vi "CW-main.vi"() -> ()   [LabVIEW 2024]
doc: "Main VI for HFEPR measurements in Field domain.\nProgram uses a tab control that divides user interface in 5 pages. First (status) page is to monitor status of instruments. Second (adjustment) page is to setup individual parameters of each instrument. Third (EPR measurement) page serves for execution of measurement. Fourth (script) page serves for generation of script that can be later loaded in measurement tab. Fifth (measurement review) page is to display previous measurements. The last (about) page contains quick start info for user."
uses:
  Datatypes/Connected modules.ctl
  Datatypes/Magnet controls.ctl
  Datatypes/Servo controls.ctl
  Datatypes/THz parameters.ctl
  Datatypes/Measurement info.ctl
  Datatypes/experiment state.ctl
  Datatypes/SampleHolders.ctl
  Datatypes/Module selection.ctl
  Subsystem modules/Lock-in module/ctl/MFLI parameters.ctl
  Subsystem modules/Temperature control module/ctl/Set temperature.ctl
  Datatypes/script polymorh line.ctl
  Datatypes/Instr Info.ctl
  Subsystem modules/Magnet module/ctl/RampingOutput.ctl
  Datatypes/Single servo status.ctl
  Subsystem modules/Servo drive module/ctl/Axis names.ctl
  Datatypes/Measurement type.ctl
  Datatypes/Rotator controls.ctl
  Subsystem modules/Sample rotator/ctl/Motion Properties.ctl
  Subsystem modules/Sample rotator/ctl/Positoin to set.ctl
  Subsystem modules/Source meter/ctls/SMU settings.ctl
  Datatypes/TopStates.ctl
  Datatypes/XY measurement graph data.ctl
  Datatypes/Measurement mode.ctl
  <vilib>/Utility/sysdir.llb/System Directory Type.ctl
  Subsystem modules/Magnet module/ctl/MSG to magnet.ctl
  Subsystem modules/Magnet module/ctl/Magnet Orders.ctl
  Subsystem modules/Magnet module/ctl/SetField data.ctl
  Subsystem modules/Magnet module/ctl/Magnet mode public.ctl
  Subsystem modules/Servo drive module/ctl/Servo MSG.ctl
  Subsystem modules/Servo drive module/ctl/Servo commands.ctl
  Subsystem modules/Sample rotator/ctl/MSG to Rotator.ctl
  Subsystem modules/Sample rotator/ctl/Rotator commands.ctl
  Subsystem modules/THz module/ctl/THz Message for module.ctl
  Subsystem modules/THz module/ctl/THz commands enum.ctl
  Subsystem modules/THz module/ctl/THz sweep parameters.ctl
  Subsystem modules/Lock-in module/ctl/MFLI_message for module.ctl
  Subsystem modules/Lock-in module/ctl/MFLI_command enum.ctl
  Subsystem modules/Lock-in module/ctl/MFLI_parameter and value.ctl
  Subsystem modules/Lock-in module/ctl/MFLI_node.ctl
  Subsystem modules/Temperature control module/ctl/MSG for VTI.ctl
  Subsystem modules/Temperature control module/ctl/TC commands.ctl
  Subsystem modules/Temperature control module/ctl/Set point.ctl
  Subsystem modules/Source meter/ctls/MSG to SMU.ctl
  Subsystem modules/Source meter/ctls/SMU Commands.ctl
  Subsystem modules/THz module/ctl/THz MW generator constants.ctl
  Subsystem modules/Magnet module/ctl/TM Revision.ctl
  Subsystem modules/Magnet module/ctl/Overall status.ctl
  Subsystem modules/Magnet module/ctl/Actual magnet state.ctl
  Subsystem modules/Magnet module/ctl/Magnet mode.ctl
  Subsystem modules/Magnet module/ctl/Cryostat temperature sensors.ctl
  Subsystem modules/Power monitor/PwrM status.ctl
  Subsystem modules/Source meter/ctls/SMU status.ctl
  Subsystem modules/Lock-in module/ctl/ACQ info.ctl
  <instrlib>/Zurich Instruments LabOne/Public/Data/ziTypeDemodSampleSingle.ctl
  <instrlib>/Zurich Instruments LabOne/Public/ziTypeHandle.ctl
  Subsystem modules/Temperature control module/ctl/TC sensors.ctl
  Subsystem modules/Servo drive module/ctl/Servo state.ctl
  Subsystem modules/Servo drive module/ctl/Servo variables.ctl
  Subsystem modules/Servo drive module/ctl/Servo constants.ctl
  Subsystem modules/Servo drive module/ctl/Status variable change.ctl
  Subsystem modules/Sample rotator/ctl/Rotator all.ctl
  Subsystem modules/Sample rotator/ctl/Axis status.ctl
  <vilib>/Utility/error.llb/Trim Whitespace One-Sided.vi
  Subsystem modules/Messenger service/MessengerLib.lvlib
  Subsystem modules/Magnet module/Magnet module.lvlib
  Subsystem modules/Servo drive module/Servo drive module.lvlib
  Subsystem modules/THz module/THz source modeule.lvlib
  Subsystem modules/Lock-in module/Lock-in module.lvlib
  Subsystem modules/Sample rotator/SampleRotator.lvlib
  <instrlib>/Zurich Instruments LabOne/Zurich Instruments LabOne.lvlib
  Subsystem modules/Temperature control module/Temperature controller.lvlib
  <userlib>/_OpenG.lib/variantconfig/variantconfig.llb/openg_variant_configuration_file.lvlib
  <vilib>/Utility/config.llb/NI_LVConfig.lvlib
  Subsystem modules/Source meter/Source meter.lvlib
  Subsystem modules/Power monitor/Power monitor.lvlib
panel:
  out "Instr status":T1 caption="Connected\ninstuments"
  out "Controls referencies":T2
  out "Tmp [K]":T3
  out "Busy":bool
  in  "Stop":bool
  out "Results":T5(array[cluster])
  out "Magnetic\nfield state":bool
  out "data time":timestamp
  out "New data":bool
  out "Data":dbl[](array[numeric])
  out "Instr control refs":refnum<vi>[](array[refnum])
  out "meas results":refnum<file>
  out "Tmp reched time":dbl format="%<%H:%M:%S>T"
  out "VTI tmp reached":bool
  out "Running experiment":bool
  out "Temperature log ref":refnum<file>
  out "round execution\ntime [ms]":u32
  out "loggersRef":refnum<file>
  in  "Tab Control":T6(tab)
  out "Drift[K/s]":dbl[](array[numeric])
  in  "Log folder":path=path "C:/HFEPR logs"
  in  "Disconnect":bool
  in  "Select module":T7
  out "Logger":string[](array[string])
  in  "Re-connect instruments":bool
  in  "System config file path":path=path "C:/Programs/Debug/HFEPR spectrometer SW 2024/Multi-HFEPR app/SystemData/config.ini"
  out "Instr info":T8 {"PwrMonitor"."Last update" format="%<%H:%M:%S>T"; "VTI"."Last update" format="%<%H:%M:%S>T"; "PMD"."Last update" format="%<%H:%M:%S>T"; "SMU"."Last update" format="%<%H:%M:%S>T"; "Servo"."Last update" format="%<%H:%M:%S>T"; "Rotator"."Actuator" items=["Linear", "Roatator", "Goniometer"]; "Rotator"."Name" items=["ANC350res", "ANC350num", "ANC350fps", "Unknown"]; "Rotator"."Last update" format="%<%H:%M:%S>T"; "THz"."Last update" format="%<%H:%M:%S>T"; "MFLI"."Last update" format="%<%H:%M:%S>T"; "Magnet"."Last update" format="%<%H:%M:%S>T"}
  in  "Use previous settings":bool=TRUE
  out "Temperature monitor":T12(graph)
  in  "Debug mode?":bool=TRUE
  in  "SMU controls":T14={"Apply"=FALSE, "Measurement settings"={"Source Mode "=1, "Source Level"=0.1, "Source Limit"=0.21, "Measure Function"=0, "Remote sense"=TRUE, "Clear buffer?"=FALSE, "Beep"=TRUE, "High Capacity"=TRUE, "Terminals"=1, "PLCs"=4.0, "Fast measurement"=TRUE}, "Value"=0.1006, "Stop"=FALSE, "Record"=FALSE, "B[T]"=0.0, "Refresh"=FALSE} {"Value" format="%#_3e"; "Measurement settings"."Measure Function" items=["Volts", "Current", "Auto Resistance", "Manual Resistance", "Digitize Voltage", "Digitize Current"]; "Measurement settings"."Source Level" max=0.3; "Measurement settings"."Source Mode" items=["Voltage", "Current"]; "Measurement settings"."Terminals" items=["Front", "Rear"]}
  in  "Rotator controls":T15={"Motion properties"={"Frequency [Hz]"=1000.0, "Precision [m°]"=100.0, "DC voltage [V]"=0.0, "Amplitude [V]"=25.0}, "Set position"={"Relative?"=FALSE, "Position [°]"=0.0, "Safe to move?"=FALSE}, "Actual angle[°]"=0.0, "Rot set properties btn"=FALSE, "Rot set position btn"=FALSE, "Stop btn"=FALSE, "EoF"=FALSE, "EoB"=FALSE, "Error"=FALSE} {"Motion properties"."Amplitude [V]" min=0.0 max=60.0; "Motion properties"."DC voltage [V]" min=0.0 max=60.0; "Motion properties"."Precision [m°]" min=1.0 max=1000.0; "Motion properties"."Frequency [Hz]" min=10.0 max=5000.0 step=1.0}
  in  "Password":string
  in  "VTI control":T18={"VTI space [K]"=1.0, "Sample [K]"=0.0, "Heater3 [K]"=1.8, "Heater4 [K]"=1.8, "Out 1 [%]"=0.0, "Out 2 [%]"=0.0, "Range out 1"=0} {"Range out 1" items=["Off", "Range 1 (On)", "Range 2", "Range 3", "Range 4", "Range 5"]; "Heater4 [K]" min=1.8 max=300.0; "Heater3 [K]" min=1.8 max=300.0}
  in  "Acquisition controls":T21={"ACQ parameters"={"Filter order"=7.0, "Filter tau [ms]"=10.0, "F_Mod [kHz]"=1.0, "Amp_Mod [mV]"=10.0, "Enable output"=0, "Phase [°]"=0.0}, "ACQ shot btn"=FALSE, "Modulation [A]"=0.0, "In50"=FALSE, "Out50"=FALSE, "DemEn"=FALSE, "Actual [G]"=0.0, "Sample holder"=enum."Simple", "Desired [G]"=0.0, "Adj mod"=FALSE, "Auto-modulation"=TRUE, "Autorange"=FALSE, "AuxIn0 [V]"=0.0, "AuxIn1 [V]"=0.0} {"AuxIn1 [V]" format="%#_3g"; "AuxIn0 [V]" format="%#_3g"; "Desired [G]" format="%.1g"; "ACQ parameters"."Enable output" items=["Disable", "Enable"]; "ACQ parameters"."Amp_Mod [mV]" min=0.0 max=10000.0; "ACQ parameters"."F_Mod [kHz]" min=0.1 max=500.0; "ACQ parameters"."Filter order" min=1.0 max=9.0 step=1.0; "ACQ parameters"."Filter tau [ms]" min=0.0 max=1000.0}
  in  "THz control":T22={"AMC"=9, "Multip"=1, "Base frequency [GHz]"=82.0, "End frequency [GHz]"=0.0, "Im frequency [MHz]"=1500.0, "Sweep up [ms]"=0.0, "Reset trigger?"=FALSE} {"Multip" items=["1"=1, "2"=2, "3"=3, "4"=4, "6"=6, "8"=8, "9"=9]; "AMC" items=["9"=9, "12"=12]; "End frequency [GHz]" min=0.09 max=126.0; "Base frequency [GHz]" min=0.09 max=126.0 step=0.001 format="%.2g"}
  in  "Servo controls":T23={"Y left"=FALSE, "Y right"=FALSE, "X backward"=FALSE, "X forward"=FALSE, "Zdown"=FALSE, "Zup"=FALSE, "Step\n[mm]"=5.0, "QO table"={"ZLdown"=FALSE, "ZLup"=FALSE, "ZRup"=FALSE, "ZRdown"=FALSE, "ZMdown"=FALSE, "ZMup"=FALSE}, "X"=0.0, "Y"=0.0, "ZL"=0.0, "ZR"=0.0, "ZM"=0.0, "Measure Position btn"=FALSE, "Eject position btn"=FALSE, "Stop servo btn"=FALSE, "Save position btn"=FALSE} {"Step\n[mm]" min=0.0 max=10.0 step=0.25}
  in  "Magnet controls":T24 {"Actual\noutput [T]" scale=0.0..16.0; "Actual\nfield [T]" scale=0.0..16.0; "Desired\nramp [mT/s]" max=7.544966; "Set Field [T]" max=16.0}
  out "lookup":cluster{"X (Vrms)":dbl, "Y (Vrms)":dbl}(graph) caption="Waveform Chart - Dark"
  in  "Create folder with date":bool
  in  "Operator":string
  in  "Hide script":bool
  in  "Save also backup":bool
  in  "Main data folder":path
  in  "Global comment":string
  in  "Sample name":string="Unknown"
  in  "Run script btn":bool
  in  "Direct stop meas. btn":bool
  out "Infobar":T25 {"Started" format="%<%H:%M:%S>T"; "Remains" format="%<%H:%M:%S>t"}
  out "Spectrum":cluster{dbl[], dbl[]}[](graph) caption="Live spectrum"
  in  "Paste from Editor":bool
  out "Actual measurement":T27={"Start"=nan, "Start Caption"="Start [T]", "End"=0.0, "End Caption"="End [T]", "Sweep"=0.0, "Sweep caption"="Rate [mT/s]", "Constant"=0.0, "Constant caption"="Freq [GHz]", "Mod_F [kHz]"=0.0, "Mod_A [G]"=0.0, "Tau [ms]"=0.0, "Angle [°]"=0.0, "Tmp [K]"=50.0, "Wait [min]"=0.0, "Carousel"=-1, "Comment"="", "Auto-mod"=TRUE, "Execute"=FALSE} {"Carousel" items=["0", "1", "2", "3", "4", "5", "6"]; "Angle [°]" min=0.0 max=350.0; "Tau [ms]" min=0.0 max=100.0; "Wait [min]" min=0.0 max=350.0; "Tmp [K]" min=0.0 max=3000.0; "Mod_A [G]" min=0.1 max=150.0; "Mod_F [kHz]" min=0.1 max=150.0}
  in  "Script Array":T27[](array[typedef]) {"Carousel" items=["0", "1", "2", "3", "4", "5", "6"]; "Angle [°]" min=-1.0 max=330.0; "Tau [ms]" min=0.002 max=10000.0; "Wait [min]" min=0.0 max=3000.0; "Tmp [K]" min=0.0 max=350.0; "Mod_A [G]" min=0.0 max=100.0; "Mod_F [kHz]" min=0.1 max=150.0}
  in  "Generator options":T28={"Tmp step [K]"=0.0, "Angle step [°]"=0.0, "Freq step [GHz]"=0.0, "Append"=TRUE, "Iterate"=0}
  in  "Clear script btn":bool caption="Clear all script"
  in  "Set as adj tab btn":bool caption="Apply settings from\nadjustment tab"
  in  "Prototype line":T27={"Start"=0.0, "Start Caption"="Start [T]", "End"=0.0, "End Caption"="End [T]", "Sweep"=3.0, "Sweep caption"="Rate [mT/s]", "Constant"=210.0, "Constant caption"="Freq [GHz]", "Mod_F [kHz]"=69.1, "Mod_A [G]"=2.0, "Tau [ms]"=100.0, "Angle [°]"=-1.0, "Tmp [K]"=2.0, "Wait [min]"=0.1, "Carousel"=0, "Comment"="No comment", "Auto-mod"=TRUE, "Execute"=FALSE} {"Carousel" items=["0", "1", "2", "3", "4", "5", "6"]; "Angle [°]" min=-1.0 max=330.0; "Tau [ms]" min=0.002 max=10000.0; "Wait [min]" min=0.0 max=3000.0; "Tmp [K]" min=0.0 max=350.0; "Mod_A [G]" min=0.0 max=100.0; "Mod_F [kHz]" min=0.1 max=150.0}
  in  "Paste from meeasurrement":bool
  in  "Save script file btn":bool
  in  "Generate Script btn":bool caption="Generate Script"
  in  "Edited script":T27[](array[typedef]) caption="Script file name:" {"Carousel" items=["0", "1", "2", "3", "4", "5", "6"]; "Angle [°]" min=-1.0 max=330.0; "Tau [ms]" min=0.002 max=10000.0; "Wait [min]" min=0.0 max=3000.0; "Tmp [K]" min=0.0 max=350.0; "Mod_A [G]" min=0.0 max=100.0; "Mod_F [kHz]" min=0.1 max=150.0}
  in  "Remove from script btn":bool
  in  "Load script btn":bool
  in  "Select\nline":i32 min=-8 max=7
  in  "Save data btn":bool
  in  "Shift data btn":bool
  in  "Edit Channel":bool
  in  "Amlitude shift [-]":dbl
  in  "From point [T]":dbl
  out "Header":string[](array[string])
  out "Review Graph":cluster{"Array":dbl[], "Array":dbl[]}[](graph) caption="Header"
  in  "Open measurement":bool
  in  "Data file to show":u16(ring) items=["Empty", "Empty", "Empty", "Empty", "Empty", "Empty", "Empty", "Empty", "Empty", "Empty"]
  in  "Quick guide":T29(tab)
  # "Status part"
  # "Action part"
  # "stop after this line button"
  # "Option 1:\nchoice primary and secondary sweep\n\nOption 2:\nChoice measurement mode, and appropriate cluster will apear. Other clusters wil be hidden.\n\n\nOption 3:\nChoice measurement mode.\nInternal parts of single cluster will (dis)apear if needed.\n\nNote:\nPosibility to do an orientation/temperature deppendency."
  # "Tmp [K]"
  # "Position [mm]"
  # "Z"
  # "X/Y"
  # "This software was developed for HFEPR spectrometer in 2019 (2020) at CEITEC BUT by members of MOTES research group.\n\nQuick guide:\n1) Re-connect to all instruments.\n2) Check if necessary instruments are ready. (At least VTI, VDI, Lock-In, and Magnet has to work)\n3) Go to Adjustment tab and set up Lock-in parameters as well as VDI multipiers.\n4) Go to EPR measurement tab, select folder path, fill the sample description.\n5) Fill at least 1 line of the script and press Run script button.\n\n6) In case of a bug please report this to software developer or make a note into developement diary loaceted at:\n    RG-1-12/Instriments/HFEPR spectrometer/Software developement.\n\nLast update: 07.02. 2020 - Script editor is working, measurement review not yet.\n\nSpecial thanks to: Luke Skywalker, my mom, Tonda's mom, Pilsner, God, Oleksi, Vinicius, Petr from parallel universe.\n\n \nTODO: Invisible controls: referencies for: adjustment controls, meas results, loggerRef,"
  # "1.\tSelect module for subsystem, which is ready to operate. For CW measurements it is necessary to use subsystems: Magnet, VTI,\n THz sources and data acquisition (MFLI).\n2.\tClick on (Re)Connect button. Repeat for all subsystems that are ready and needed.\n3.\tWhen VTI and Magnet subsystems are connected, readings from temperature monitor and controller are displayed in graph.\n4.\tSuccessful connection to subsystem is indicated here.\n5.\tEvents on instruments are reported in this indicator.\n6.\tIf everything is OK, user may continue to another tab."
  # "1.\tFor CW experiments, magnet has to be in  ramping mode. (Magnet can be then pre-set to a start field.)\n2.\tCorrect multiplication factor need to be set manually by user.\n3.\tIntermediate frequency need to be set in in a middle of the range of band pass filters. \n4.\tTemperature of VTI can be also pre-set, while other settings are done (2 - 325 K).\n5.\tPosition of table in X axis should be about 900 mm. If table is not in measurement position, and there is no object in way, user can click on button Measure.\n6.\tIn control cluster for MFLI it is needed to enable output and set reasonable frequency and amplitude of modulation. After that click on Auto range button.\n7.\tIn case when sample rotator is used, user can check if rotator works correctly by setting desired position and press Go button.\n8.\tIn case when field sensor is used, it is required to setup current source, 100 mA, measure voltage, remote sense, rear terminals and press Apply button.\n9.\tIf series of measurement is going to be done, it is recommended to first setup measurement script in a script editor."
  # "1.\tLoad script from the Script editor tab. (overwrites current script in this tab)\n2.\tModify script if needed.\n3.\tSelect main folder, where data will be stored.\n4.\tFill name of a sample and operator that will be included in a file name.\n5.\tIf checked, save data in subfolder.\n6.\tTextbox for user to add any comment in header of data file.\n7.\tStart sequence of measurements in the script.\n8.\tContain brief information about measurement process.\n9.\tDisplays a raw spectrum.\n10.\tStop whole sequence.\n11.\tA standard graph tools."
  # "1.\tLoad actual settings of instruments and apply them to a prototype line.\n2.\tModify prototype line if needed.\n3.\tSet step for one (or more) parameter, and number of iterations.\n4.\tIf checked, append to a current scrip; else, overwrites.\n5.\tSave current script into text file (structured as configuration file) to load it later.\n6.\tModify generated script or manually fill a next line."
  # "1.\tLoad data from a file.\n2.\tRing for switching to previously loaded data.\n3.\tStandard graph tools (zoom, cursor).\n4.\tFeature to apply a simple data correction."
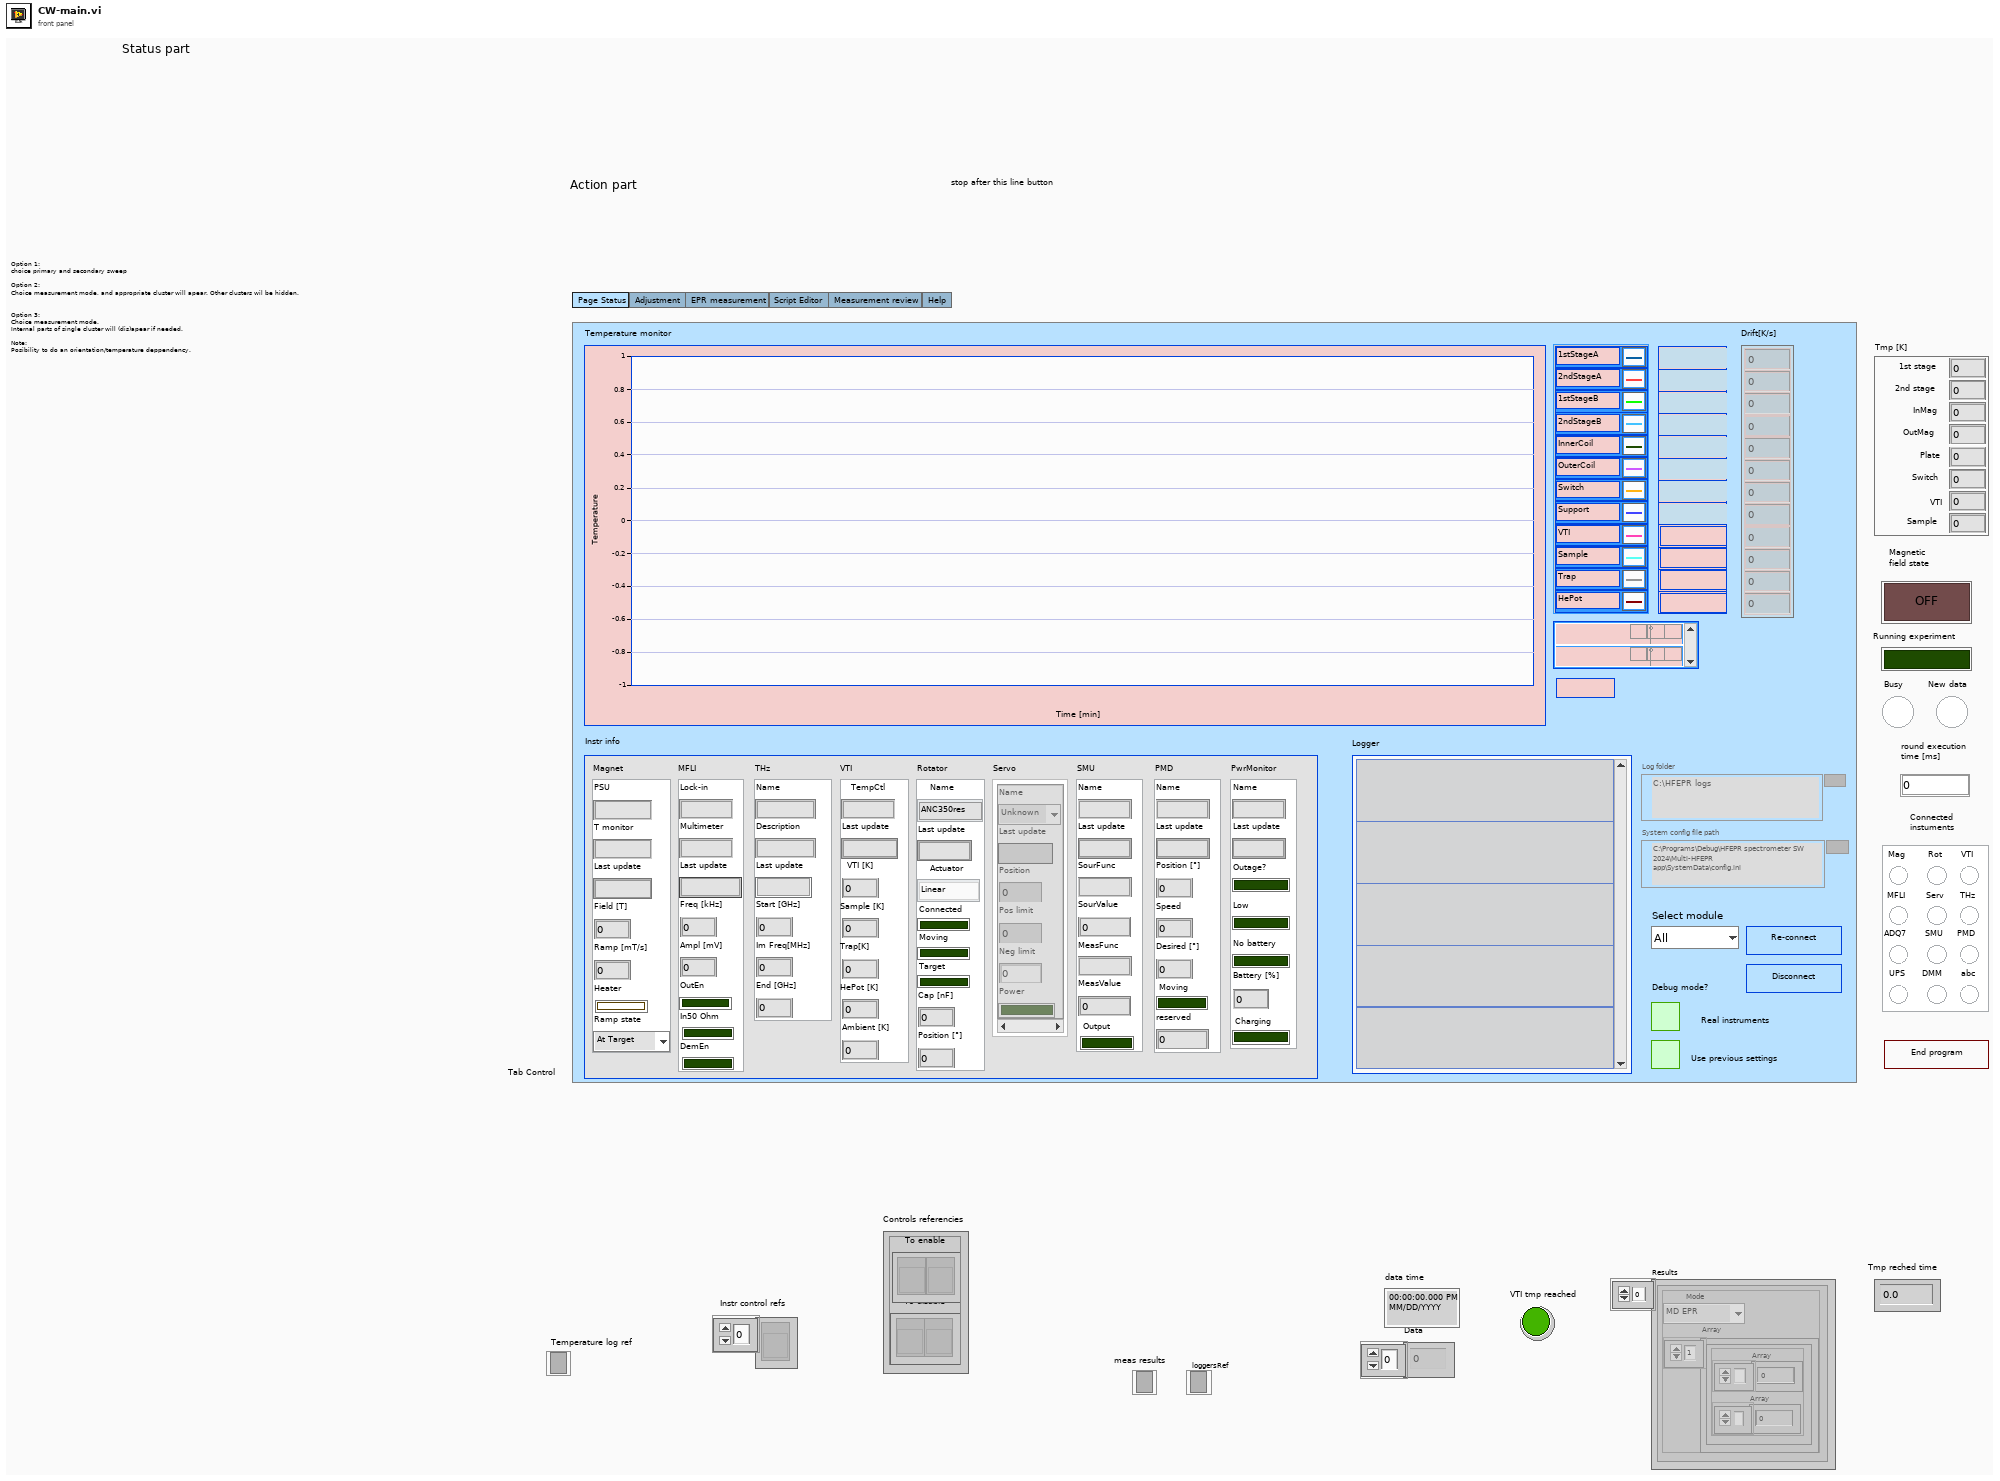
[diagram p1: front panel]
types:
  T1 = typedef "Connected modules.ctl" = cluster{"Mag":bool, "Rot":bool, "VTI":bool, "MFLI":bool, "Serv":bool, "THz":bool, "ADQ7":bool, "SMU":bool, "PMD":bool, "UPS":bool, "DMM":bool, "abc":bool}
  T2 = cluster{"To disable":refnum<vi>[], "To enable":refnum<vi>[]}
  T3 = cluster{"1st stage":dbl, "2nd stage":dbl, "InMag":dbl, "OutMag":dbl, "Plate":dbl, "Switch":dbl, "VTI":dbl, "Sample":dbl}
  T4 = typedef "Measurement type.ctl" = enum16{"MD EPR", "FD EPR"}
  T5 = cluster{"Mode":T4, "Array":cluster{"Array":dbl[], "Array":dbl[]}[]}[]
  T6 = enum32{"Page Status", "Adjustment", "EPR measurement", "Script Editor", "Measurement review", "Help"}
  T7 = typedef "Module selection.ctl" = enum16{"All", "None", "ACQ", "THz", "MAG", "SERV", "ROT", "VTI", "SMU", "ADQ7", "PMD"}
  T8 = typedef "Instr Info.ctl" = cluster{"Magnet":cluster{"PSU":string, "T monitor":string, "Last update":timestamp, "Field [T]":dbl, "Ramp [mT/s]":dbl, "Heater":bool, "Ramp state":T9}, "MFLI":cluster{"Lock-in":string, "Multimeter":string, "Last update":timestamp, "Freq [kHz]":dbl, "Ampl [mV]":dbl, "OutEn":bool, "In50 Ohm":bool, "DemEn":bool}, "THz":cluster{"Name":string, "Description":string, "Last update":timestamp, "Start [GHz]":dbl, "Im Freq[MHz]":dbl, "End [GHz]":dbl}, "VTI":cluster{"TempCtl":string, "Last update":timestamp, "VTI [K]":dbl, "Sample [K]":dbl, "Trap[K]":dbl, "HePot [K]":dbl, "Ambient [K]":dbl}, "Rotator":cluster{"Name":u16, "Last update":timestamp, "Actuator":u16, "Connected":bool, "Moving":bool, "Target":bool, "Cap [nF]":dbl, "Position [°]":dbl}, "Servo":T10[], "SMU":cluster{"Name":string, "Last update":timestamp, "SourFunc":string, "SourValue":dbl, "MeasFunc":string, "MeasValue":dbl, "Output":bool}, "PMD":cluster{"Name":string, "Last update":timestamp, "Position [°]":dbl, "Speed":dbl, "Desired [°]":dbl, "Moving":bool, "reserved":dbl}, "PwrMonitor":cluster{"Name":string, "Last update":timestamp, "Outage?":bool, "Low":bool, "No battery":bool, "Battery [%]":u8, "Charging":bool}}
  T9 = typedef "Magnet module.lvlib/RampingOutput.ctl" = enum16{"At Target", "Go up", "Go down"}
  T10 = typedef "Single servo status.ctl" = cluster{"Name":T11, "Last update":timestamp, "Position":dbl, "Pos limit":dbl, "Neg limit":dbl, "Power":bool}
  T11 = typedef "Servo drive module.lvlib/Axis names.ctl" = enum16{"Unknown", "AxisX", "AxisY", "AxisZ_left", "AxisZ_middle", "AxisZ_right"}
  T12 = cluster{"[0]":dbl, "[1]":dbl, "[2]":dbl, "[3]":dbl, "[4]":dbl, "[5]":dbl, "[6]":dbl, "[7]":dbl, "[8]":dbl, "[9]":dbl, "[10]":dbl, "[11]":dbl}
  T13 = typedef "SMU settings.ctl" = cluster{"Source Mode ":u16, "Source Level":dbl, "Source Limit":dbl, "Measure Function":u16, "Remote sense":bool, "Clear buffer?":bool, "Beep":bool, "High Capacity":bool, "Terminals":u16, "PLCs":dbl, "Fast measurement":bool}
  T14 = cluster{"Apply":bool, "Measurement settings":T13, "Value":dbl, "Stop":bool, "Record":bool, "B[T]":dbl, "Refresh":bool}
  T15 = typedef "Rotator controls.ctl" = cluster{"Motion properties":T16, "Set position":T17, "Actual angle[°]":dbl, "Rot set properties btn":bool, "Rot set position btn":bool, "Stop btn":bool, "EoF":bool, "EoB":bool, "Error":bool}
  T16 = typedef "Motion Properties.ctl" = cluster{"Frequency [Hz]":dbl, "Precision [m°]":dbl, "DC voltage [V]":dbl, "Amplitude [V]":dbl}
  T17 = typedef "Positoin to set.ctl" = cluster{"Relative?":bool, "Position [°]":dbl, "Safe to move?":bool}
  T18 = typedef "Temperature controller.lvlib/Set temperature.ctl" = cluster{"VTI space [K]":dbl, "Sample [K]":dbl, "Heater3 [K]":dbl, "Heater4 [K]":dbl, "Out 1 [%]":dbl, "Out 2 [%]":dbl, "Range out 1":u16}
  T19 = typedef "Lock-in module.lvlib/MFLI parameters.ctl" = cluster{"Filter order":dbl, "Filter tau [ms]":dbl, "F_Mod [kHz]":dbl, "Amp_Mod [mV]":dbl, "Enable output":u16, "Phase [°]":dbl}
  T20 = typedef "SampleHolders.ctl" = enum16{"Simple", "Carousel", "Chip", "Rotator", "Liquid"}
  T21 = cluster{"ACQ parameters":T19, "ACQ shot btn":bool, "Modulation [A]":dbl, "In50":bool, "Out50":bool, "DemEn":bool, "Actual [G]":dbl, "Sample holder":T20, "Desired [G]":dbl, "Adj mod":bool, "Auto-modulation":bool, "Autorange":bool, "AuxIn0 [V]":dbl, "AuxIn1 [V]":dbl}
  T22 = typedef "THz parameters.ctl" = cluster{"AMC":u16, "Multip":u16, "Base frequency [GHz]":dbl, "End frequency [GHz]":dbl, "Im frequency [MHz]":dbl, "Sweep up [ms]":dbl, "Reset trigger?":bool}
  T23 = typedef "Servo controls.ctl" = cluster{"Y left":bool, "Y right":bool, "X backward":bool, "X forward":bool, "Zdown":bool, "Zup":bool, "Step\n[mm]":dbl, "QO table":cluster{"ZLdown":bool, "ZLup":bool, "ZRup":bool, "ZRdown":bool, "ZMdown":bool, "ZMup":bool}, "X":dbl, "Y":dbl, "ZL":dbl, "ZR":dbl, "ZM":dbl, "Measure Position btn":bool, "Eject position btn":bool, "Stop servo btn":bool, "Save position btn":bool}
  T24 = typedef "Magnet controls.ctl" = cluster{"Set Field [T]":dbl, "Desired\nramp [mT/s]":dbl, "Custom\nramp":bool, "Mode switch":bool, "Pause ramp":bool, "Actual\nfield [T]":dbl, "Actual\noutput [T]":dbl, "Equalize":bool, "Discharge":bool, "Switch tmp [K]":dbl, "Direction":bool}
  T25 = typedef "Measurement info.ctl" = cluster{"Remains":dbl, "T_sample [K]":dbl, "Last log":string, "Experiment state":T26, "Field [T]":dbl, "Sample holder":T20, "Started":timestamp}
  T26 = typedef "experiment state.ctl" = enum16{"Setup", "Preparation", "Stabilization", "Begin", "Acquisition", "Save"}
  T27 = typedef "script polymorh line.ctl" = cluster{"Start":dbl, "Start Caption":string, "End":dbl, "End Caption":string, "Sweep":dbl, "Sweep caption":string, "Constant":dbl, "Constant caption":string, "Mod_F [kHz]":dbl, "Mod_A [G]":dbl, "Tau [ms]":dbl, "Angle [°]":dbl, "Tmp [K]":dbl, "Wait [min]":dbl, "Carousel":i8, "Comment":string, "Auto-mod":bool, "Execute":bool}
  T28 = cluster{"Tmp step [K]":dbl, "Angle step [°]":dbl, "Freq step [GHz]":dbl, "Append":bool, "Iterate":u16}
  T29 = enum32{"Status", "Adjustment", "Measurement", "Script", "Viewer"}
  T30 = typedef "TopStates.ctl" = enum16{"Initialize GUI", "Wait for Event", "Check message", "Check measurement", "Stop", "Restart"}
  T31 = typedef "MessengerLib.lvlib/Messenger referencies.ctl" = cluster{"TOP":refnum<queue>, "Instr_M":refnum<queue>, "Field_C":refnum<queue>, "Tmp_M":refnum<queue>, "Tmp_C":refnum<queue>, "Table_C":refnum<queue>, "MW_C":refnum<queue>, "Data_Aq":refnum<queue>, "Mod_M":refnum<queue>, "Field_M":refnum<queue>, "Pwr_M":refnum<queue>, "Angle_C":refnum<queue>, "Sample_C":refnum<queue>, "Reserved":refnum<queue>}
  T32 = typedef "XY measurement graph data.ctl" = cluster{"Mode":T33, "Array":cluster{"Array":dbl[], "Array":dbl[]}[]}
  T33 = typedef "Measurement mode.ctl" = enum16{"MD EPR", "FD EPR", "EDMR", "EPR MAP"}
  T34 = enum8{"Enabled", "Disabled", "Disabled and Grayed Out"}
  T35 = typedef "Magnet module.lvlib/Magnet mode public.ctl" = enum16{"Persistant", "Ramping"}
  T36 = typedef "Magnet module.lvlib/SetField data.ctl" = cluster{"Field [T]":dbl, "Ramp [T/s]":dbl, "Custom Ramp?":bool, "Mode":T35}
  T37 = typedef "Magnet module.lvlib/Magnet Orders.ctl" = enum16{"Ignore", "Connect", "Update", "Switch mode", "Set field", "Stop ramping", "Equalize output", "Zero output", "Flip polarity", "Blackout", "Set timer", "Eval temperatures", "Disconnect"}
  T38 = typedef "Magnet module.lvlib/MSG to magnet.ctl" = cluster{"Order":T37, "Data":variant}
  T39 = typedef "Servo drive module.lvlib/Servo commands.ctl" = enum16{"Initialize", "Update", "Move by", "Move to", "Stop", "Ignore", "Disconnect", "End"}
  T40 = typedef "Servo drive module.lvlib/Servo MSG.ctl" = cluster{"Command":T39, "Data":variant}
  T41 = typedef "SampleRotator.lvlib/MSG to Rotator.ctl" = cluster{"Command":T42, "Data":variant}
  T42 = typedef "SampleRotator.lvlib/Rotator commands.ctl" = enum16{"Ignore", "Initialize", "Update", "Set parameters", "Stop movement", "Set position", "Disconnect", "End"}
  T43 = typedef "THz source modeule.lvlib/THz commands enum.ctl" = enum16{"Ignore", "Connect", "Update", "Set parameters", "Disconnect", "End"}
  T44 = typedef "THz source modeule.lvlib/THz sweep parameters.ctl" = cluster{"Start [GHz]":dbl, "End [GHz] ":dbl, "Sweep up\ntime [ms]":dbl, "Sweep down\ntime [ms]":dbl, "Intermidiate [MHz]":dbl, "Reset trigger":bool}
  T45 = typedef "THz source modeule.lvlib/THz Message for module.ctl" = cluster{"Command":T43, "Data":variant}
  T46 = typedef "Lock-in module.lvlib/MFLI_parameter and value.ctl" = cluster{"parameter":T47, "value":dbl}
  T47 = typedef "Lock-in module.lvlib/MFLI_node.ctl" = enum16{"None", "filter_order [-]", "filter_constant [ms]", "in_diff", "in_autorange", "in_imp50", "in_AC", "osc_freq [kHz]", "out_ampl [V]", "out_autorange", "out_imp50", "enable output", "enamble ampl", "scope_enable", "scope_rate", "scope_len", "scope_trigEn", "AuxOut_amplify", "Phase_deg", "AuxOut_select"}
  T48 = typedef "Lock-in module.lvlib/MFLI_command enum.ctl" = enum16{"Initialize", "Update", "Set parameters", "Set module", "Set individual parameters", "Get point", "Get array", "Disconnect", "End", "Ignore"}
  T49 = typedef "Lock-in module.lvlib/MFLI_message for module.ctl" = cluster{"Command":T48, "Data":variant}
  T50 = typedef "Temperature controller.lvlib/Set point.ctl" = cluster{"Heater":string, "Tmp [K]":dbl}
  T51 = typedef "Temperature controller.lvlib/TC commands.ctl" = enum16{"Initialize", "Update", "Stop tmp change", "Set temperature", "Set point", "Disconnect", "End", "Ignore"}
  T52 = typedef "Temperature controller.lvlib/MSG for VTI.ctl" = cluster{"Command":T51, "Data":variant}
  T53 = typedef "Source meter.lvlib/MSG to SMU.ctl" = cluster{"Command":T54, "Data":variant}
  T54 = typedef "Source meter.lvlib/SMU Commands.ctl" = enum16{"Ignore", "Connect", "Update", "Set measurement", "Start measurement", "Get actual results", "Stop measurement", "Disconnect", "End"}
  T55 = cluster{"min synth f":dbl, "max synth f":dbl, "Ramp limits [mT/s]":dbl[], "Field ranges [T]":dbl[]}
  T56 = cluster{"Mode":T4, "Array":cluster{"Array":dbl[], "Array":dbl[]}[]}
  T57 = typedef "THz source modeule.lvlib/THz MW generator constants.ctl" = cluster{"Lower limit [GHz]":dbl, "Upper limit [GHz]":dbl, "Device name":string, "Connection":string, "Description":string, "Connected":bool, "Last settings":string, "Operation mode":enum16{"Disabled", "CW", "Arbitrary", "Sweep"}, "Enable ch 1":bool, "Enable ch 2":bool}
  T58 = typedef "Magnet module.lvlib/TM Revision.ctl" = cluster{"Instr Serial Number":string, "Instr Driver Revision":string, "Instr Firmware Revision":string, "Instr Model Number":string}
  T59 = typedef "Magnet module.lvlib/Overall status.ctl" = cluster{"Desired":T36, "Actual":T60}
  T60 = typedef "Magnet module.lvlib/Actual magnet state.ctl" = cluster{"Mode":T61, "Ramping output":T9, "Ready for change":bool, "Switch heater":bool, "Cooler Overheat":bool, "Coil overheat":bool, "Energized":bool, "Output [T]":dbl, "Field [T]":dbl, "Ramp[T/s]":dbl, "Switch\ntemperature [K]":dbl, "Voltage [V]":dbl, "Current direction":bool}
  T61 = typedef "Magnet module.lvlib/Magnet mode.ctl" = enum16{"Persistant", "Switching", "Ramping", "Quenched"}
  T62 = typedef "Magnet module.lvlib/Cryostat temperature sensors.ctl" = cluster{"First stage A [K]":dbl, "Second stage A [K]":dbl, "Firs stage B [K]":dbl, "Second stage B [K]":dbl, "Inner magnet [K]":dbl, "Outer Magnet [K]":dbl, "Switch [K]":dbl, "Support plate [K]":dbl, "Time stamp":dbl}
  T63 = typedef "Power monitor.lvlib/PwrM status.ctl" = cluster{"Name":string, "Last update":timestamp, "Outage?":bool, "Low":bool, "No battery":bool, "Battery [%]":u8, "Charging":bool}
  T64 = typedef "Source meter.lvlib/SMU status.ctl" = cluster{"VISA name":refnum<visa-resource-name>, "Connected":bool, "Name":string, "Message":string, "Error message":string, "Min voltage":dbl, "Max voltage":dbl, "Min Current":dbl, "Max Current":dbl, "Measurement value":dbl, "Source Voltage":dbl, "Measurement":bool, "Source Current":dbl, "Source Mode":u16, "Measure Function":u16}
  T65 = typedef "Lock-in module.lvlib/ACQ info.ctl" = cluster{"In50":bool, "InAC":bool, "InDiff":bool, "Out50":bool, "OutEN":bool, "OutF[Hz]":dbl, "OutA[V]":dbl, "DemEN":bool, "Const[ms]":dbl, "Order[-]":i32, "Phase [°]":dbl}
  T66 = enum32{"Page Status", "Adjustment", "EPR measurement", "About"}
  T67 = typedef "Zurich Instruments LabOne.lvlib/ziTypeDemodSampleSingle.ctl" = cluster{"Timestamps (ticks)":u64, "X (Vrms)":dbl, "Y (Vrms)":dbl, "Osc Phase (deg)":dbl, "Freq (Hz)":dbl, "DIO":u32, "AuxIn0 (V)":dbl, "AuxIn1 (V)":dbl, "Trigger":u32}
  T68 = typedef "Zurich Instruments LabOne.lvlib/ziTypeHandle.ctl" = cluster{"handleValid":bool, "Conn":u64, "Path Prefix":string, "Handle":u64, "Connected":bool, "Clockbase(s)":dbl}
  T69 = typedef "Temperature controller.lvlib/TC sensors.ctl" = cluster{"VTI space":dbl, "Sample":dbl, "He pot":dbl, "Trap":dbl, "Ambient":dbl, "SetP_VTI":dbl, "SetP_Smp":dbl, "SetP_Pot":dbl, "SetP_Trap":dbl, "Range out 1":u16, "Out 1 [%]":dbl, "Out 2 [%]":dbl}
  T70 = typedef "Servo drive module.lvlib/Servo state.ctl" = cluster{"Servo variables":T71, "Servo constants":T72, "Connection":variant}
  T71 = typedef "Servo drive module.lvlib/Servo variables.ctl" = cluster{"Terget reached":bool, "Connected":bool, "Power ON":bool, "Operation mode":bool, "Actual position":dbl, "Target position":dbl}
  T72 = typedef "Servo drive module.lvlib/Servo constants.ctl" = cluster{"Name":T11, "Pos position limit [mm]":dbl, "Neg position limit [mm]":dbl, "Pos velocity limit":dbl, "Neg velocity limit":dbl, "Acceleration limit":dbl}
  T73 = typedef "Servo drive module.lvlib/Status variable change.ctl" = cluster{"Property":string, "Value":variant, "Name":T11}
  T74 = typedef "SampleRotator.lvlib/Rotator all.ctl" = cluster{"Controller info":cluster{"deviceNumber":i32, "DeviceType":i32, "ID":u32, "Serial":string, "Address":string, "connected":bool}, "Handle":u64, "FW-Version":i32, "Features":u32, "ActuatorType":u16, "ActuatorName":string, "Axis info":T75, "Capacitance[uF]":dbl, "Path to DLL":path}
  T75 = typedef "SampleRotator.lvlib/Axis status.ctl" = cluster{"Axis status":cluster{"connected":bool, "enabled":bool, "moving":bool, "target":bool, "EotFwd":bool, "EotBwd":bool, "error":bool}, "Position [°]":dbl, "Freque [Hz]":dbl, "Voltage [V]":dbl}
  T76 = typedef "NI_LVConfig.lvlib/Config Data RefNum.ctl" = refnum<k1>
  T77 = typedef "System Directory Type.ctl" = i32
  T78 = typedef "lveventtype.ctl" = enum32{"Null", "Timeout", "Annotation Menu Selection", "Annotation Menu Selection?", "App Instance Close", "App Instance Close?", "Autoscale Range Change", "Bookmark Info Change", "Cell Edit", "Cell Edit?", "Cursor Grab", "Cursor Grab?", "Cursor Menu Selection", "Cursor Menu Selection?", "Cursor Move", "Cursor Release", "Data Change", "Direction Change", "Display State Change", "Drag Ended", "Drag Enter", "Drag Leave", "Drag Over", "Drag Source Update", "Drag Starting", "Drag Starting?", "Drop", "Exec State Change", "Key Down", "Key Down?", "Key Repeat", "Key Repeat?", "Key Up", "Listbox Double Click", "Menu Activation?", "Menu Selection (App)", "Menu Selection? (App)", "Menu Selection (User)", "Mouse Down", "Mouse Down?", "Mouse Enter", "Mouse Leave", "Mouse Move", "Mouse Up", "Mouse Wheel", "NI Security User Change (App)", "Pane Size", "Panel Close", "Panel Close?", "Panel Resize", "Plot Attribute Change", "Scale Range Change", "Shortcut Menu Activation?", "Shortcut Menu Selection (App)", "Shortcut Menu Selection? (App)", "Shortcut Menu Selection (User)", "Tree Double Click", "Tree Drag", "Tree Drag?", "Tree Drop", "Tree Drop?", "Tree Item Close", "Tree Item Close?", "Tree Item Open", "Tree Item Open?", "User Event", "Value Change"}
  T79 = typedef "Mudules status.ctl" = cluster{"Mag":bool, "Rot":bool, "VTI":bool, "MFLI":bool, "Serv":bool, "THz":bool, "ADQ7":bool, "SMU":bool, "PMD":bool, "UPS":bool, "DMM":bool, "abc":bool}
  T80 = typedef "Magnet module.lvlib/Magnet config constants.ctl" = cluster{"Switch resistant [K]":dbl, "Switch superconducting [K]":dbl, "First stage critical temperature [K]":dbl, "Second stage critical temperature [K]":dbl, "Inner magnet critical temperature [K]":dbl, "Outer magnet critical temperature [K]":dbl, "Field Constant [T/A]":dbl, "Maximum Current [A]":dbl, "Maximum field [T]":dbl, "Maximum source ramp [A/s]":dbl, "Source precision [T]":dbl, "Ramp limits [A/s]":dbl[], "Field limits [T]":dbl[], "SMS":refnum<visa-resource-name>, "LSC218":refnum<visa-resource-name>}
  T81 = typedef "MessengerLib.lvlib/MSG to TOP.ctl" = cluster{"Module":T82, "Response":string, "Data":variant, "Time":timestamp}
  T82 = typedef "Module name.ctl" = enum16{"Emty", "Magnet", "VTI", "Excitation", "Servo", "Acquisition", "Rotator", "Digitizer", "SMU2450", "Carousel", "Multimeter", "Tmp monitor", "Power monitor"}
  T83 = cluster{"PSU":string, "T monitor":string, "Last update":timestamp, "Field [T]":dbl, "Ramp [mT/s]":dbl, "Heater":bool, "Ramp state":T9}
  T84 = cluster{"TempCtl":string, "Last update":timestamp, "VTI [K]":dbl, "Sample [K]":dbl, "Trap[K]":dbl, "HePot [K]":dbl, "Ambient [K]":dbl}
  T85 = cluster{"Name":string, "Description":string, "Last update":timestamp, "Start [GHz]":dbl, "Im Freq[MHz]":dbl, "End [GHz]":dbl}
  T86 = cluster{"Name":string, "Last update":timestamp, "Outage?":bool, "Low":bool, "No battery":bool, "Battery [%]":u8, "Charging":bool}
  T87 = cluster{"Name":string, "Last update":timestamp, "SourFunc":string, "SourValue":dbl, "MeasFunc":string, "MeasValue":dbl, "Output":bool}
  T88 = cluster{"Lock-in":string, "Multimeter":string, "Last update":timestamp, "Freq [kHz]":dbl, "Ampl [mV]":dbl, "OutEn":bool, "In50 Ohm":bool, "DemEn":bool}
  T89 = cluster{"Name":u16, "Last update":timestamp, "Actuator":u16, "Connected":bool, "Moving":bool, "Target":bool, "Cap [nF]":dbl, "Position [°]":dbl}
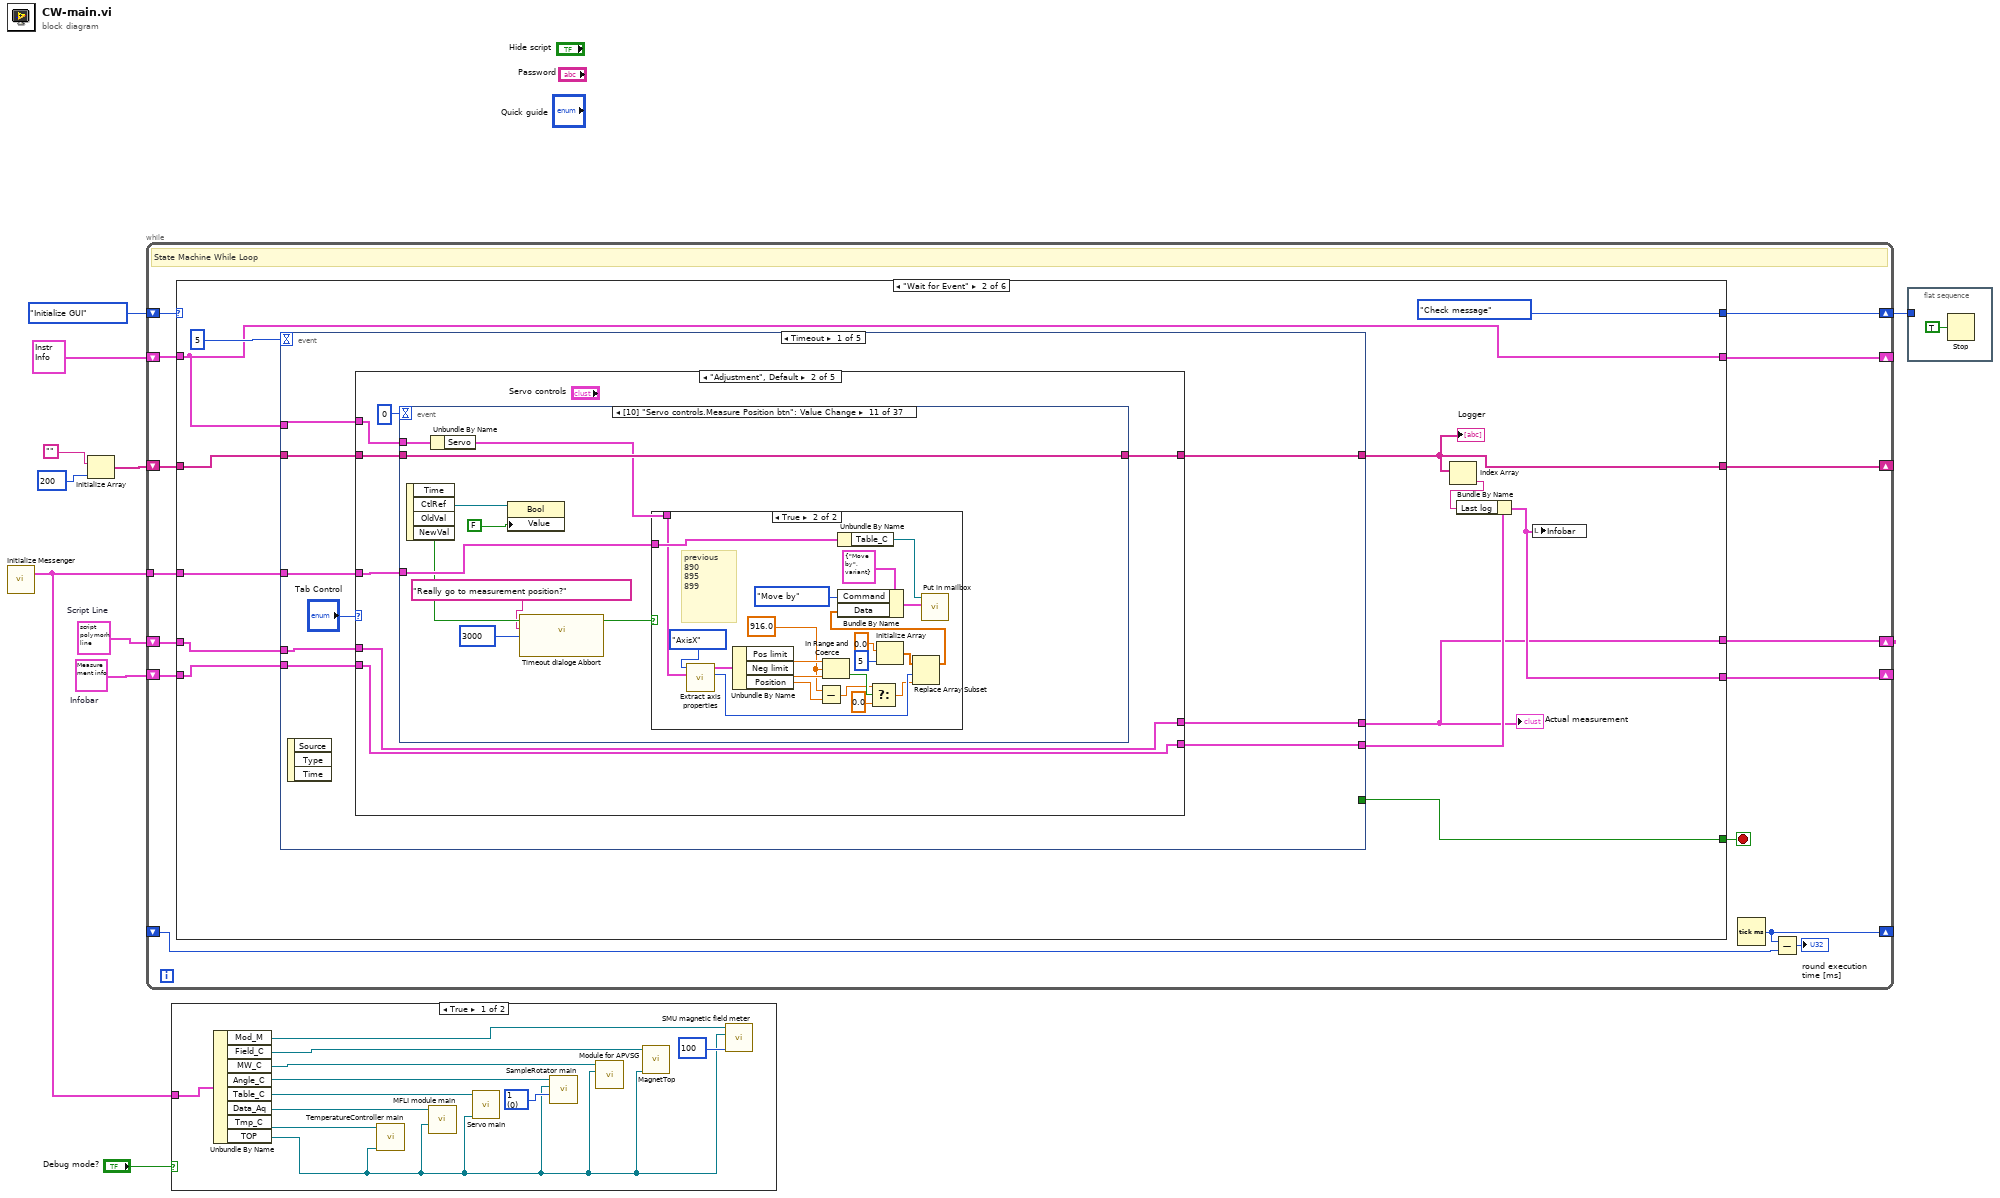
[diagram p0: block diagram]
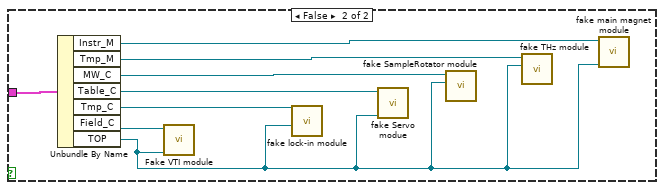
[diagram p2: hidden frame]
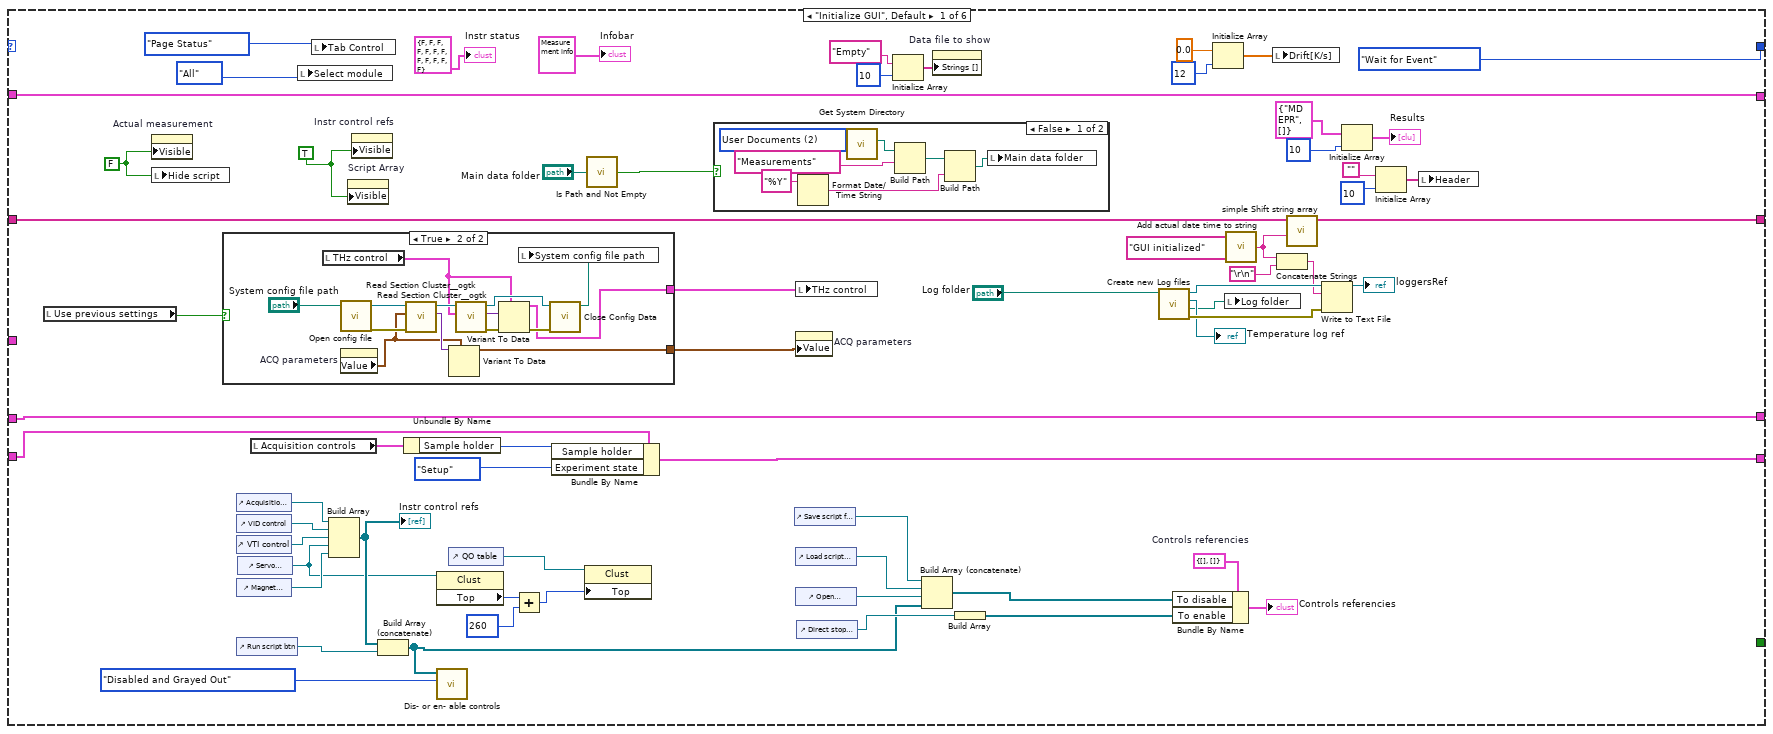
[diagram p3: hidden frame]
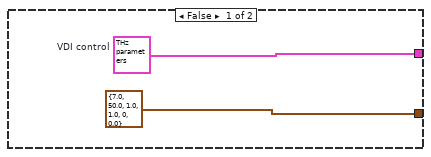
[diagram p5: hidden frame]
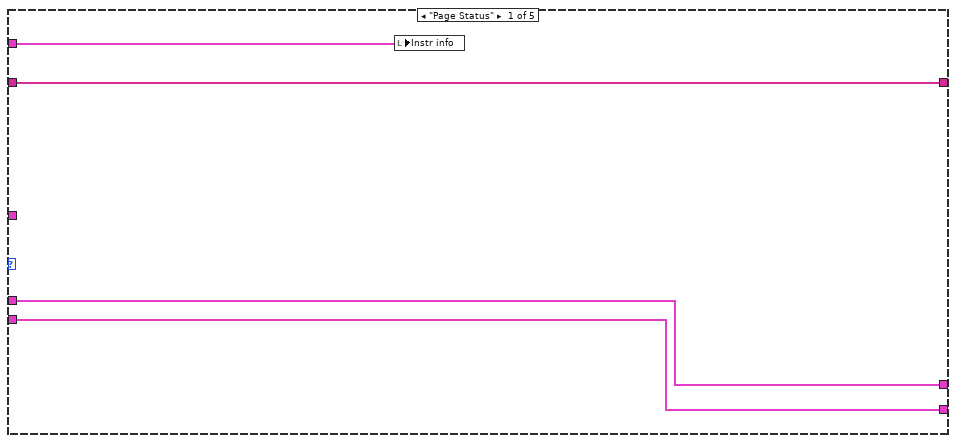
[diagram p6: hidden frame]
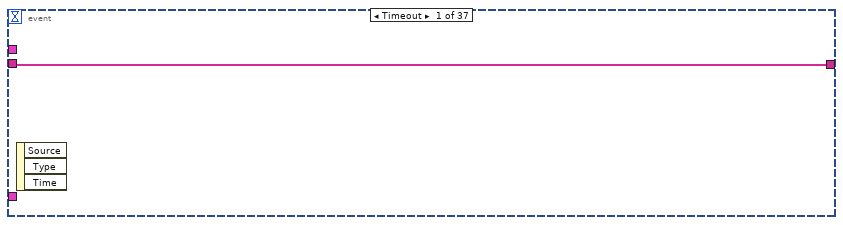
[diagram p7: hidden frame]
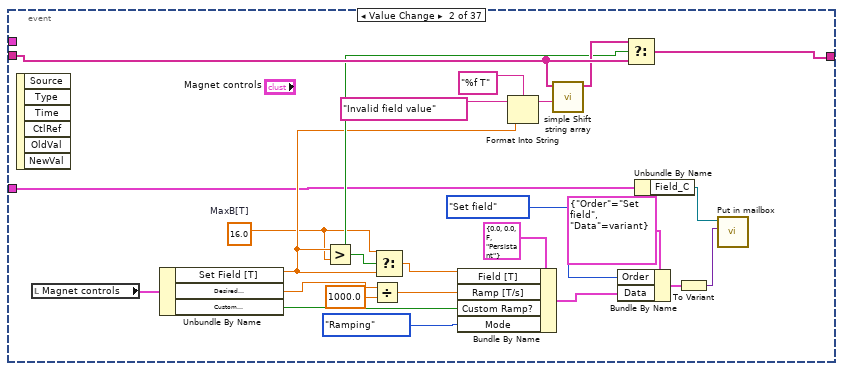
[diagram p8: hidden frame]
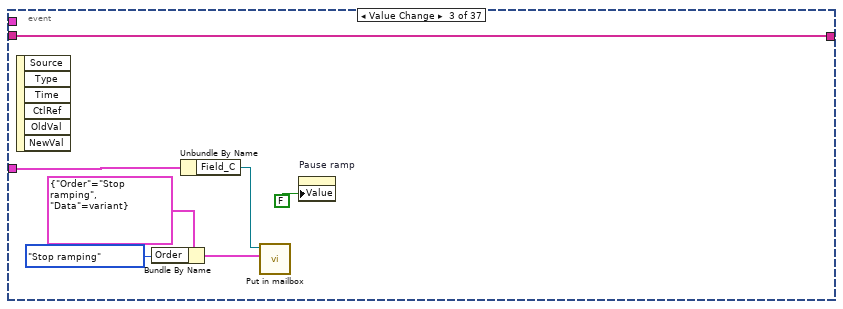
[diagram p9: hidden frame]
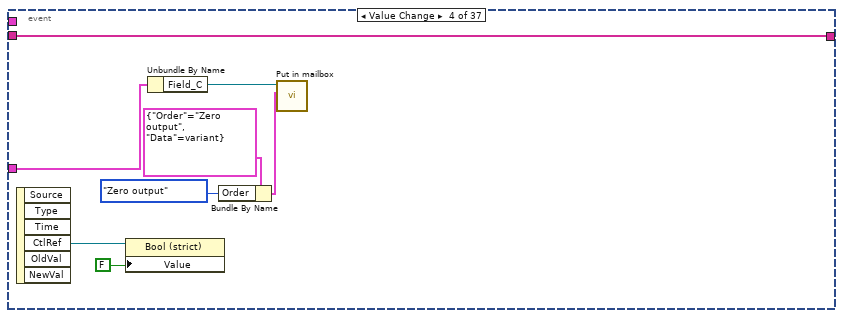
[diagram p10: hidden frame]
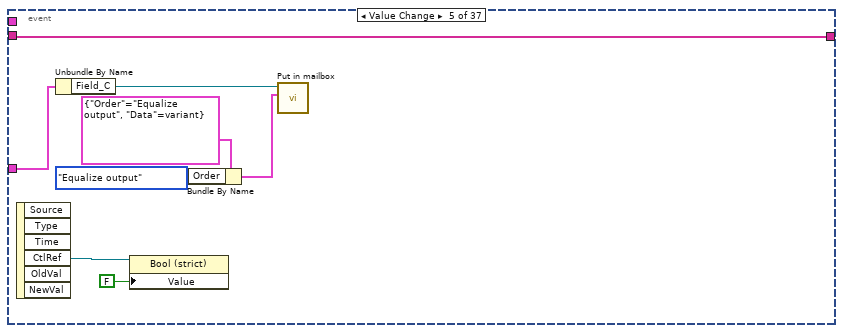
[diagram p11: hidden frame]
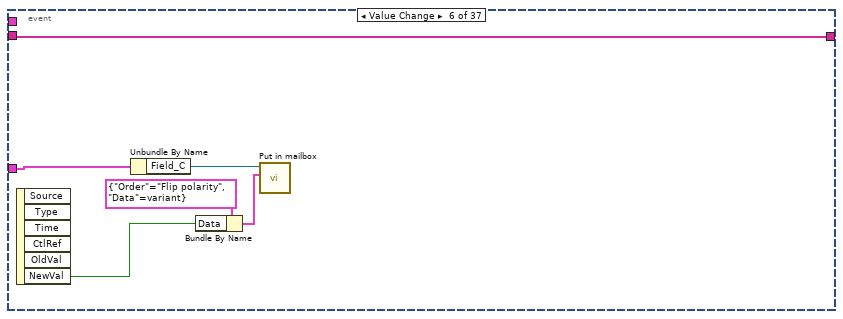
[diagram p12: hidden frame]
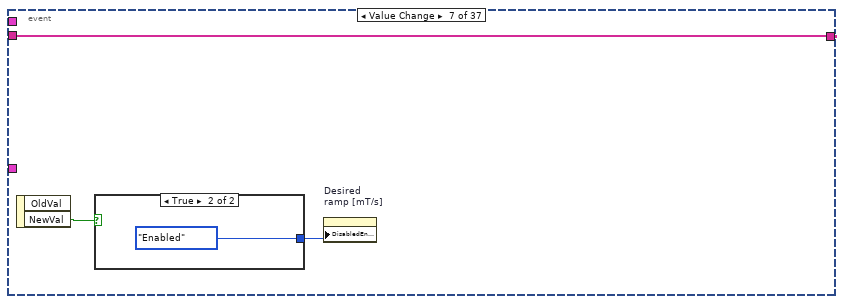
[diagram p13: hidden frame]
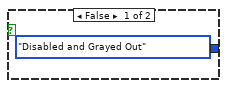
[diagram p14: hidden frame]
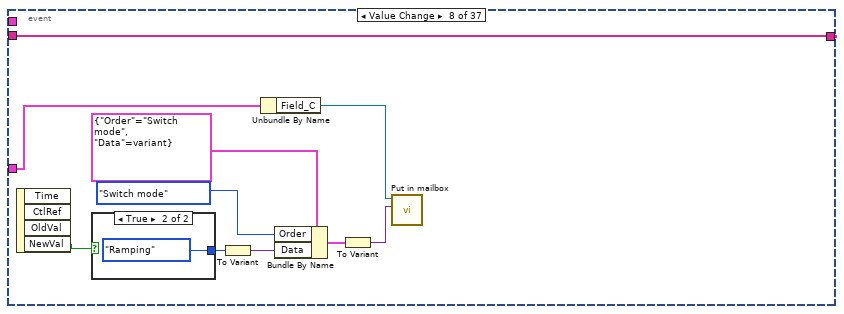
[diagram p15: hidden frame]
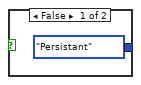
[diagram p16: hidden frame]
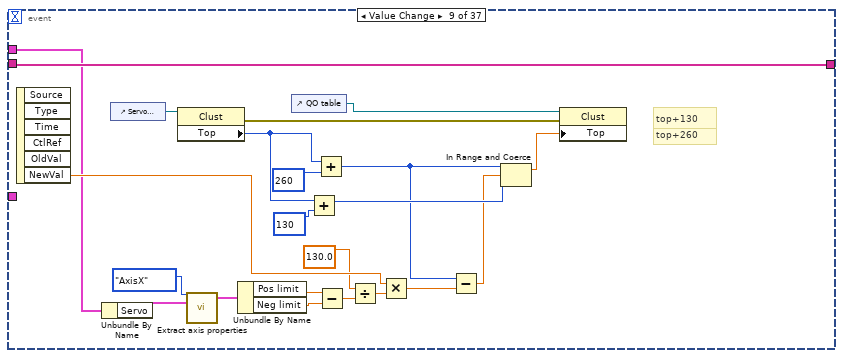
[diagram p17: hidden frame]
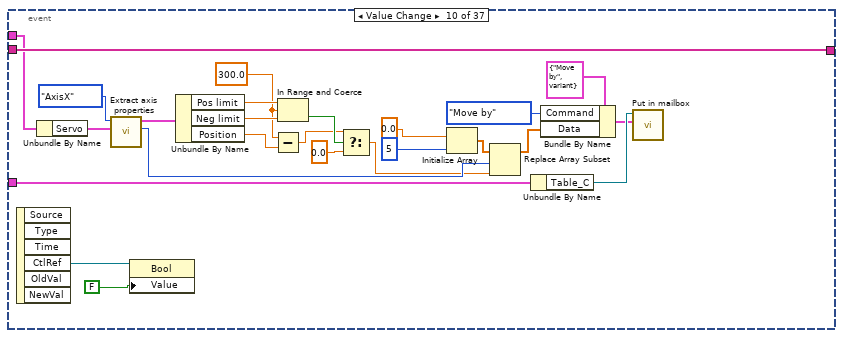
[diagram p18: hidden frame]
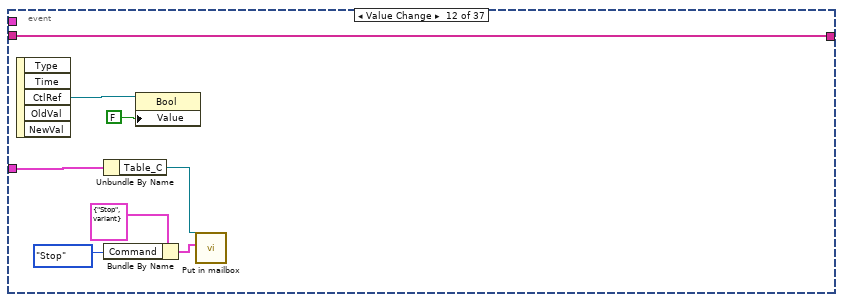
[diagram p20: hidden frame]
diagram:
  w1 = T27 {"Start"=nan, "Start Caption"="Start [T]", "End"=0.0, "End Caption"="End [T]", "Sweep"=0.0, "Sweep caption"="Rate [mT/s]", "Constant"=0.0, "Constant caption"="Freq [GHz]", "Mod_F [kHz]"=0.0, "Mod_A [G]"=0.0, "Tau [ms]"=0.0, "Angle [°]"=0.0, "Tmp [K]"=50.0, "Wait [min]"=0.0, "Carousel"=-1, "Comment"="", "Auto-mod"=TRUE, "Execute"=FALSE}  # Script Line
  w4 = T25 {"Remains"=0.0, "T_sample [K]"=1.6, "Last log"="", "Experiment state"=enum."Setup", "Field [T]"=0.0, "Sample holder"=enum."Simple", "Started"=timestamp(0 s since 1904-01-01)}  # Infobar
  n1 = call "Initialize Messenger.vi"() -> ("Referencies out"=w10:T31)  [unwired: 2 in, 1 out]
  n2 = Initialize Array("", 200 ("dimension size")) -> (w7:string[])
  n3 = while {
    tunnel: w10 -> [w25]
    shift-right: [w14] -> _
    shift-left: w7 -> [w24]
    shift-right: [w22] -> w5
    shift-left: TopStates."Initialize GUI" ("State") -> [w23]
    shift-right: [w20] -> _
    shift-left: _ -> [w19]
    shift-right: [w11] -> _
    shift-left: w1 -> [w17]
    shift-right: [w15] -> _
    shift-left: w4 -> [w16]
    shift-right: [w12] -> _
    shift-left: T8 {"Magnet"={"PSU"="None", "T monitor"="None", "Last update"=timestamp(0 s since 1904-01-01), "Field [T]"=0.0, "Ramp [mT/s]"=0.0, "Heater"=FALSE, "Ramp state"=enum."At Target"}, "MFLI"={"Lock-in"="None", "Multimeter"="None", "Last update"=timestamp(0 s since 1904-01-01), "Freq [kHz]"=0.0, "Ampl [mV]"=0.0, "OutEn"=FALSE, "In50 Ohm"=FALSE, "DemEn"=FALSE}, "THz"={"Name"="None", "Description"="None", "Last update"=timestamp(0 s since 1904-01-01), "Start [GHz]"=0.0, "Im Freq[MHz]"=0.0, "End [GHz]"=0.0}, "VTI"={"TempCtl"="", "Last update"=timestamp(0 s since 1904-01-01), "VTI [K]"=0.0, "Sample [K]"=0.0, "Trap[K]"=0.0, "HePot [K]"=0.0, "Ambient [K]"=0.0}, "Rotator"={"Name"=0, "Last update"=timestamp(0 s since 1904-01-01), "Actuator"=0, "Connected"=FALSE, "Moving"=FALSE, "Target"=FALSE, "Cap [nF]"=0.0, "Position [°]"=0.0}, "Servo"=[{"Name"=enum."Unknown", "Last update"=timestamp(0 s since 1904-01-01), "Position"=0.0, "Pos limit"=0.0, "Neg limit"=0.0, "Power"=FALSE}], "SMU"={"Name"="", "Last update"=timestamp(0 s since 1904-01-01), "SourFunc"="None", "SourValue"=0.0, "MeasFunc"="", "MeasValue"=0.0, "Output"=FALSE}, "PMD"={"Name"="", "Last update"=timestamp(0 s since 1904-01-01), "Position [°]"=0.0, "Speed"=0.0, "Desired [°]"=0.0, "Moving"=FALSE, "reserved"=0.0}, "PwrMonitor"={"Name"="", "Last update"=timestamp(0 s since 1904-01-01), "Outage?"=FALSE, "Low"=FALSE, "No battery"=FALSE, "Battery [%]"=0, "Charging"=FALSE}} ("Instr info") -> [w13]
    stop <- w21 stop-if-true
    # "State Machine While Loop"
    n4 = case shown="\"Wait for Event\"" w23 {
      tunnel: w25 -> [_ w125 w1412 w2843 _ _]
      tunnel: w24 -> [w88 w124 w1426 w2842 w3123 _]
      tunnel: [w87 w113 w1425 w2841 w3122 w3128] -> w14
      tunnel: [TopStates."Wait for Event" ("State") TopStates."Check message" ("State") w1415 TopStates."Wait for Event" ("State") TopStates."Stop" ("State") TopStates."Initialize GUI" ("State")] -> w22
      tunnel: [_ w122 _ _ _ _] -> w21
      tunnel: [w74 w114 w1413 w2838 w3120 w3127] -> w11
      tunnel: w17 -> [w74 w120 w1413 w2839 w3120 w3127]
      tunnel: [w72 w115 w1414 w2840 w3119 w3126] -> w15
      tunnel: w16 -> [w73 w119 w1409 w2835 w3119 w3126]
      tunnel: w13 -> [w64 w116 w1411 w2836 w3118 w3125]
      tunnel: [w64 w116 w1410 w2836 w3118 w3125] -> w12
      frame "Initialize GUI", Default {
        w34 = FALSE ("Hide script")
        w42 = T2 {"To disable"=[], "To enable"=[]}  # Controls referencies
        w63 = TRUE ("Visible")
        n5 = local read "Use previous settings"() -> (w57:bool)
        n6 = property on="Actual measurement" class="Clust (strict)"("Visible"=w34) -> ()  [unwired: 2 in, 2 out]
        n7 = local write "Hide script"(w34) -> ()
        n8 = case shown="True" w57 {
          tunnel: [w98 w100] -> w60
          tunnel: [T19 {"Filter order"=7.0, "Filter tau [ms]"=50.0, "F_Mod [kHz]"=1.0, "Amp_Mod [mV]"=1.0, "Enable output"=0, "Phase [°]"=0.0} ("ACQ parameters") w103] -> w54
          frame False {
            w98 = T22 {"AMC"=9, "Multip"=1, "Base frequency [GHz]"=90.0, "End frequency [GHz]"=90.0, "Im frequency [MHz]"=10.0, "Sweep up [ms]"=0.0, "Reset trigger?"=FALSE}  # VDI control
          }
          frame True {
            n9 = local read "THz control"() -> (w102:T22)
            n10 = call "Open config file.vi"("MAG config file path"="System config file path") -> ("error out"=w111:errorcluster, "Refnum out"=w112:T76)  [unwired: 7 in, 2 out]
            n11 = property on="ACQ parameters" class="Clust (strict)"() -> ("Value"=w101:T19)  [unwired: 2 in, 2 out]
            n12 = call <userlib>:"Read Section Cluster__ogtk.vi"("error in (no error)"=w111, "Section Formatted Cluster Type"=w101, "refnum"=w112) -> ("Section Formatted Cluster"=w110:variant, "dup refnum"=w107:T76)  [unwired: 4 in, 3 out]
            n13 = Variant To Data(type=w101, Variant=w110) -> (data=w103:T19)  [unwired: 1 in, 1 out]
            n14 = call <userlib>:"Read Section Cluster__ogtk.vi"("Section Formatted Cluster Type"=w102, "refnum"=w107) -> ("error out"=w109:errorcluster, "Section Formatted Cluster"=w108:variant, "dup refnum"=w106:T76)  [unwired: 5 in, 2 out]
            n15 = Variant To Data(error in=w109, type=w102, Variant=w108) -> (data=w100:T22, error out=w104:errorcluster)
            n16 = call <vilib>:"Close Config Data.vi"("error in (no error)"=w104, "refnum"=w106) -> ("file path"=w99:path)  [unwired: 8 in, 1 out]
            n17 = local write "System config file path"(w99) -> ()
          }
        }
        n18 = control-ref of="Acquisition controls"() -> (w76:refnum<vi>)
        n19 = control-ref of="VID control"() -> (w58:refnum<vi>)
        n20 = control-ref of="VTI control"() -> (w59:refnum<vi>)
        n21 = control-ref of="Magnet controls"() -> (w75:refnum<vi>)
        n22 = control-ref of="Run script btn"() -> (w52:refnum<vi>)
        n23 = control-ref of="Servo controls"() -> (w65:refnum<vi>)
        n24 = local read "Acquisition controls"() -> (w56:T21)
        n25 = local write "Select module"(Module_selection."All" ("Module")) -> ()
        n26 = local write "Tab Control"(T6."Page Status" ("Tab Control")) -> ()
        n27 = Build Array(w76, w58, w59, w65, w75) -> (w66:refnum<vi>[])
        "Instr control refs" <- w66
        n28 = property on="Script Array" class="Arr (strict)"("Visible"=w63) -> ()  [unwired: 2 in, 2 out]
        n29 = property on="Instr control refs" class="Arr (strict)"("Visible"=w63) -> ()  [unwired: 2 in, 2 out]
        n30 = Build Array (concatenate)(w66, w52) -> (w33:refnum<vi>[])
        n31 = Unbundle By Name(w56) -> ("Sample holder"=w30:T20)
        n32 = property class="Clust"(reference=w65) -> ("Top"=w69:i32)  [unwired: 1 in, 2 out]
        n33 = call "Dis- or en- able controls.vi"("Disabled"=T34."Disabled and Grayed Out", "Control referencies"=w33) -> ()  [unwired: 9 in, 1 out]
        n34 = control-ref of="QO table"() -> (w68:refnum<vi>)
        n35 = Add(x=w69, y=260 ("Position:Top")) -> (x+y=w70:i32)
        n36 = Bundle By Name(cluster=w73, "Sample holder"=w30, "Experiment state"=experiment_state."Setup" ("Value")) -> (w72:T25)
        n37 = property class="Clust"(reference=w68, "Top"=w70) -> ()  [unwired: 1 in, 2 out]
        n38 = call <vilib>:"Is Path and Not Empty.vi"("path"="Main data folder") -> ("Is Path and Not Empty?"=w32:bool)  [unwired: 4 in]
        n39 = case shown="False" w32 {
          frame False {
            w94 = T77 2 items=["User Home"=0, "User Desktop"=1, "User Documents"=2, "User Application Data"=3, "User Preferences"=4, "User Temporary"=5, "Public Documents"=6, "Public Application Data"=7, "Public Preferences"=8, "Public Cache"=13, "System Core Libraries"=9, "System Installed Libraries"=10, "Application Files"=11, "Boot Volume Root"=12] ("system directory type")
            n40 = Format Date/Time String(time format string (%c)="%Y") -> (date/time string=w90:string)  [unwired: 2 in]
            n41 = call <vilib>:"Get System Directory.vi"("system directory type"=w94) -> ("system directory"=w96:path)  [unwired: 10 in]
            n42 = Build Path(base path=w96, name or relative path="Measurements") -> (appended path=w95:path)
            n43 = Build Path(base path=w95, name or relative path=w90) -> (appended path=w92:path)
            n44 = local write "Main data folder"(w92) -> ()
          }
          frame True {
          }
        }
        n45 = control-ref of="Save script file btn"() -> (w35:refnum<vi>)
        n46 = local write "THz control"(w60) -> ()
        n47 = property on="ACQ parameters" class="Clust (strict)"("Value"=w54) -> ()  [unwired: 2 in, 2 out]
        n48 = control-ref of="Load script btn"() -> (w36:refnum<vi>)
        n49 = control-ref of="Open measurement"() -> (w37:refnum<vi>)
        n50 = control-ref of="Direct stop meas. btn"() -> (w40:refnum<vi>)
        n51 = Initialize Array("Empty", 10 ("dimension size")) -> (w44:string[])
        n52 = Build Array (concatenate)(w35, w36, w37, w33) -> (w38:refnum<vi>[])
        n53 = property on="Data file to show" class="Ring (strict)"("Strings []"=w44) -> ()  [unwired: 2 in, 2 out]
        n54 = Build Array(w40) -> (w39:refnum<vi>[])
        n55 = call "Create new Log files.vi"("Log folder"="Log folder") -> ("error out"=w82:errorcluster, "dup path"=w53:path, "tmp logfile out"=→"Temperature log ref":refnum<file>, "event logfile out"=w83:refnum<file>)  [unwired: 7 in]
        n56 = Bundle By Name(cluster=w42, "To disable"=w38, "To enable"=w39) -> (→"Controls referencies":T2)
        n57 = Initialize Array(0.0 ("element"), 12 ("dimension size")) -> (w29:dbl[])
        n58 = local write "Log folder"(w53) -> ()
        n59 = call "Add actual date time to string.vi"("String in"="GUI initialized") -> ("String out"=w81:string)  [unwired: 4 in]
        n60 = local write "Drift[K/s]"(w29) -> ()
        n61 = Concatenate Strings(w81, "\r\n") -> (w80:string)
        n62 = call "simple Shift string array.vi"("Element in"=w81, "Array in"=w88) -> ("Array out"=w87:string[])  [unwired: 8 in, 1 out]
        n63 = Write to Text File(file (use dialog)=w83, text=w80, error in=w82) -> (refnum out=→"loggersRef":refnum<file>)  [unwired: 1 in, 2 out]
        n64 = Initialize Array(T32 {"Mode"=enum."MD EPR", "Array"=[]} ("Results"), 10 ("dimension size")) -> (→"Results":T32[])
        n65 = Initialize Array("", 10 ("dimension size")) -> (w50:string[])
        n66 = local write "Header"(w50) -> ()
        "Instr status" <- T1 {"Mag"=FALSE, "Rot"=FALSE, "VTI"=FALSE, "MFLI"=FALSE, "Serv"=FALSE, "THz"=FALSE, "ADQ7"=FALSE, "SMU"=FALSE, "PMD"=FALSE, "UPS"=FALSE, "DMM"=FALSE, "abc"=FALSE} ("Instruments status 2")
        "Infobar" <- T25 {"Remains"=0.0, "T_sample [K]"=0.0, "Last log"="", "Experiment state"=enum."Setup", "Field [T]"=0.0, "Sample holder"=enum."Simple", "Started"=timestamp(0 s since 1904-01-01)} ("Infobar")
      }
      frame "Wait for Event" {
        n67 = event shown="[0] Timeout" {
          selector: _ -> [_ _ _ _ _]
          dyn-events: _ -> [_ _ _ _ _]
          timeout: 5 -> [_ _ _ _ _]
          tunnel: w124 -> [w132 w1137 w1147 w1219 w1303]
          tunnel: [w134 w1137 w1147 w1219 w1302] -> w113
          tunnel: w125 -> [w127 _ w1141 w1221 w1304]
          tunnel: [_ _ _ w1220 _] -> w122
          tunnel: [w131 w1140 w1146 w1218 w1301] -> w114
          tunnel: w120 -> [w130 w1140 w1146 w1218 w1301]
          tunnel: [w129 w1139 w1145 w1217 w1300] -> w117
          tunnel: w119 -> [w128 w1139 w1145 w1217 w1300]
          tunnel: w116 -> [w126 _ _ _ _]
          event Timeout {
            n68 = event-data() -> ()  [unwired: 1 in, 3 out]
            n69 = case shown="\"Adjustment\", Default" "Tab Control" {
              tunnel: [w138 w145 w842 w976 w1080] -> w134
              tunnel: w132 -> [w138 w143 w843 w976 w1080]
              tunnel: w127 -> [_ w142 w840 _ _]
              tunnel: [w137 w141 w839 w975 w1079] -> w131
              tunnel: w130 -> [w137 w141 w838 w975 w1079]
              tunnel: [w136 w140 w836 w974 w1078] -> w129
              tunnel: w128 -> [w136 w140 w837 w974 w1078]
              tunnel: w126 -> [w135 w139 _ _ _]
              frame "Page Status" {
                n70 = local write "Instr info"(w135) -> ()
              }
              frame "Adjustment", Default {
                n71 = event shown="[10] \"Servo controls.Measure Position btn\": Value Change" {
                  selector: _ -> [_ _ _ _ _ _ _ _ _ _ _ _ _ _ _ _ _ _ _ _ _ _ _ _ _ _ _ _ _ _ _ _ _ _ _ _ _]
                  dyn-events: _ -> [_ _ _ _ _ _ _ _ _ _ _ _ _ _ _ _ _ _ _ _ _ _ _ _ _ _ _ _ _ _ _ _ _ _ _ _ _]
                  timeout: 0 -> [_ _ _ _ _ _ _ _ _ _ _ _ _ _ _ _ _ _ _ _ _ _ _ _ _ _ _ _ _ _ _ _ _ _ _ _ _]
                  tunnel: w143 -> [w146 w162 w177 w185 w193 w199 w200 w209 w219 w263 w273 w302 w316 w341 w367 w397 w432 w477 w506 w531 w557 w582 w608 w633 w666 w679 w687 w709 w718 w733 w784 w793 w804 w813 w820 w827 w833]
                  tunnel: [w146 w166 w177 w185 w193 w199 w200 w209 w219 w263 w273 w302 w316 w341 w367 w397 w432 w477 w506 w531 w557 w582 w608 w633 w666 w679 w687 w709 w718 w733 w784 w793 w804 w813 w820 w827 w833] -> w145
                  tunnel: w142 -> [_ w152 w171 w180 w188 w195 _ w205 _ w253 w270 w299 w307 w332 w358 w383 w408 w452 w497 w522 w548 w573 w599 w624 w652 w675 w684 w700 _ w732 w783 w790 w803 w808 w814 w823 _]
                  tunnel: w139 -> [_ _ _ _ _ _ _ _ w218 w240 w265 _ w304 w328 w354 w379 w405 w448 w494 w518 w544 w569 w595 w620 w665 _ _ _ _ _ _ _ _ _ _ _ _]
                  event Timeout {
                    (unwired) TopStates."Check message" ("State")
                    n72 = event-data() -> ()  [unwired: 1 in, 3 out]
                  }
                  event Value Change {
                    w147 = 16.0  # MaxB[T]
                    n73 = event-data() -> ()  [unwired: 1 in, 6 out]
                    n74 = local read "Magnet controls"() -> (w168:T24)
                    n75 = Unbundle By Name(w168) -> ("Set Field [T]"=w159:dbl, "Desired\nramp [mT/s]"=w149:dbl, "Custom\nramp"=w155:bool)
                    n76 = Greater?(x=w159, y=w147) -> (0:w160:bool)
                    n77 = Divide(x=w149, y=1000.0) -> (x/y=w150:dbl)
                    n78 = Select(t=w147, s=w160, f=w159) -> (s? t:f=w157:dbl)
                    n79 = Bundle By Name(cluster=T36 {"Field [T]"=0.0, "Ramp [T/s]"=0.0, "Custom Ramp?"=FALSE, "Mode"=enum."Persistant"} ("Set Field"), "Field [T]"=w157, "Ramp [T/s]"=w150, "Custom Ramp?"=w155, "Mode"=Magnet_mode_public."Ramping") -> (w156:T36)
                    n80 = Format Into String(format string="%f T", initial string="Invalid field value" ("Element in"), w159) -> (resulting string=w163:string)  [unwired: 1 in, 1 out]
                    n81 = call "simple Shift string array.vi"("Element in"=w163, "Array in"=w162) -> ("Array out"=w161:string[])  [unwired: 8 in, 1 out]
                    n82 = Bundle By Name(cluster=T38 {"Order"=enum."Set field", "Data"=variant(enum16{"Ramping", "Perzistant"} enum."Ramping")} ("MSG to magnet"), "Order"=Magnet_Orders."Set field", "Data"=w156) -> (w170:T38)
                    n83 = Select(t=w161, s=w160, f=w162) -> (s? t:f=w166:string[])
                    n84 = Unbundle By Name(w152) -> ("Field_C"=w154:refnum<queue>)
                    n85 = To Variant(anything=w170) -> (Variant=w153:variant)
                    n86 = call "Put in mailbox.vi"("Message"=w153, "Queue in"=w154) -> ()  [unwired: 7 in, 3 out]
                  }
                  event Value Change {
                    n87 = event-data() -> ()  [unwired: 1 in, 6 out]
                    n88 = Bundle By Name(cluster=T38 {"Order"=enum."Stop ramping", "Data"=variant(enum16{"Ramping", "Perzistant"} enum."Ramping")} ("MSG to magnet"), "Order"=Magnet_Orders."Stop ramping") -> (w174:T38)
                    n89 = Unbundle By Name(w171) -> ("Field_C"=w175:refnum<queue>)
                    n90 = call "Put in mailbox.vi"("Message"=w174, "Queue in"=w175) -> ()  [unwired: 7 in, 3 out]
                    n91 = property on="Pause ramp" class="Bool (strict)"("Value"=FALSE) -> ()  [unwired: 2 in, 2 out]
                  }
                  event Value Change {
                    n92 = event-data() -> ("CtlRef"=w179:refnum<vi>)  [unwired: 1 in, 5 out]
                    n93 = property class="Bool (strict)"(reference=w179, "Value"=FALSE) -> ()  [unwired: 1 in, 2 out]
                    n94 = Unbundle By Name(w180) -> ("Field_C"=w182:refnum<queue>)
                    n95 = Bundle By Name(cluster=T38 {"Order"=enum."Zero output", "Data"=variant(enum16{"Ramping", "Perzistant"} enum."Ramping")} ("MSG to magnet"), "Order"=Magnet_Orders."Zero output") -> (w181:T38)
                    n96 = call "Put in mailbox.vi"("Message"=w181, "Queue in"=w182) -> ()  [unwired: 7 in, 3 out]
                  }
                  event Value Change {
                    n97 = event-data() -> ("CtlRef"=w186:refnum<vi>)  [unwired: 1 in, 5 out]
                    n98 = Unbundle By Name(w188) -> ("Field_C"=w190:refnum<queue>)
                    n99 = property class="Bool (strict)"(reference=w186, "Value"=FALSE) -> ()  [unwired: 1 in, 2 out]
                    n100 = Bundle By Name(cluster=T38 {"Order"=enum."Equalize output", "Data"=variant(enum16{"Ramping", "Perzistant"} enum."Ramping")} ("MSG to magnet"), "Order"=Magnet_Orders."Equalize output") -> (w189:T38)
                    n101 = call "Put in mailbox.vi"("Message"=w189, "Queue in"=w190) -> ()  [unwired: 7 in, 3 out]
                  }
                  event Value Change {
                    n102 = event-data() -> ("NewVal"=w194:bool)  [unwired: 1 in, 5 out]
                    n103 = Unbundle By Name(w195) -> ("Field_C"=w197:refnum<queue>)
                    n104 = Bundle By Name(cluster=T38 {"Order"=enum."Flip polarity", "Data"=variant(enum16{"Ramping", "Perzistant"} enum."Ramping")} ("MSG to magnet"), "Data"=w194) -> (w196:T38)
                    n105 = call "Put in mailbox.vi"("Message"=w196, "Queue in"=w197) -> ()  [unwired: 7 in, 3 out]
                  }
                  event Value Change {
                    n106 = event-data() -> ("NewVal"=w202:bool)  [unwired: 1 in, 1 out]
                    n107 = case shown="True" w202 {
                      tunnel: [T34."Disabled and Grayed Out" ("Disabled") T34."Enabled" ("Disabled")] -> w201
                      frame False {
                      }
                      frame True {
                      }
                    }
                    n108 = property on="Desired\nramp [mT/s]" class="DigNum (strict)"("DisabledEnum"=w201) -> ()  [unwired: 2 in, 2 out]
                  }
                  event Value Change {
                    n109 = event-data() -> ("NewVal"=w210:bool)  [unwired: 1 in, 3 out]
                    n110 = case shown="True" w210 {
                      tunnel: [Magnet_mode_public."Persistant" ("Operation mode") Magnet_mode_public."Ramping" ("Operation mode")] -> w211
                      frame False {
                      }
                      frame True {
                      }
                    }
                    n111 = To Variant(anything=w211) -> (Variant=w208:variant)
                    n112 = Unbundle By Name(w205) -> ("Field_C"=w207:refnum<queue>)
                    n113 = Bundle By Name(cluster=T38 {"Order"=enum."Switch mode", "Data"=variant(enum16{"Ramping", "Perzistant"} enum."Ramping")} ("MSG to magnet"), "Order"=Magnet_Orders."Switch mode", "Data"=w208) -> (w214:T38)
                    n114 = To Variant(anything=w214) -> (Variant=w206:variant)
                    n115 = call "Put in mailbox.vi"("Message"=w206, "Queue in"=w207) -> ()  [unwired: 7 in, 3 out]
                  }
                  event Value Change {
                    # "top+260"
                    # "top+130"
                    n116 = event-data() -> ("NewVal"=w230:dbl)  [unwired: 1 in, 5 out]
                    n117 = Unbundle By Name(w218) -> ("Servo"=w217:T10[])
                    n118 = control-ref of="Servo controls"() -> (w238:refnum<vi>)
                    n119 = property class="Clust"(reference=w238) -> (error out=w229:errorcluster, "Top"=w224:i32)  [unwired: 1 in, 1 out]
                    n120 = call "Extract axis properties.vi"("Name"=Axis_names."AxisX", "All servo status"=w217) -> ("Servo"=w235:T10)  [unwired: 6 in, 2 out]
                    n121 = Unbundle By Name(w235) -> ("Pos limit"=w233:dbl, "Neg limit"=w232:dbl)
                    n122 = control-ref of="QO table"() -> (w234:refnum<vi>)
                    n123 = Add(x=w224, y=130) -> (x+y=w226:i32)
                    n124 = Add(x=w224, y=260) -> (x+y=w223:i32)
                    n125 = Subtract(x=w233, y=w232) -> (x-y=w220:dbl)
                    n126 = Divide(x=130.0 ("y"), y=w220) -> (x/y=w231:dbl)
                    n127 = Multiply(x=w230, y=w231) -> (x*y=w227:dbl)
                    n128 = Subtract(x=w223, y=w227) -> (x-y=w222:dbl)
                    n129 = In Range and Coerce(upper limit=w223, x=w222, lower limit=w226) -> (coerced(x)=w237:dbl)  [unwired: 1 out]
                    n130 = property class="Clust"(reference=w234, error in=w229, "Top"=w237) -> ()  [unwired: 2 out]
                  }
                  event Value Change {
                    w245 = 300.0 ("x")
                    n131 = event-data() -> ("CtlRef"=w262:refnum<vi>)  [unwired: 1 in, 5 out]
                    n132 = Unbundle By Name(w240) -> ("Servo"=w239:T10[])
                    n133 = call "Extract axis properties.vi"("Name"=Axis_names."AxisX", "All servo status"=w239) -> ("Servo"=w260:T10, "Index"=w251:i32)  [unwired: 6 in, 1 out]
                    n134 = property class="Bool"(reference=w262, "Value"=FALSE) -> ()  [unwired: 1 in, 2 out]
                    n135 = Unbundle By Name(w260) -> ("Pos limit"=w247:dbl, "Neg limit"=w246:dbl, "Position"=w248:dbl)
                    n136 = Subtract(x=w245, y=w248) -> (x-y=w242:dbl)
                    n137 = In Range and Coerce(upper limit=w247, x=w245, lower limit=w246) -> (In Range?=w244:bool)  [unwired: 1 out]
                    n138 = Select(t=w242, s=w244, f=0.0) -> (s? t:f=w241:dbl)
                    n139 = Initialize Array(0.0 ("element"), 5 ("dimension size")) -> (w249:dbl[])
                    n140 = Replace Array Subset(array=w249, new element=w241, index=w251) -> (w250:dbl[])
                    n141 = Unbundle By Name(w253) -> ("Table_C"=w254:refnum<queue>)
                    n142 = Bundle By Name(cluster=T40 {"Command"=enum."Move by", "Data"=variant(dbl[] [])} ("MSG to Servo"), "Command"=Servo_commands."Move by", "Data"=w250) -> (w252:T40)
                    n143 = call "Put in mailbox.vi"("Message"=w252, "Queue in"=w254) -> ()  [unwired: 7 in, 3 out]
                  }
                  event Value Change {
                    n144 = event-data() -> ("CtlRef"=w272:refnum<vi>, "NewVal"=w269:bool)  [unwired: 1 in, 2 out]
                    n145 = Unbundle By Name(w265) -> ("Servo"=w264:T10[])
                    n146 = property class="Bool"(reference=w272, "Value"=FALSE) -> ()  [unwired: 1 in, 2 out]
                    n147 = call "Timeout dialoge Abbort.vi"("Enable"=w269, "Message to Display"="Really go to measurement position?", "timeout[ms]"=u32 3000) -> ("Yes"=w266:bool)  [unwired: 15 in, 1 out]
                    n148 = case shown="True" w266 {
                      tunnel: w270 -> [_ w287]
                      tunnel: w264 -> [_ w275]
                      frame False {
                      }
                      frame True {
                        w274 = 916.0 ("x")
                        # "previous\n890\n895\n899"
                        n149 = call "Extract axis properties.vi"("Name"=Axis_names."AxisX", "All servo status"=w275) -> ("Servo"=w294:T10, "Index"=w285:i32)  [unwired: 6 in, 1 out]
                        n150 = Unbundle By Name(w294) -> ("Pos limit"=w281:dbl, "Neg limit"=w280:dbl, "Position"=w282:dbl)
                        n151 = Subtract(x=w274, y=w282) -> (x-y=w277:dbl)
                        n152 = In Range and Coerce(upper limit=w281, x=w274, lower limit=w280) -> (In Range?=w279:bool)  [unwired: 1 out]
                        n153 = Unbundle By Name(w287) -> ("Table_C"=w288:refnum<queue>)
                        n154 = Select(t=w277, s=w279, f=0.0) -> (s? t:f=w276:dbl)
                        n155 = Initialize Array(0.0 ("element"), 5 ("dimension size")) -> (w283:dbl[])
                        n156 = Replace Array Subset(array=w283, new element=w276, index=w285) -> (w284:dbl[])
                        n157 = Bundle By Name(cluster=T40 {"Command"=enum."Move by", "Data"=variant(dbl[] [])} ("MSG to Servo"), "Command"=Servo_commands."Move by", "Data"=w284) -> (w286:T40)
                        n158 = call "Put in mailbox.vi"("Message"=w286, "Queue in"=w288) -> ()  [unwired: 7 in, 3 out]
                      }
                    }
                  }
                  event Value Change {
                    n159 = event-data() -> ("CtlRef"=w301:refnum<vi>)  [unwired: 1 in, 4 out]
                    n160 = Unbundle By Name(w299) -> ("Table_C"=w296:refnum<queue>)
                    n161 = Bundle By Name(cluster=T40 {"Command"=enum."Stop", "Data"=variant(dbl[] [])} ("MSG to Servo"), "Command"=Servo_commands."Stop") -> (w295:T40)
                    n162 = property class="Bool"(reference=w301, "Value"=FALSE) -> ()  [unwired: 1 in, 2 out]
                    n163 = call "Put in mailbox.vi"("Message"=w295, "Queue in"=w296) -> ()  [unwired: 7 in, 3 out]
                  }
                  event Value Change {
                    # "X position limit"
                    n164 = event-data() -> ("CtlRef"=w305:refnum<vi>)  [unwired: 1 in, 5 out]
                    n165 = Unbundle By Name(w304) -> ("Servo"=w303:T10[])
                    n166 = call "Extract axis properties.vi"("Name"=Axis_names."AxisX", "All servo status"=w303) -> ("Servo"=w313:T10, "Index"=w310:i32)  [unwired: 6 in, 1 out]
                    n167 = property class="Bool"(reference=w305, "Value"=FALSE) -> ()  [unwired: 1 in, 2 out]
                    n168 = Unbundle By Name(w313) -> ("Position"=w308:dbl, "Pos limit"=w311:dbl)
                    n169 = property on="Step\n[mm]" class="DigNum (strict)"() -> ("Value"=w309:dbl)  [unwired: 2 in, 2 out]
                    n170 = Subtract(x=w311, y=w309) -> (x-y=w315:dbl)
                    n171 = Less?(x=w308, y=w315) -> (x < y?=w314:bool)
                    n172 = case shown="True" w314 {
                      tunnel: w309 -> [_ w325]
                      tunnel: w310 -> [_ w321]
                      tunnel: w307 -> [_ w318]
                      frame False {
                      }
                      frame True {
                        n173 = Initialize Array(0.0 ("element"), 5 ("dimension size")) -> (w326:dbl[])
                        n174 = Replace Array Subset(array=w326, new element=w325, index=w321) -> (w322:dbl[])
                        n175 = Bundle By Name(cluster=T40 {"Command"=enum."Move by", "Data"=variant(dbl[] [])} ("MSG to Servo"), "Command"=Servo_commands."Move by", "Data"=w322) -> (w319:T40)
                        n176 = Unbundle By Name(w318) -> ("Table_C"=w320:refnum<queue>)
                        n177 = call "Put in mailbox.vi"("Message"=w319, "Queue in"=w320) -> ()  [unwired: 7 in, 3 out]
                      }
                    }
                  }
                  event Value Change {
                    n178 = event-data() -> ("CtlRef"=w330:refnum<vi>)  [unwired: 1 in, 5 out]
                    n179 = Unbundle By Name(w328) -> ("Servo"=w329:T10[])
                    n180 = property on="Step\n[mm]" class="DigNum (strict)"() -> ("Value"=w334:dbl)  [unwired: 2 in, 2 out]
                    n181 = call "Extract axis properties.vi"("Name"=Axis_names."AxisX", "All servo status"=w329) -> ("Servo"=w338:T10, "Index"=w335:i32)  [unwired: 6 in, 1 out]
                    n182 = property class="Bool"(reference=w330, "Value"=FALSE) -> ()  [unwired: 1 in, 2 out]
                    n183 = Unbundle By Name(w338) -> ("Position"=w333:dbl, "Neg limit"=w336:dbl)
                    n184 = Add(x=w336, y=w334) -> (x+y=w339:dbl)
                    n185 = Greater?(x=w333, y=w339) -> (0:w340:bool)
                    n186 = case shown="True" w340 {
                      tunnel: w334 -> [_ w350]
                      tunnel: w335 -> [_ w346]
                      tunnel: w332 -> [_ w343]
                      frame False {
                      }
                      frame True {
                        n187 = Negate(x=w350) -> (-x=w352:dbl)
                        n188 = Initialize Array(0.0 ("element"), 5 ("dimension size")) -> (w351:dbl[])
                        n189 = Replace Array Subset(array=w351, new element=w352, index=w346) -> (w347:dbl[])
                        n190 = Unbundle By Name(w343) -> ("Table_C"=w344:refnum<queue>)
                        n191 = Bundle By Name(cluster=T40 {"Command"=enum."Move by", "Data"=variant(dbl[] [])} ("MSG to Servo"), "Command"=Servo_commands."Move by", "Data"=w347) -> (w342:T40)
                        n192 = call "Put in mailbox.vi"("Message"=w342, "Queue in"=w344) -> ()  [unwired: 7 in, 3 out]
                      }
                    }
                  }
                  event Value Change {
                    w364 = 0.5 ("y")
                    n193 = event-data() -> ("CtlRef"=w356:refnum<vi>)  [unwired: 1 in, 3 out]
                    n194 = Unbundle By Name(w354) -> ("Servo"=w355:T10[])
                    n195 = call "Extract axis properties.vi"("Name"=Axis_names."AxisY", "All servo status"=w355) -> ("Servo"=w363:T10, "Index"=w360:i32)  [unwired: 6 in, 1 out]
                    n196 = Unbundle By Name(w363) -> ("Position"=w359:dbl, "Pos limit"=w361:dbl)
                    n197 = property class="Bool"(reference=w356, "Value"=FALSE) -> ()  [unwired: 1 in, 2 out]
                    n198 = Subtract(x=w361, y=w364) -> (x-y=w365:dbl)
                    n199 = Less?(x=w359, y=w365) -> (x < y?=w366:bool)
                    n200 = case shown="True" w366 {
                      tunnel: w364 -> [_ w376]
                      tunnel: w360 -> [_ w372]
                      tunnel: w358 -> [_ w368]
                      frame False {
                      }
                      frame True {
                        n201 = Initialize Array(0.0 ("element"), 5 ("dimension size")) -> (w377:dbl[])
                        n202 = Replace Array Subset(array=w377, new element=w376, index=w372) -> (w373:dbl[])
                        n203 = Bundle By Name(cluster=T40 {"Command"=enum."Move by", "Data"=variant(dbl[] [])} ("MSG to Servo"), "Command"=Servo_commands."Move by", "Data"=w373) -> (w369:T40)
                        n204 = Unbundle By Name(w368) -> ("Table_C"=w370:refnum<queue>)
                        n205 = call "Put in mailbox.vi"("Message"=w369, "Queue in"=w370) -> ()  [unwired: 7 in, 3 out]
                      }
                    }
                  }
                  event Value Change {
                    w390 = 0.5 ("y")
                    n206 = event-data() -> ("CtlRef"=w381:refnum<vi>)  [unwired: 1 in, 5 out]
                    n207 = Unbundle By Name(w379) -> ("Servo"=w380:T10[])
                    n208 = call "Extract axis properties.vi"("Name"=Axis_names."AxisY", "All servo status"=w380) -> ("Servo"=w388:T10, "Index"=w385:i32)  [unwired: 6 in, 1 out]
                    n209 = Unbundle By Name(w388) -> ("Position"=w384:dbl, "Neg limit"=w387:dbl)
                    n210 = property class="Bool"(reference=w381, "Value"=FALSE) -> ()  [unwired: 1 in, 2 out]
                    n211 = Add(x=w387, y=w390) -> (x+y=w389:dbl)
                    n212 = Negate(x=w390) -> (-x=w391:dbl)
                    n213 = Greater?(x=w384, y=w389) -> (0:w396:bool)
                    n214 = Initialize Array(0.0 ("element"), 5 ("dimension size")) -> (w395:dbl[])
                    n215 = Replace Array Subset(array=w395, new element=w391, index=w385) -> (w392:dbl[])
                    n216 = case shown="True" w396 {
                      tunnel: w392 -> [_ w402]
                      tunnel: w383 -> [_ w399]
                      frame False {
                      }
                      frame True {
                        n217 = Unbundle By Name(w399) -> ("Table_C"=w400:refnum<queue>)
                        n218 = Bundle By Name(cluster=T40 {"Command"=enum."Move by", "Data"=variant(dbl[] [])} ("MSG to Servo"), "Command"=Servo_commands."Move by", "Data"=w402) -> (w398:T40)
                        n219 = call "Put in mailbox.vi"("Message"=w398, "Queue in"=w400) -> ()  [unwired: 7 in, 3 out]
                      }
                    }
                  }
                  event Value Change {
                    w427 = 0.5 ("y")
                    n220 = event-data() -> ("CtlRef"=w406:refnum<vi>)  [unwired: 1 in, 5 out]
                    n221 = Unbundle By Name(w405) -> ("Servo"=w404:T10[])
                    n222 = call "Extract axis properties.vi"("Name"=Axis_names."AxisZ_right", "All servo status"=w404) -> ("Servo"=w425:T10, "Index"=w416:i32)  [unwired: 6 in, 1 out]
                    n223 = call "Extract axis properties.vi"("Name"=Axis_names."AxisZ_middle", "All servo status"=w404) -> ("Servo"=w424:T10, "Index"=w415:i32)  [unwired: 6 in, 1 out]
                    n224 = call "Extract axis properties.vi"("Name"=Axis_names."AxisZ_left", "All servo status"=w404) -> ("Servo"=w426:T10, "Index"=w417:i32)  [unwired: 6 in, 1 out]
                    n225 = property class="Bool"(reference=w406, "Value"=FALSE) -> ()  [unwired: 1 in, 2 out]
                    n226 = Unbundle By Name(w425) -> ("Position"=w411:dbl, "Pos limit"=w419:dbl)
                    n227 = Unbundle By Name(w424) -> ("Position"=w410:dbl, "Pos limit"=w418:dbl)
                    n228 = Unbundle By Name(w426) -> ("Position"=w409:dbl, "Pos limit"=w420:dbl)
                    n229 = Subtract(x=w419, y=w427) -> (x-y=w430:dbl)
                    n230 = Subtract(x=w420, y=w427) -> (x-y=w431:dbl)
                    n231 = Subtract(x=w418, y=w427) -> (x-y=w429:dbl)
                    n232 = Less?(x=w409, y=w431) -> (x < y?=w412:bool)
                    n233 = Less?(x=w411, y=w430) -> (x < y?=w413:bool)
                    n234 = Less?(x=w410, y=w429) -> (x < y?=w414:bool)
                    n235 = Compound Arithmetic op=AND(w413, w414, w412) -> (w428:bool)
                    n236 = case shown="True" w428 {
                      tunnel: w427 -> [_ w439]
                      tunnel: w417 -> [_ w440]
                      tunnel: w416 -> [_ w438]
                      tunnel: w415 -> [_ w437]
                      tunnel: w408 -> [_ w434]
                      frame False {
                      }
                      frame True {
                        n237 = Initialize Array(0.0 ("element"), 5 ("dimension size")) -> (w446:dbl[])
                        n238 = Replace Array Subset(array=w446, new element=w439, index=w438) -> (w443:dbl[])
                        n239 = Replace Array Subset(array=w443, new element=w439, index=w437) -> (w442:dbl[])
                        n240 = Replace Array Subset(array=w442, new element=w439, index=w440) -> (w441:dbl[])
                        n241 = Bundle By Name(cluster=T40 {"Command"=enum."Move by", "Data"=variant(dbl[] [])} ("MSG to Servo"), "Command"=Servo_commands."Move by", "Data"=w441) -> (w435:T40)
                        n242 = Unbundle By Name(w434) -> ("Table_C"=w436:refnum<queue>)
                        n243 = call "Put in mailbox.vi"("Message"=w435, "Queue in"=w436) -> ()  [unwired: 7 in, 3 out]
                      }
                    }
                  }
                  event Value Change {
                    w469 = 0.5 ("y")
                    n244 = event-data() -> ("CtlRef"=w450:refnum<vi>)  [unwired: 1 in, 2 out]
                    n245 = Unbundle By Name(w448) -> ("Servo"=w449:T10[])
                    n246 = property class="Bool"(reference=w450, "Value"=FALSE) -> ()  [unwired: 1 in, 2 out]
                    n247 = call "Extract axis properties.vi"("Name"=Axis_names."AxisZ_middle", "All servo status"=w449) -> ("Servo"=w465:T10, "Index"=w458:i32)  [unwired: 6 in, 1 out]
                    n248 = call "Extract axis properties.vi"("Name"=Axis_names."AxisZ_left", "All servo status"=w449) -> ("Servo"=w468:T10, "Index"=w457:i32)  [unwired: 6 in, 1 out]
                    n249 = call "Extract axis properties.vi"("Name"=Axis_names."AxisZ_right", "All servo status"=w449) -> ("Servo"=w466:T10, "Index"=w456:i32)  [unwired: 6 in, 1 out]
                    n250 = Unbundle By Name(w468) -> ("Position"=w455:dbl, "Neg limit"=w462:dbl)
                    n251 = Unbundle By Name(w465) -> ("Position"=w453:dbl, "Neg limit"=w460:dbl)
                    n252 = Unbundle By Name(w466) -> ("Position"=w454:dbl, "Neg limit"=w461:dbl)
                    n253 = Add(x=w462, y=w469) -> (x+y=w476:dbl)
                    n254 = Add(x=w461, y=w469) -> (x+y=w475:dbl)
                    n255 = Add(x=w460, y=w469) -> (x+y=w474:dbl)
                    n256 = Greater?(x=w455, y=w476) -> (0:w473:bool)
                    n257 = Greater?(x=w454, y=w475) -> (0:w472:bool)
                    n258 = Greater?(x=w453, y=w474) -> (0:w470:bool)
                    n259 = Negate(x=w469) -> (-x=w459:dbl)
                    n260 = Compound Arithmetic op=AND(w473, w472, w470) -> (w471:bool)
                    n261 = case shown="True" w471 {
                      tunnel: w459 -> [_ w485]
                      tunnel: w458 -> [_ w484]
                      tunnel: w457 -> [_ w483]
                      tunnel: w456 -> [_ w482]
                      tunnel: w452 -> [_ w478]
                      frame False {
                      }
                      frame True {
                        n262 = Initialize Array(0.0 ("element"), 5 ("dimension size")) -> (w491:dbl[])
                        n263 = Replace Array Subset(array=w491, new element=w485, index=w484) -> (w488:dbl[])
                        n264 = Replace Array Subset(array=w488, new element=w485, index=w483) -> (w487:dbl[])
                        n265 = Replace Array Subset(array=w487, new element=w485, index=w482) -> (w486:dbl[])
                        n266 = Bundle By Name(cluster=T40 {"Command"=enum."Move by", "Data"=variant(dbl[] [])} ("MSG to Servo"), "Command"=Servo_commands."Move by", "Data"=w486) -> (w479:T40)
                        n267 = Unbundle By Name(w478) -> ("Table_C"=w480:refnum<queue>)
                        n268 = call "Put in mailbox.vi"("Message"=w479, "Queue in"=w480) -> ()  [unwired: 7 in, 3 out]
                      }
                    }
                  }
                  event Value Change {
                    w503 = 0.5 ("y")
                    n269 = event-data() -> ("CtlRef"=w495:refnum<vi>)  [unwired: 1 in, 2 out]
                    n270 = Unbundle By Name(w494) -> ("Servo"=w493:T10[])
                    n271 = call "Extract axis properties.vi"("Name"=Axis_names."AxisZ_left", "All servo status"=w493) -> ("Servo"=w502:T10, "Index"=w499:i32)  [unwired: 6 in, 1 out]
                    n272 = Unbundle By Name(w502) -> ("Position"=w498:dbl, "Pos limit"=w500:dbl)
                    n273 = property class="Bool"(reference=w495, "Value"=FALSE) -> ()  [unwired: 1 in, 2 out]
                    n274 = Subtract(x=w500, y=w503) -> (x-y=w504:dbl)
                    n275 = Less?(x=w498, y=w504) -> (x < y?=w505:bool)
                    n276 = case shown="True" w505 {
                      tunnel: w503 -> [_ w516]
                      tunnel: w499 -> [_ w511]
                      tunnel: w497 -> [_ w507]
                      frame False {
                      }
                      frame True {
                        n277 = Initialize Array(0.0 ("element"), 5 ("dimension size")) -> (w515:dbl[])
                        n278 = Replace Array Subset(array=w515, new element=w516, index=w511) -> (w512:dbl[])
                        n279 = Bundle By Name(cluster=T40 {"Command"=enum."Move by", "Data"=variant(dbl[] [])} ("MSG to Servo"), "Command"=Servo_commands."Move by", "Data"=w512) -> (w508:T40)
                        n280 = Unbundle By Name(w507) -> ("Table_C"=w509:refnum<queue>)
                        n281 = call "Put in mailbox.vi"("Message"=w508, "Queue in"=w509) -> ()  [unwired: 7 in, 3 out]
                      }
                    }
                  }
                  event Value Change {
                    w528 = 0.5 ("y")
                    n282 = event-data() -> ("CtlRef"=w520:refnum<vi>)  [unwired: 1 in, 3 out]
                    n283 = Unbundle By Name(w518) -> ("Servo"=w519:T10[])
                    n284 = call "Extract axis properties.vi"("Name"=Axis_names."AxisZ_left", "All servo status"=w519) -> ("Servo"=w527:T10, "Index"=w524:i32)  [unwired: 6 in, 1 out]
                    n285 = Unbundle By Name(w527) -> ("Position"=w523:dbl, "Neg limit"=w525:dbl)
                    n286 = property class="Bool"(reference=w520, "Value"=FALSE) -> ()  [unwired: 1 in, 2 out]
                    n287 = Add(x=w525, y=w528) -> (x+y=w529:dbl)
                    n288 = Greater?(x=w523, y=w529) -> (0:w530:bool)
                    n289 = case shown="True" w530 {
                      tunnel: w528 -> [_ w540]
                      tunnel: w524 -> [_ w536]
                      tunnel: w522 -> [_ w533]
                      frame False {
                      }
                      frame True {
                        n290 = Negate(x=w540) -> (-x=w542:dbl)
                        n291 = Initialize Array(0.0 ("element"), 5 ("dimension size")) -> (w541:dbl[])
                        n292 = Replace Array Subset(array=w541, new element=w542, index=w536) -> (w537:dbl[])
                        n293 = Unbundle By Name(w533) -> ("Table_C"=w534:refnum<queue>)
                        n294 = Bundle By Name(cluster=T40 {"Command"=enum."Move by", "Data"=variant(dbl[] [])} ("MSG to Servo"), "Command"=Servo_commands."Move by", "Data"=w537) -> (w532:T40)
                        n295 = call "Put in mailbox.vi"("Message"=w532, "Queue in"=w534) -> ()  [unwired: 7 in, 3 out]
                      }
                    }
                  }
                  event Value Change {
                    w554 = 0.5 ("y")
                    n296 = event-data() -> ("CtlRef"=w546:refnum<vi>)  [unwired: 1 in, 3 out]
                    n297 = Unbundle By Name(w544) -> ("Servo"=w545:T10[])
                    n298 = call "Extract axis properties.vi"("Name"=Axis_names."AxisZ_right", "All servo status"=w545) -> ("Servo"=w553:T10, "Index"=w550:i32)  [unwired: 6 in, 1 out]
                    n299 = Unbundle By Name(w553) -> ("Position"=w549:dbl, "Pos limit"=w551:dbl)
                    n300 = property class="Bool"(reference=w546, "Value"=FALSE) -> ()  [unwired: 1 in, 2 out]
                    n301 = Subtract(x=w551, y=w554) -> (x-y=w556:dbl)
                    n302 = Less?(x=w549, y=w556) -> (x < y?=w555:bool)
                    n303 = case shown="True" w555 {
                      tunnel: w554 -> [_ w566]
                      tunnel: w550 -> [_ w562]
                      tunnel: w548 -> [_ w558]
                      frame False {
                      }
                      frame True {
                        n304 = Initialize Array(0.0 ("element"), 5 ("dimension size")) -> (w567:dbl[])
                        n305 = Replace Array Subset(array=w567, new element=w566, index=w562) -> (w563:dbl[])
                        n306 = Bundle By Name(cluster=T40 {"Command"=enum."Move by", "Data"=variant(dbl[] [])} ("MSG to Servo"), "Command"=Servo_commands."Move by", "Data"=w563) -> (w559:T40)
                        n307 = Unbundle By Name(w558) -> ("Table_C"=w560:refnum<queue>)
                        n308 = call "Put in mailbox.vi"("Message"=w559, "Queue in"=w560) -> ()  [unwired: 7 in, 3 out]
                      }
                    }
                  }
                  event Value Change {
                    w578 = 0.5 ("y")
                    n309 = event-data() -> ("CtlRef"=w571:refnum<vi>)  [unwired: 1 in, 4 out]
                    n310 = Unbundle By Name(w569) -> ("Servo"=w570:T10[])
                    n311 = call "Extract axis properties.vi"("Name"=Axis_names."AxisZ_right", "All servo status"=w570) -> ("Servo"=w577:T10, "Index"=w575:i32)  [unwired: 6 in, 1 out]
                    n312 = property class="Bool"(reference=w571, "Value"=FALSE) -> ()  [unwired: 1 in, 2 out]
                    n313 = Unbundle By Name(w577) -> ("Position"=w574:dbl, "Neg limit"=w580:dbl)
                    n314 = Add(x=w580, y=w578) -> (x+y=w579:dbl)
                    n315 = Greater?(x=w574, y=w579) -> (0:w581:bool)
                    n316 = case shown="True" w581 {
                      tunnel: w578 -> [_ w591]
                      tunnel: w575 -> [_ w587]
                      tunnel: w573 -> [_ w583]
                      frame False {
                      }
                      frame True {
                        n317 = Negate(x=w591) -> (-x=w593:dbl)
                        n318 = Initialize Array(0.0 ("element"), 5 ("dimension size")) -> (w592:dbl[])
                        n319 = Replace Array Subset(array=w592, new element=w593, index=w587) -> (w588:dbl[])
                        n320 = Unbundle By Name(w583) -> ("Table_C"=w585:refnum<queue>)
                        n321 = Bundle By Name(cluster=T40 {"Command"=enum."Move by", "Data"=variant(dbl[] [])} ("MSG to Servo"), "Command"=Servo_commands."Move by", "Data"=w588) -> (w584:T40)
                        n322 = call "Put in mailbox.vi"("Message"=w584, "Queue in"=w585) -> ()  [unwired: 7 in, 3 out]
                      }
                    }
                  }
                  event Value Change {
                    w605 = 0.5 ("y")
                    n323 = event-data() -> ("CtlRef"=w597:refnum<vi>)  [unwired: 1 in, 3 out]
                    n324 = Unbundle By Name(w595) -> ("Servo"=w596:T10[])
                    n325 = call "Extract axis properties.vi"("Name"=Axis_names."AxisZ_middle", "All servo status"=w596) -> ("Servo"=w604:T10, "Index"=w601:i32)  [unwired: 6 in, 1 out]
                    n326 = Unbundle By Name(w604) -> ("Position"=w600:dbl, "Pos limit"=w602:dbl)
                    n327 = property class="Bool"(reference=w597, "Value"=FALSE) -> ()  [unwired: 1 in, 2 out]
                    n328 = Subtract(x=w602, y=w605) -> (x-y=w606:dbl)
                    n329 = Less?(x=w600, y=w606) -> (x < y?=w607:bool)
                    n330 = case shown="True" w607 {
                      tunnel: w605 -> [_ w617]
                      tunnel: w601 -> [_ w613]
                      tunnel: w599 -> [_ w609]
                      frame False {
                      }
                      frame True {
                        n331 = Initialize Array(0.0 ("element"), 5 ("dimension size")) -> (w618:dbl[])
                        n332 = Replace Array Subset(array=w618, new element=w617, index=w613) -> (w614:dbl[])
                        n333 = Bundle By Name(cluster=T40 {"Command"=enum."Move by", "Data"=variant(dbl[] [])} ("MSG to Servo"), "Command"=Servo_commands."Move by", "Data"=w614) -> (w610:T40)
                        n334 = Unbundle By Name(w609) -> ("Table_C"=w611:refnum<queue>)
                        n335 = call "Put in mailbox.vi"("Message"=w610, "Queue in"=w611) -> ()  [unwired: 7 in, 3 out]
                      }
                    }
                  }
                  event Value Change {
                    w630 = 0.5 ("y")
                    n336 = event-data() -> ("CtlRef"=w622:refnum<vi>)  [unwired: 1 in, 3 out]
                    n337 = Unbundle By Name(w620) -> ("Servo"=w621:T10[])
                    n338 = call "Extract axis properties.vi"("Name"=Axis_names."AxisZ_middle", "All servo status"=w621) -> ("Servo"=w628:T10, "Index"=w626:i32)  [unwired: 6 in, 1 out]
                    n339 = Unbundle By Name(w628) -> ("Position"=w625:dbl, "Neg limit"=w627:dbl)
                    n340 = property class="Bool"(reference=w622, "Value"=FALSE) -> ()  [unwired: 1 in, 2 out]
                    n341 = Add(x=w627, y=w630) -> (x+y=w631:dbl)
                    n342 = Greater?(x=w625, y=w631) -> (0:w632:bool)
                    n343 = case shown="True" w632 {
                      tunnel: w630 -> [_ w642]
                      tunnel: w626 -> [_ w638]
                      tunnel: w624 -> [_ w635]
                      frame False {
                      }
                      frame True {
                        n344 = Negate(x=w642) -> (-x=w644:dbl)
                        n345 = Initialize Array(0.0 ("element"), 5 ("dimension size")) -> (w643:dbl[])
                        n346 = Replace Array Subset(array=w643, new element=w644, index=w638) -> (w639:dbl[])
                        n347 = Unbundle By Name(w635) -> ("Table_C"=w636:refnum<queue>)
                        n348 = Bundle By Name(cluster=T40 {"Command"=enum."Move by", "Data"=variant(dbl[] [])} ("MSG to Servo"), "Command"=Servo_commands."Move by", "Data"=w639) -> (w634:T40)
                        n349 = call "Put in mailbox.vi"("Message"=w634, "Queue in"=w636) -> ()  [unwired: 7 in, 3 out]
                      }
                    }
                  }
                  event Value Change {
                    n350 = event-data() -> ("CtlRef"=w647:refnum<vi>)  [unwired: 1 in, 3 out]
                    n351 = Unbundle By Name(w665) -> ("Magnet.PSU"=w664:string, "Magnet.Field [T]"=w663:dbl)
                    n352 = Unbundle By Name(w652) -> ("Angle_C"=w651:refnum<queue>)
                    n353 = property class="Bool (strict)"(reference=w647, "Value"=FALSE) -> ()  [unwired: 1 in, 2 out]
                    n354 = local read "Rotator controls"() -> (w655:T15)
                    n355 = Less?(x=w663, y=8.0) -> (x < y?=w660:bool)
                    n356 = Not Equal?(x="", y=w664) -> (x != y?=w659:bool)
                    n357 = And(x=w659, y=w660) -> (x .and. y?=w658:bool)
                    n358 = Select(t=TRUE, s=w658, f=FALSE ("x .and. y?")) -> (s? t:f=w653:bool)
                    n359 = Unbundle By Name(w655) -> ("Set position"=w654:T17)
                    n360 = Bundle By Name(cluster=w654, "Safe to move?"=w653) -> (w648:T17)
                    n361 = Bundle By Name(cluster=T41 {"Command"=enum."Set position", "Data"=variant} ("MSG to rotator"), "Data"=w648) -> (w649:T41)
                    n362 = call "Put in mailbox.vi"("Message"=w649, "Queue in"=w651) -> ()  [unwired: 7 in, 3 out]
                  }
                  event Value Change {
                    n363 = event-data() -> ()  [unwired: 1 in, 5 out]
                    n364 = Unbundle By Name(w675) -> ("Angle_C"=w674:refnum<queue>)
                    n365 = Unbundle By Name("Rotator controls") -> ("Motion properties"=w673:T16)
                    n366 = Unbundle By Name(w673) -> ("DC voltage [V]"=w668:dbl)
                    n367 = Greater Than 0?(x=w668) -> (x > 0?=w672:bool)
                    n368 = case shown="True" w672 {
                      tunnel: [_ w680] -> w670
                      frame False {
                      }
                      frame True {
                        n369 = Two Button Dialog(message="DC Voltage is not zero.\nDo you realy want to set it?") -> (T button?=w680:bool)  [unwired: 2 in]
                      }
                    }
                    n370 = Select(t=w668, s=w670, f=0.0) -> (s? t:f=w669:dbl)
                    n371 = Bundle By Name(cluster=w673, "DC voltage [V]"=w669) -> (w671:T16)
                    n372 = Bundle By Name(cluster=T41 {"Command"=enum."Set parameters", "Data"=variant} ("MSG to rotator"), "Data"=w671) -> (w676:T41)
                    n373 = call "Put in mailbox.vi"("Message"=w676, "Queue in"=w674) -> ()  [unwired: 7 in, 3 out]
                  }
                  event Value Change {
                    n374 = event-data() -> ("CtlRef"=w686:refnum<vi>)  [unwired: 1 in, 3 out]
                    n375 = Unbundle By Name(w684) -> ("Angle_C"=w683:refnum<queue>)
                    n376 = property class="Bool (strict)"(reference=w686, "Value"=FALSE) -> ()  [unwired: 1 in, 2 out]
                    n377 = call "Put in mailbox.vi"("Message"=T41 {"Command"=enum."Stop movement", "Data"=variant} ("MSG to rotator"), "Queue in"=w683) -> ()  [unwired: 7 in, 3 out]
                  }
                  event Value Change {
                    n378 = event-data() -> ()  [unwired: 1 in, 6 out]
                    n379 = Unbundle By Name("THz control") -> ("AMC"=w698:u16, "Multip"=w697:u16, "Base frequency [GHz]"=w705:dbl, "End frequency [GHz]"=w706:dbl, "Im frequency [MHz]"=w707:dbl, "Sweep up [ms]"=w691:dbl, "Reset trigger?"=w690:bool)
                    n380 = Unbundle By Name(w700) -> ("MW_C"=w699:refnum<queue>)
                    n381 = Multiply(x=w698, y=w697) -> (x*y=w693:u16)
                    n382 = Divide(x=w705, y=w693) -> (x/y=w696:dbl)
                    n383 = Divide(x=w706, y=w693) -> (x/y=w695:dbl)
                    n384 = Divide(x=w691, y=2.0) -> (x/y=w689:dbl)
                    n385 = Divide(x=w707, y=w693) -> (x/y=w694:dbl)
                    n386 = Bundle By Name(cluster=T44 {"Start [GHz]"=8.0, "End [GHz] "=8.0, "Sweep up\ntime [ms]"=0.0, "Sweep down\ntime [ms]"=0.0, "Intermidiate [MHz]"=0.0, "Reset trigger"=FALSE} ("Sweep parameters"), "Start [GHz]"=w696, "End [GHz]"=w695, "Intermidiate [MHz]"=w694, "Sweep up\ntime [ms]"=w691, "Sweep down\ntime [ms]"=w689, "Reset trigger"=w690) -> (w702:T44)
                    n387 = Bundle By Name(cluster=T45 {"Command"=enum."Set parameters", "Data"=variant} ("Incoming msg"), "Command"=THz_commands_enum."Set parameters", "Data"=w702) -> (w703:T45)
                    n388 = call "Put in mailbox.vi"("Message"=w703, "Queue in"=w699) -> ()  [unwired: 7 in, 3 out]
                  }
                  event Value Change {
                    n389 = event-data() -> ()  [unwired: 1 in, 6 out]
                    n390 = local read "THz control"() -> (w717:T22)
                    n391 = Unbundle By Name(w717) -> ("AMC"=w714:u16, "Multip"=w713:u16)
                    n392 = Multiply(x=w714, y=w713) -> (x*y=w712:u16)
                    n393 = Multiply(x=14.0, y=w712) -> (x*y=w711:dbl)
                    n394 = Multiply(x=0.01, y=w712) -> (x*y=w710:dbl)
                    n395 = property on="End frequency [GHz]" class="DigNum (strict)"("Minimum"=w710, "Maximum"=w711) -> ()  [unwired: 2 in, 2 out]
                    n396 = property on="Base frequency [GHz]" class="DigNum (strict)"("Minimum"=w710, "Maximum"=w711) -> ()  [unwired: 2 in, 2 out]
                  }
                  event Value Change {
                    n397 = event-data() -> ("CtlRef"=w725:refnum<vi>, "NewVal"=w722:dbl)  [unwired: 1 in]
                    n398 = Unbundle By Name(w732) -> ("Data_Aq"=w731:refnum<queue>)
                    n399 = property class="DigNum (strict)"(reference=w725) -> ("Label.Text"=w724:string)  [unwired: 1 in, 2 out]
                    n400 = case shown="\"Amp_Mod [mV]\"" w724 {
                      tunnel: [MFLI_node."None" ("parameter") MFLI_node."filter_constant [ms]" ("parameter") MFLI_node."filter_order [-]" ("parameter") MFLI_node."osc_freq [kHz]" ("parameter") MFLI_node."Phase_deg" ("parameter") MFLI_node."out_ampl [V]" ("parameter")] -> w720
                      tunnel: w722 -> [_ w736 w738 w740 w742 w746]
                      tunnel: [_ w736 w738 w740 w742 w758] -> w723
                      tunnel: "Acquisition controls" -> [_ _ _ _ _ w756]
                      tunnel: [_ _ _ _ _ w744] -> _
                      frame "Unknown", Default {
                      }
                      frame "Time constant [ms]" {
                      }
                      frame "Filter order" {
                      }
                      frame "F_Mod [kHz]" {
                      }
                      frame "Phase [°]" {
                      }
                      frame "Amp_Mod [mV]" {
                        n401 = Unbundle By Name(w756) -> ("ACQ parameters.F_Mod [kHz]"=w753:dbl, "Sample holder"=w743:T20)
                        n402 = case shown="\"Carousel\"" w743 {
                          tunnel: [w762 w765 w768 w771] -> w755
                          tunnel: [w761 w764 w767 w770] -> w751
                          tunnel: [w760 w763 w766 w769] -> w745
                          frame "Simple", Default {
                            w760 = 0.0  # G/A
                            w761 = 8.9  # R
                            w762 = 0.0017  # L
                          }
                          frame "Carousel" {
                            w763 = 0.0  # G/A
                            w764 = 8.9  # R
                            w765 = 0.0017  # L
                          }
                          frame "Chip" {
                            w766 = 0.0  # G/A
                            w767 = 8.9  # R
                            w768 = 0.0017  # L
                          }
                          frame "Rotator" {
                            w769 = 0.0  # G/A
                            w770 = 8.9  # R
                            w771 = 0.0017  # L
                          }
                        }
                        n403 = Divide(x=w746, y=1000.0) -> (x/y=w758:dbl)
                        n404 = Square(x=w751) -> (x^2=w749:dbl)
                        n405 = Compound Arithmetic op=MULTIPLY(w753, 6.283185307179586, w755) -> (w752:dbl)
                        n406 = Square(x=w752) -> (x^2=w750:dbl)
                        n407 = Add(x=w750, y=w749) -> (x+y=w748:dbl)
                        n408 = Square Root(x=w748) -> (sqrt(x)=w747:dbl)
                        n409 = Compound Arithmetic op=MULTIPLY(w745, w747) -> (w744:dbl)
                      }
                    }
                    n410 = Bundle(cluster=T46 {"parameter"=enum."filter_order [-]", "value"=0.0} ("Parameter to set"), "parameter"=w720, "value"=w723) -> (w726:T46)
                    n411 = Build Array(w726) -> (w721:T46[])
                    n412 = Bundle By Name(cluster=T49 {"Command"=enum."Initialize", "Data"=variant} ("MSG for  ACQ"), "Command"=MFLI_command_enum."Set individual parameters", "Data"=w721) -> (w728:T49)
                    n413 = call "Put in mailbox.vi"("Message"=w728, "Queue in"=w731) -> ()  [unwired: 7 in, 3 out]
                  }
                  event Value Change {
                    w775 = T46 {"parameter"=enum."filter_order [-]", "value"=0.0} ("Parameter to set")
                    n414 = event-data() -> ("NewVal"=w773:u16)  [unwired: 1 in, 2 out]
                    n415 = Unbundle By Name(w783) -> ("Data_Aq"=w782:refnum<queue>)
                    n416 = Bundle(cluster=w775, "parameter"=MFLI_node."enable output", "value"=w773) -> (w778:T46)
                    n417 = Bundle(cluster=w775, "parameter"=MFLI_node."enamble ampl", "value"=w773) -> (w772:T46)
                    n418 = Build Array(w778, w772) -> (w777:T46[])
                    n419 = Bundle By Name(cluster=T49 {"Command"=enum."Initialize", "Data"=variant} ("MSG for  ACQ"), "Command"=MFLI_command_enum."Set individual parameters", "Data"=w777) -> (w779:T49)
                    n420 = call "Put in mailbox.vi"("Message"=w779, "Queue in"=w782) -> ()  [unwired: 7 in, 3 out]
                  }
                  event "Acquisition controls.Autorange": Value Change {
                    n421 = event-data() -> ("CtlRef"=w792:refnum<vi>)  [unwired: 1 in, 3 out]
                    n422 = Unbundle By Name(w790) -> ("Data_Aq"=w789:refnum<queue>)
                    n423 = property class="Bool (strict)"(reference=w792, "Value"=FALSE) -> ()  [unwired: 1 in, 2 out]
                    n424 = Build Array(T46 {"parameter"=enum."in_autorange", "value"=1.0} ("Parameter to set")) -> (w786:T46[])
                    n425 = Bundle By Name(cluster=T49 {"Command"=enum."Set individual parameters", "Data"=variant} ("MSG for  ACQ"), "Data"=w786) -> (w785:T49)
                    n426 = call "Put in mailbox.vi"("Message"=w785, "Queue in"=w789) -> ()  [unwired: 7 in, 3 out]
                  }
                  event Value Change {
                    n427 = event-data() -> ("CtlRef"=w799:refnum<vi>, "NewVal"=w797:dbl)  [unwired: 1 in]
                    n428 = property class="DigNum (strict)"(reference=w799) -> ("Label.Text"=w798:string)  [unwired: 1 in, 2 out]
                    n429 = Unbundle By Name(w803) -> ("Tmp_C"=w800:refnum<queue>)
                    n430 = Bundle(cluster=T50 {"Heater"="None", "Tmp [K]"=0.0} ("Set point"), "Heater"=w798, "Tmp [K]"=w797) -> (w794:T50)
                    n431 = Bundle By Name(cluster=T52 {"Command"=enum."Initialize", "Data"=variant}, "Command"=TC_commands."Set point", "Data"=w794) -> (w801:T52)
                    n432 = call "Put in mailbox.vi"("Message"=w801, "Queue in"=w800) -> ()  [unwired: 7 in, 3 out]
                  }
                  event "SMU controls.Apply": Value Change {
                    n433 = event-data() -> ()  [unwired: 1 in, 5 out]
                    n434 = Unbundle By Name(w808) -> ("Field_M"=w810:refnum<queue>)
                    n435 = Bundle By Name(cluster="SMU controls", "Apply"=FALSE) -> (w809:T14)
                    n436 = Unbundle By Name(w809) -> ("Measurement settings"=w805:T13)
                    n437 = local write "SMU controls"(w809) -> ()
                    n438 = Bundle By Name(cluster=T53 {"Command"=enum."Set measurement", "Data"=variant} ("MSG to Source meter"), "Data"=w805) -> (w806:T53)
                    n439 = call "Put in mailbox.vi"("Message"=w806, "Queue in"=w810) -> ()  [unwired: 7 in, 3 out]
                  }
                  event "SMU controls.Record": Value Change {
                    n440 = event-data() -> ()  [unwired: 1 in, 6 out]
                    n441 = local read "SMU controls"() -> (w819:T14)
                    n442 = Unbundle By Name(w814) -> ("Field_M"=w816:refnum<queue>)
                    n443 = Bundle By Name(cluster=w819, "Record"=FALSE ("Apply")) -> (w818:T14)
                    n444 = call "Put in mailbox.vi"("Message"=T53 {"Command"=enum."Start measurement", "Data"=variant} ("MSG to Source meter"), "Queue in"=w816) -> ()  [unwired: 7 in, 3 out]
                    n445 = local write "SMU controls"(w818) -> ()
                  }
                  event "SMU controls.Stop": Value Change {
                    n446 = event-data() -> ()  [unwired: 1 in, 6 out]
                    n447 = Unbundle By Name(w823) -> ("Field_M"=w822:refnum<queue>)
                    n448 = local read "SMU controls"() -> (w826:T14)
                    n449 = call "Put in mailbox.vi"("Message"=T53 {"Command"=enum."Stop measurement", "Data"=variant} ("MSG to Source meter"), "Queue in"=w822) -> ()  [unwired: 7 in, 3 out]
                    n450 = Bundle By Name(cluster=w826, "Stop"=FALSE ("Apply")) -> (w825:T14)
                    n451 = local write "SMU controls"(w825) -> ()
                  }
                  event "Password": Value Change {
                    n452 = event-data() -> ("NewVal"=w832:string)  [unwired: 1 in, 1 out]
                    n453 = Equal?(x="admin", y=w832) -> (x = y?=w828:bool)
                    n454 = case shown="False" w828 {
                      tunnel: [T34."Disabled and Grayed Out" ("Disabled") T34."Enabled" ("Disabled")] -> w829
                      frame False {
                      }
                      frame True {
                      }
                    }
                    n455 = local read "Instr control refs"() -> (w830:refnum<vi>[])
                    n456 = call "Dis- or en- able controls.vi"("Disabled"=w829, "Control referencies"=w830) -> ()  [unwired: 9 in, 1 out]
                  }
                }
              }
              frame "EPR measurement" {
                n457 = event shown="[1] \"Run script btn\": Value Change" {
                  selector: _ -> [_ _ _ _ _ _]
                  dyn-events: _ -> [_ _ _ _ _ _]
                  timeout: 0 -> [_ _ _ _ _ _]
                  tunnel: w843 -> [w846 w865 w896 w928 w966 w972]
                  tunnel: [w846 w864 w896 w928 w966 w972] -> w842
                  tunnel: w840 -> [_ _ w895 _ _ _]
                  tunnel: [w844 w860 w892 w927 w963 w971] -> w839
                  tunnel: w838 -> [w844 w857 w892 w927 w963 w971]
                  tunnel: [w845 w861 w891 w926 w962 w970] -> w836
                  tunnel: w837 -> [w845 w862 w890 w926 w962 w970]
                  event Timeout {
                    n458 = event-data() -> ()  [unwired: 1 in, 3 out]
                  }
                  event "Run script btn": Value Change {
                    n459 = event-data() -> ()  [unwired: 1 in, 6 out]
                    n460 = local read "Script Array"() -> (w863:T27[])
                    n461 = local read "THz control"() -> (w855:T22)
                    n462 = Unbundle By Name(w855) -> ("AMC"=w853:u16, "Multip"=w854:u16)
                    n463 = Multiply(x=w853, y=w854) -> (x*y=w852:u16)
                    n464 = for {
                      tunnel: w863 -> [w870] mode=indexing
                      tunnel: [w869] -> w859
                      tunnel: [w870] -> w858
                      tunnel: [w868] -> w856
                      tunnel: w852 -> [w867]
                      tunnel: [w866] -> w850
                      i -> [w868]
                      stop <- w869 stop-if-true
                      n465 = local read "Instr status"() -> (w871:T1)
                      n466 = call "verify executabiity of line.vi"("Freq multiplication factor"=w867, "Instr status"=w871, "Script cluster"=w870) -> ("Response"=w866:string, "is executable"=w869:bool)  [unwired: 7 in]
                    }
                    n467 = One Button Dialog(message="Absorbers!!!", button name ("OK")="OK, run measurement!") -> (true=w849:bool)
                    n468 = case shown="False" w859 {
                      tunnel: w862 -> [w876 w885]
                      tunnel: [w876 w884] -> w861
                      tunnel: [w875 w882] -> w860
                      tunnel: w858 -> [_ w882]
                      tunnel: w857 -> [w875 _]
                      tunnel: w856 -> [_ w880]
                      tunnel: [w873 w878] -> w851
                      tunnel: w850 -> [w874 _]
                      tunnel: w849 -> [_ _]
                      frame False {
                        n469 = Concatenate Strings("Line is not executable beause:" ("string"), w874) -> (w873:string)
                      }
                      frame True {
                        n470 = local read "Controls referencies"() -> (w886:T2)
                        n471 = Unbundle By Name(w886) -> ("To disable"=w877:refnum<vi>[])
                        n472 = Build Array(w880) -> (w881:i32[])
                        n473 = Bundle By Name(cluster=w885, "Experiment state"=experiment_state."Preparation" ("Value")) -> (w884:T25)
                        n474 = Format Into String(format string="%d sctrip lines skipped", w880) -> (resulting string=w878:string)  [unwired: 2 in, 1 out]
                        n475 = property on="Script Array" class="Arr (strict)"("Selection Start []"=w881) -> ()  [unwired: 2 in, 2 out]
                        n476 = call "Dis- or en- able controls.vi"("Disabled"=T34."Disabled and Grayed Out", "Control referencies"=w877) -> ()  [unwired: 9 in, 1 out]
                      }
                    }
                    n477 = call "simple Shift string array.vi"("Element in"=w851, "Array in"=w865) -> ("Array out"=w864:string[])  [unwired: 8 in, 1 out]
                  }
                  event "Direct stop meas. btn": Value Change {
                    n478 = event-data() -> ("NewVal"=w894:bool)  [unwired: 1 in, 5 out]
                    n479 = call "Timeout dialoge Abbort.vi"("Enable"=w894, "Message to Display"="Realy abbort measurement?", "timeout[ms]"=u32 5000) -> ("Yes"=w893:bool)  [unwired: 15 in, 1 out]
                    n480 = case shown="True" w893 {
                      tunnel: w895 -> [_ w914]
                      tunnel: w890 -> [w897 w901]
                      tunnel: [w897 w900] -> w891
                      frame False {
                      }
                      frame True {
                        n481 = Unbundle By Name(w914) -> ("Field_C"=w908:refnum<queue>, "Tmp_C"=w909:refnum<queue>, "Angle_C"=w910:refnum<queue>)
                        n482 = local read "Controls referencies"() -> (w903:T2)
                        n483 = local write "Run script btn"(FALSE ("Direct stop meas. btn")) -> ()
                        n484 = Bundle By Name(cluster=w901, "Experiment state"=experiment_state."Save" ("Value")) -> (w900:T25)
                        n485 = Unbundle By Name(w903) -> ("To disable"=w904:refnum<vi>[])
                        n486 = call "Put in mailbox.vi"("Message"=T38 {"Order"=enum."Stop ramping", "Data"=variant} ("MSG to magnet"), "Queue in"=w908) -> ("error out"=w907:errorcluster)  [unwired: 7 in, 2 out]
                        n487 = call "Put in mailbox.vi"("error in (no error)"=w907, "Message"=T52 {"Command"=enum."Stop tmp change", "Data"=variant} ("MSG for VTI"), "Queue in"=w909) -> ("error out"=w906:errorcluster)  [unwired: 6 in, 2 out]
                        n488 = call "Put in mailbox.vi"("error in (no error)"=w906, "Message"=T41 {"Command"=enum."Stop movement", "Data"=variant} ("MSG to rotator"), "Queue in"=w910) -> ("error out"=w898:errorcluster)  [unwired: 6 in, 2 out]
                        n489 = call "Dis- or en- able controls.vi"("error in"=w898, "Disabled"=T34."Enabled", "Control referencies"=w904) -> ()  [unwired: 8 in, 1 out]
                      }
                    }
                  }
                  event "Script Array": Value Change {
                    # "Verification of values"
                    n490 = event-data() -> ("OldVal"=w921:T27[], "NewVal"=w920:T27[])  [unwired: 1 in, 2 out]
                    n491 = local read "THz control"() -> (w919:T22)
                    n492 = Unbundle By Name(w919) -> ("AMC"=w917:u16, "Multip"=w918:u16)
                    n493 = Array Size(array=w920) -> (size(s)=w924:i32)
                    n494 = Array Size(array=w921) -> (size(s)=w923:i32)
                    n495 = Multiply(x=w917, y=w918) -> (x*y=w916:u16)
                    n496 = Equal?(x=w923, y=w924) -> (x = y?=w922:bool)
                    n497 = case shown="False" w922 {
                      tunnel: w921 -> [w933 w951]
                      tunnel: w920 -> [w934 w950]
                      tunnel: [w932 w949] -> w915
                      tunnel: w923 -> [w935 _]
                      tunnel: w924 -> [w936 _]
                      tunnel: T55 {"min synth f"=9.0, "max synth f"=14.0, "Ramp limits [mT/s]"=[7.5, 5.5, 4.2, 3.1, 1.5], "Field ranges [T]"=[3.0, 9.6, 13.3, 15.5, 16.0]} ("Limits") -> [w930 w948]
                      tunnel: w916 -> [w929 w947]
                      frame False {
                        n498 = Greater?(x=w935, y=w936) -> (0:w931:bool)
                        n499 = case shown="False" w931 {
                          tunnel: w934 -> [w937 w942]
                          tunnel: [w937 w938] -> w932
                          tunnel: w933 -> [_ w940]
                          tunnel: w930 -> [_ w945]
                          tunnel: w929 -> [_ w944]
                          frame True {
                          }
                          frame False {
                            n500 = Reverse 1D Array(array=w942) -> (reversed array=w943:T27[])
                            n501 = Index Array(array=w943) -> (element=w941:T27)  [unwired: 1 in]
                            n502 = call "Check polymorh script.vi"("Multipl factor"=w944, "Limits"=w945, "New val"=w941, "Old val"=T27 {"Start"=0.0, "Start Caption"="Start [T]", "End"=0.0, "End Caption"="End [T]", "Sweep"=0.0, "Sweep caption"="Rate [mT/s]", "Constant"=-1.0, "Constant caption"="Freq [GHz]", "Mod_F [kHz]"=0.1, "Mod_A [G]"=0.0, "Tau [ms]"=0.0, "Angle [°]"=0.0, "Tmp [K]"=0.0, "Wait [min]"=0.0, "Carousel"=-1, "Comment"="", "Auto-mod"=TRUE, "Execute"=FALSE} ("Old Row")) -> ("Row out"=w939:T27)  [unwired: 7 in]
                            n503 = Insert Into Array(array=w940, new element=w939) -> (w938:T27[])  [unwired: 1 in]
                          }
                        }
                      }
                      frame True {
                        n504 = for {
                          tunnel: w951 -> [w956] mode=indexing
                          tunnel: w950 -> [w955] mode=indexing
                          tunnel: [w954] -> w949 mode=indexing
                          tunnel: w948 -> [w953]
                          tunnel: w947 -> [w952]
                          n505 = call "Check polymorh script.vi"("Multipl factor"=w952, "Limits"=w953, "New val"=w955, "Old val"=w956) -> ("Row out"=w954:T27)  [unwired: 7 in]
                        }
                      }
                    }
                    n506 = local write "Script Array"(w915) -> ()
                  }
                  event "Sample name", "Global comment": Value Change {
                    n507 = event-data() -> ("CtlRef"=w961:refnum<vi>, "NewVal"=w965:string)  [unwired: 1 in, 4 out]
                    n508 = Search and Replace String(replace all?=TRUE ("replace all? (F)"), input string=w965, search string="[<>:\"/\\|?*%]" ("regular expression"), replace string="-" ("replace string (\"\")")) -> (result string=w959:string)  [unwired: 4 in, 3 out]
                    n509 = call <vilib>:"Space Constant.vi"() -> ("String"=w958:string)
                    n510 = Search and Replace String(input string=w959, search string="\r\n", replace string=w958) -> (result string=w960:string)  [unwired: 5 in, 3 out]
                    n511 = property class="Str"(reference=w961, "Value"=w960) -> ()  [unwired: 1 in, 2 out]
                  }
                  event "Paste from Editor": Value Change {
                    n512 = event-data() -> ()  [unwired: 1 in, 6 out]
                    n513 = local read "Edited script"() -> (w969:T27[])
                    n514 = local write "Script Array"(w969) -> ()
                  }
                }
              }
              frame "Script Editor" {
                n515 = event shown="[8] \"Edited script\": Value Change" {
                  selector: _ -> [_ _ _ _ _ _ _ _ _ _ _]
                  dyn-events: _ -> [_ _ _ _ _ _ _ _ _ _ _]
                  timeout: 0 -> [_ _ _ _ _ _ _ _ _ _ _]
                  event Timeout {
                    n516 = event-data() -> ()  [unwired: 1 in, 3 out]
                  }
                  event "Generate Script btn": Value Change {
                    n517 = event-data() -> ()  [unwired: 1 in, 4 out]
                    n518 = local read "Edited script"() -> (w980:T27[])
                    n519 = call "Generate script array elements.vi"("Script in"=w980, "Generator options"="Generator options", "Prototype line"="Prototype line") -> ("Script out"=w979:T27[])  [unwired: 2 in]
                    n520 = Array Size(array=w979) -> (size(s)=w983:i32)
                    n521 = case shown="1, Default" w983 {
                      selector: w983 -> [w984 w986]
                      tunnel: [w984 w985] -> w982
                      tunnel: [w984 w987] -> w981
                      frame 0 {
                      }
                      frame 1, Default {
                        n522 = Decrement(x=w986) -> (x-1=w985:i32)
                        n523 = Negate(x=w986) -> (-x=w987:i32)
                      }
                    }
                    n524 = local write "Edited script"(w979) -> ()
                    n525 = property on="Select\nline" class="DigNum (strict)"("Maximum"=w982, "Minimum"=w981) -> ()  [unwired: 2 in, 2 out]
                  }
                  event "Load script btn": Value Change {
                    n526 = event-data() -> ()  [unwired: 1 in, 3 out]
                    n527 = local read "THz control"() -> (w992:T22)
                    n528 = call "Load script file.vi"() -> ("Array"=w988:T27[], "Multiplication factor"=w989:i32)  [unwired: 10 in]
                    n529 = Unbundle By Name(w992) -> ("AMC"=w993:u16, "Multip"=w994:u16)
                    n530 = Array Size(array=w988) -> (size(s)=w995:i32)
                    n531 = Multiply(x=w993, y=w994) -> (x*y=w990:u16)
                    n532 = Greater Than 0?(x=w995) -> (x > 0?=w998:bool)
                    n533 = Not Equal?(x=w990, y=w989) -> (x != y?=w991:bool)
                    n534 = case shown="True" w998 {
                      tunnel: w988 -> [_ w1008]
                      frame False {
                      }
                      frame True {
                        n535 = local write "Edited script"(w1008) -> ()
                      }
                    }
                    n536 = case shown="1, Default" w995 {
                      selector: w995 -> [w1004 w1006]
                      tunnel: [w1004 w1005] -> w997
                      tunnel: [w1004 w1007] -> w996
                      frame 0 {
                      }
                      frame 1, Default {
                        n537 = Decrement(x=w1006) -> (x-1=w1005:i32)
                        n538 = Negate(x=w1006) -> (-x=w1007:i32)
                      }
                    }
                    n539 = case shown="True" w991 {
                      tunnel: w990 -> [_ w1001]
                      tunnel: w989 -> [_ w1000]
                      frame False {
                      }
                      frame True {
                        n540 = Format Into String(format string="Actual multiplication factor is %d, but in script is %d.", initial string="Warning!\n", w1001, w1000) -> (resulting string=w999:string)  [unwired: 1 in, 1 out]
                        n541 = One Button Dialog(message=w999) -> ()  [unwired: 1 in, 1 out]
                      }
                    }
                    n542 = property on="Select\nline" class="DigNum (strict)"("Maximum"=w997, "Minimum"=w996) -> ()  [unwired: 2 in, 2 out]
                  }
                  event "Remove from script btn": Value Change {
                    n543 = event-data() -> ()  [unwired: 1 in, 6 out]
                    n544 = local read "Edited script"() -> (w1020:T27[])
                    n545 = local read "Select\nline"() -> (w1010:i32)
                    n546 = Decrement(x=w1010) -> (x-1=w1009:i32)
                    n547 = Array Size(array=w1020) -> (size(s)=w1018:i32)
                    n548 = Build Array(w1009) -> (w1011:i32[])
                    n549 = Add(x=w1018, y=w1010) -> (x+y=w1017:i32)
                    n550 = Less Than 0?(x=w1010) -> (x < 0?=w1019:bool)
                    n551 = local write "Select\nline"(w1009) -> ()
                    n552 = Select(t=w1017, s=w1019, f=w1010) -> (s? t:f=w1016:i32)
                    n553 = property on="Edited script" class="Arr (strict)"("Selection Start []"=w1011) -> ()  [unwired: 2 in, 2 out]
                    n554 = Delete From Array(array=w1020, index=w1016) -> (array with subset deleted=w1012:T27[])  [unwired: 1 in, 1 out]
                    n555 = Array Size(array=w1012) -> (size(s)=w1013:i32)
                    n556 = local write "Edited script"(w1012) -> ()
                    n557 = case shown="1, Default" w1013 {
                      selector: w1013 -> [w1021 w1023]
                      tunnel: [w1021 w1022] -> w1015
                      tunnel: [w1021 w1024] -> w1014
                      frame 0 {
                      }
                      frame 1, Default {
                        n558 = Decrement(x=w1023) -> (x-1=w1022:i32)
                        n559 = Negate(x=w1023) -> (-x=w1024:i32)
                      }
                    }
                    n560 = property on="Select\nline" class="DigNum (strict)"("Maximum"=w1015, "Minimum"=w1014) -> ()  [unwired: 2 in, 2 out]
                  }
                  event "Clear script btn": Value Change {
                    n561 = event-data() -> ()  [unwired: 1 in, 6 out]
                    n562 = local write "Edited script"(T27[] [] ("Edited script")) -> ()
                  }
                  event "Set as adj tab btn": Value Change {
                    n563 = event-data() -> ()  [unwired: 1 in, 4 out]
                    n564 = local read "Acquisition controls"() -> (w1030:T21)
                    n565 = local read "Magnet controls"() -> (w1034:T24)
                    n566 = local read "THz control"() -> (w1032:T22)
                    n567 = Unbundle By Name(w1032) -> ("Base frequency [GHz]"=w1031:dbl)
                    n568 = Unbundle By Name(w1030) -> ("ACQ parameters.F_Mod [kHz]"=w1027:dbl, "ACQ parameters.Filter tau [ms]"=w1028:dbl, "Desired [G]"=w1029:dbl, "Auto-modulation"=w1026:bool)
                    n569 = Unbundle By Name(w1034) -> ("Set Field [T]"=w1033:dbl)
                    n570 = Bundle By Name(cluster=T27 {"Start"=0.0, "Start Caption"="Start [T]", "End"=0.0, "End Caption"="End [T]", "Sweep"=3.0, "Sweep caption"="Rate [mT/s]", "Constant"=210.0, "Constant caption"="Freq [GHz]", "Mod_F [kHz]"=69.1, "Mod_A [G]"=1.0, "Tau [ms]"=100.0, "Angle [°]"=-1.0, "Tmp [K]"=2.0, "Wait [min]"=0.1, "Carousel"=0, "Comment"="No comment", "Auto-mod"=TRUE, "Execute"=TRUE} ("Prototype line"), "Start"=w1033, "Constant"=w1031, "Mod_F [kHz]"=w1027, "Tau [ms]"=w1028, "Mod_A [G]"=w1029, "Auto-mod"=w1026) -> (w1035:T27)
                    n571 = local write "Prototype line"(w1035) -> ()
                  }
                  event "Select\nline": Value Change {
                    n572 = event-data() -> ("CtlRef"=w1037:refnum<vi>)  [unwired: 1 in, 5 out]
                    n573 = Less Than 0?(x="Select\nline") -> (x < 0?=w1042:bool)
                    n574 = case shown="False" w1042 {
                      tunnel: "Select\nline" -> [w1044 w1045]
                      tunnel: w1037 -> [_ w1050]
                      tunnel: [w1044 w1048] -> w1039
                      frame False {
                      }
                      frame True {
                        n575 = property class="DigNum (strict)"(reference=w1050) -> ("Maximum"=w1049:dbl)  [unwired: 1 in, 2 out]
                        n576 = To Long Integer(number=w1049) -> (32bit integer=w1047:i32)
                        n577 = Increment(x=w1047) -> (x+1=w1046:i32)
                        n578 = Add(x=w1045, y=w1046) -> (x+y=w1048:i32)
                      }
                    }
                    n579 = To Unsigned Long Integer(number=w1039) -> (unsigned 32bit integer=w1040:u32)
                    n580 = Build Array(w1040) -> (w1043:u32[])
                    n581 = property on="Edited script" class="Arr (strict)"("Selection Start []"=w1043, "Selection Size []"=u32[] [1] ("Selection Size[]")) -> ()  [unwired: 2 in, 2 out]
                  }
                  event "Edited script": Mouse Down {
                    n582 = event-data() -> ("CtlRef"=w1051:refnum<vi>)  [unwired: 1 in, 7 out]
                    n583 = property class="Arr (strict)"(reference=w1051) -> (reference out=w1062:refnum<vi>, "Index Values"=w1058:u32[], "Array Element.Top"=w1056:i32, "Top"=w1055:i32, "Array Element.Height"=w1054:u32)  [unwired: 1 in, 1 out]
                    n584 = Subtract(x=w1056, y=w1055) -> (x-y=w1057:i32)
                    n585 = Index Array(array=w1058) -> (element=w1059:u32)  [unwired: 1 in]
                    n586 = Quotient & Remainder(x=w1057, y=w1054) -> (floor(x/y)=w1060:u32)  [unwired: 1 out]
                    n587 = Add(x=w1059, y=w1060) -> (x+y=w1053:u32)
                    n588 = Build Array(w1053) -> (w1061:u32[])
                    n589 = property class="Arr (strict)"(reference=w1062, "Selection Size []"=u32[] [1] ("Selection Size[]"), "Selection Start []"=w1061) -> ()  [unwired: 1 in, 2 out]
                    n590 = local write "Select\nline"(w1053) -> ()
                  }
                  event "Edited script": Value Change {
                    n591 = event-data() -> ("NewVal"=w1063:T27[])  [unwired: 1 in, 5 out]
                    n592 = Array Size(array=w1063) -> (size(s)=w1064:i32)
                    n593 = case shown="1, Default" w1064 {
                      selector: w1064 -> [w1067 w1069]
                      tunnel: [w1067 w1068] -> w1066
                      tunnel: [w1067 w1070] -> w1065
                      frame 0 {
                      }
                      frame 1, Default {
                        n594 = Decrement(x=w1069) -> (x-1=w1068:i32)
                        n595 = Negate(x=w1069) -> (-x=w1070:i32)
                      }
                    }
                    n596 = property on="Select\nline" class="DigNum (strict)"("Maximum"=w1066, "Minimum"=w1065) -> ()  [unwired: 2 in, 2 out]
                  }
                  event "Save script file btn": Value Change {
                    n597 = event-data() -> ()  [unwired: 1 in, 6 out]
                    n598 = local read "THz control"() -> (w1075:T22)
                    n599 = Unbundle By Name(w1075) -> ("AMC"=w1074:u16, "Multip"=w1073:u16)
                    n600 = Multiply(x=w1074, y=w1073) -> (x*y=w1072:u16)
                    n601 = call "Save script file.vi"("Multiplication factor"=w1072, "Script Array"="Edited script") -> ()  [unwired: 10 in]
                  }
                  event "Paste from meeasurrement": Value Change {
                    n602 = event-data() -> ()  [unwired: 1 in, 6 out]
                    n603 = local read "Script Array"() -> (w1076:T27[])
                    n604 = local write "Edited script"(w1076) -> ()
                  }
                }
              }
              frame "Measurement review" {
                n605 = event shown="[2] \"Open measurement\": Value Change" {
                  selector: _ -> [_ _ _ _]
                  dyn-events: _ -> [_ _ _ _]
                  timeout: 0 -> [_ _ _ _]
                  event Timeout {
                    n606 = event-data() -> ()  [unwired: 1 in, 3 out]
                  }
                  event "Data file to show": Value Change {
                    n607 = event-data() -> ("Type"=w1086:T78)  [unwired: 1 in, 3 out]
                    n608 = Format Into String(w1086) -> ()  [unwired: 3 in, 2 out]
                    n609 = local read "Results"() -> (w1085:T5)
                    n610 = Build Array("Data file to show") -> (w1087:u16[])
                    n611 = property on="Header" class="Arr (strict)"("Index Values"=w1087) -> ()  [unwired: 2 in, 2 out]
                    n612 = Index Array(array=w1085, index="Data file to show") -> (element=w1083:T56)
                    n613 = Unbundle(w1083) -> ("Mode"=w1081:T4, "Array"=w1082:cluster{"Array":dbl[], "Array":dbl[]}[])
                    n614 = case shown="\"MD EPR\", Default" w1081 {
                      frame "MD EPR", Default {
                        n615 = property on="Review Graph" class="XYGraph (strict)"("XScale.NameLbl.Text"="B [T]" ("X Scale.Name Label.Text")) -> ()  [unwired: 2 in, 2 out]
                      }
                      frame "FD EPR" {
                        n616 = property on="Review Graph" class="XYGraph (strict)"("XScale.NameLbl.Text"="F [GHz]" ("X Scale.Name Label.Text")) -> ()  [unwired: 2 in, 2 out]
                      }
                    }
                    n617 = local write "Review Graph"(w1082) -> ()
                  }
                  event "Open measurement": Value Change {
                    n618 = event-data() -> ()  [unwired: 1 in, 1 out]
                    n619 = local read "Main data folder"() -> (w1090:path)
                    n620 = call "Read data file.vi"("Application Directory"=w1090) -> ("Graph data"=w1092:cluster{"Array":dbl[], "Array":dbl[]}[], "Header"=w1094:string, "Mode"=w1093:T4, "Name"=w1095:string, "Error Out"=w1091:errorcluster)  [unwired: 6 in]
                    n621 = case shown="No Error" w1091 {
                      tunnel: w1095 -> [w1108 _]
                      tunnel: w1094 -> [w1103 _]
                      tunnel: w1093 -> [w1096 _]
                      tunnel: w1092 -> [w1098 _]
                      frame No Error {
                        n622 = local read "Data file to show"() -> (w1099:u16)
                        n623 = Bundle(cluster=T56 {"Mode"=enum."MD EPR", "Array"=[]} ("Cluster 2"), "Mode"=w1096, "Array"=w1098) -> (w1101:T56)
                        n624 = local read "Header"() -> (w1105:string[])
                        n625 = local read "Results"() -> (w1102:T5)
                        n626 = property on="Data file to show" class="Ring (strict)"() -> ("Strings []"=w1107:string[])  [unwired: 2 in, 2 out]
                        n627 = Replace Array Subset(array=w1107, new element=w1108, index=w1099) -> (w1106:string[])
                        n628 = Replace Array Subset(array=w1105, new element=w1103, index=w1099) -> (→"Header":string[])
                        n629 = Replace Array Subset(array=w1102, new element=w1101, index=w1099) -> (w1100:T5)
                        n630 = property on="Data file to show" class="Ring (strict)"("Strings []"=w1106) -> ()  [unwired: 2 in, 2 out]
                        n631 = local write "Results"(w1100) -> ()
                        "Review Graph" <- w1098
                      }
                      frame Error {
                      }
                    }
                  }
                  event "Shift data btn": Value Change {
                    n632 = event-data() -> ()  [unwired: 1 in, 2 out]
                    n633 = local read "Review Graph"() -> (w1117:cluster{"Array":dbl[], "Array":dbl[]}[])
                    n634 = Boolean To (0,1)(Boolean="Edit Channel") -> (0, 1=w1119:i16)
                    n635 = Index Array(array=w1117, index=w1119) -> (element=w1121:cluster{"Array":dbl[], "Array":dbl[]})
                    n636 = Unbundle(w1121) -> ("Array"=w1113:dbl[], "Array"=w1122:dbl[])
                    n637 = Array Max & Min(array=w1113) -> (max value=w1112:dbl, min value=w1111:dbl)  [unwired: 2 out]
                    n638 = Subtract(x=w1112, y=w1111) -> (x-y=w1110:dbl)
                    n639 = for {
                      tunnel: w1113 -> [w1135] mode=indexing
                      tunnel: "From point [T]" -> [w1136]
                      shift-right: [w1132] -> w1109
                      shift-left: -1 -> [w1131]
                      shift-right: [w1130] -> _
                      shift-left: w1110 -> [w1127]
                      i -> [w1133]
                      n640 = Subtract(x=w1135, y=w1136) -> (x-y=w1134:dbl)
                      n641 = Absolute Value(x=w1134) -> (abs(x)=w1128:dbl)
                      n642 = Less?(x=w1128, y=w1127) -> (x < y?=w1129:bool)
                      n643 = Select(t=w1128, s=w1129, f=w1127) -> (s? t:f=w1130:dbl)
                      n644 = Select(t=w1133, s=w1129, f=w1131) -> (s? t:f=w1132:i32)
                    }
                    n645 = Array Subset(array=w1122, index=w1109) -> (w1125:dbl[])  [unwired: 1 in]
                    n646 = Add(x=w1125, y="Amlitude shift [-]") -> (x+y=w1123:dbl[])
                    n647 = Replace Array Subset(array=w1122, new element=w1123, index=w1109) -> (w1120:dbl[])
                    n648 = Bundle(cluster=w1121, "Array"=w1113, "Array"=w1120) -> (w1118:cluster{"Array":dbl[], "Array":dbl[]})
                    n649 = Replace Array Subset(array=w1117, new element=w1118, index=w1119) -> (w1116:cluster{"Array":dbl[], "Array":dbl[]}[])
                    n650 = local write "Review Graph"(w1116) -> ()
                  }
                }
              }
            }
          }
          event "Tab Control": Value Change {
            n651 = event-data() -> ("NewVal"=w1138:T6)  [unwired: 1 in, 3 out]
            n652 = case shown="\"Adjustment\"" w1138 {
              frame "Page Status", Default {
              }
              frame "Adjustment" {
              }
            }
          }
          event "Disconnect": Value Change {
            n653 = event-data() -> ()  [unwired: 1 in, 6 out]
            n654 = local read "Select module"() -> (w1142:T7)
            n655 = Equal?(x=w1142, y=Module_selection."All") -> (x = y?=w1143:bool)
            n656 = case shown="True" w1143 {
              tunnel: w1141 -> [w1148 w1178]
              tunnel: w1142 -> [w1149 _]
              frame False {
                n657 = case shown="\"MAG\"" w1149 {
                  tunnel: w1148 -> [w1153 w1157 w1161 w1162 w1169 w1173 w1177 _]
                  frame "MAG" {
                    n658 = Unbundle By Name(w1153) -> ("Field_C"=w1151:refnum<queue>)
                    n659 = call "Put in mailbox.vi"("Priority? (F)"=TRUE ("Priority?"), "Message"=T38 {"Order"=enum."Disconnect", "Data"=variant} ("MSG to magnet"), "Queue in"=w1151) -> ()  [unwired: 6 in, 3 out]
                  }
                  frame "VTI" {
                    n660 = Unbundle By Name(w1157) -> ("Tmp_C"=w1155:refnum<queue>)
                    n661 = call "Put in mailbox.vi"("Priority? (F)"=TRUE ("Priority?"), "Message"=T52 {"Command"=enum."Disconnect", "Data"=variant} ("MSG for VTI"), "Queue in"=w1155) -> ()  [unwired: 6 in, 3 out]
                  }
                  frame "THz" {
                    n662 = Unbundle By Name(w1161) -> ("MW_C"=w1159:refnum<queue>)
                    n663 = call "Put in mailbox.vi"("Priority? (F)"=TRUE ("Priority?"), "Message"=T45 {"Command"=enum."Disconnect", "Data"=variant} ("Incoming msg"), "Queue in"=w1159) -> ()  [unwired: 6 in, 3 out]
                  }
                  frame "ACQ" {
                    n664 = Unbundle By Name(w1162) -> ("Data_Aq"=w1164:refnum<queue>)
                    n665 = call "Put in mailbox.vi"("Priority? (F)"=TRUE ("Priority?"), "Message"=T49 {"Command"=enum."Disconnect", "Data"=variant} ("MSG for  ACQ"), "Queue in"=w1164) -> ()  [unwired: 6 in, 3 out]
                  }
                  frame "SERV" {
                    n666 = Unbundle By Name(w1169) -> ("Table_C"=w1167:refnum<queue>)
                    n667 = call "Put in mailbox.vi"("Priority? (F)"=TRUE ("Priority?"), "Message"=T40 {"Command"=enum."Disconnect", "Data"=variant(dbl[] [])} ("MSG to Servo"), "Queue in"=w1167) -> ()  [unwired: 6 in, 3 out]
                  }
                  frame "ROT" {
                    n668 = Unbundle By Name(w1173) -> ("Angle_C"=w1171:refnum<queue>)
                    n669 = call "Put in mailbox.vi"("Priority? (F)"=TRUE ("Priority?"), "Message"=cluster{"Command":T42, "Data":variant} {"Command"=enum."Disconnect", "Data"=variant} ("MSG to rotator"), "Queue in"=w1171) -> ()  [unwired: 6 in, 3 out]
                  }
                  frame "SMU" {
                    n670 = Unbundle By Name(w1177) -> ("Mod_M"=w1175:refnum<queue>)
                    n671 = call "Put in mailbox.vi"("Priority? (F)"=TRUE ("Priority?"), "Message"=T53 {"Command"=enum."Disconnect", "Data"=variant} ("MSG to Source meter"), "Queue in"=w1175) -> ()  [unwired: 6 in, 3 out]
                  }
                  frame "None", Default {
                  }
                }
              }
              frame True {
                n672 = control-ref of="Instr status"() -> (w1179:refnum<vi>)
                n673 = property class="Clust (strict)"(reference=w1179) -> ("Controls[]"=w1180:refnum<vi>[])  [unwired: 1 in, 2 out]
                n674 = for {
                  tunnel: w1180 -> [w1186] mode=indexing
                  tunnel: w1178 -> [w1184]
                  n675 = property class="Ctl"(reference=w1186) -> ("Label.Text"=w1185:string, "Value"=w1183:variant)  [unwired: 1 in, 2 out]
                  n676 = Variant To Data(type=FALSE, Variant=w1183) -> (data=w1181:bool)  [unwired: 1 in, 1 out]
                  n677 = case shown="False" w1181 {
                    tunnel: w1185 -> [_ w1188]
                    tunnel: w1184 -> [_ w1187]
                    frame False {
                    }
                    frame True {
                      n678 = case shown="\"Ignore\", Default" w1188 {
                        tunnel: w1187 -> [w1192 w1196 w1200 w1204 w1208 w1212 w1216 _]
                        frame "Mag" {
                          n679 = Unbundle By Name(w1192) -> ("Field_C"=w1190:refnum<queue>)
                          n680 = call "Put in mailbox.vi"("Priority? (F)"=TRUE ("Priority?"), "Message"=T38 {"Order"=enum."Disconnect", "Data"=variant} ("MSG to magnet"), "Queue in"=w1190) -> ()  [unwired: 6 in, 3 out]
                        }
                        frame "SMU" {
                          n681 = Unbundle By Name(w1196) -> ("Mod_M"=w1194:refnum<queue>)
                          n682 = call "Put in mailbox.vi"("Priority? (F)"=TRUE ("Priority?"), "Message"=T53 {"Command"=enum."Disconnect", "Data"=variant} ("MSG to Source meter"), "Queue in"=w1194) -> ()  [unwired: 6 in, 3 out]
                        }
                        frame "VTI" {
                          n683 = Unbundle By Name(w1200) -> ("Tmp_C"=w1198:refnum<queue>)
                          n684 = call "Put in mailbox.vi"("Priority? (F)"=TRUE ("Priority?"), "Message"=T52 {"Command"=enum."End", "Data"=variant} ("MSG for VTI"), "Queue in"=w1198) -> ()  [unwired: 6 in, 3 out]
                        }
                        frame "THz" {
                          n685 = Unbundle By Name(w1204) -> ("MW_C"=w1202:refnum<queue>)
                          n686 = call "Put in mailbox.vi"("Priority? (F)"=TRUE ("Priority?"), "Message"=T45 {"Command"=enum."End", "Data"=variant} ("Incoming msg"), "Queue in"=w1202) -> ()  [unwired: 6 in, 3 out]
                        }
                        frame "ACQ" {
                          n687 = Unbundle By Name(w1208) -> ("Data_Aq"=w1206:refnum<queue>)
                          n688 = call "Put in mailbox.vi"("Priority? (F)"=TRUE ("Priority?"), "Message"=T49 {"Command"=enum."End", "Data"=variant} ("MSG for  ACQ"), "Queue in"=w1206) -> ()  [unwired: 6 in, 3 out]
                        }
                        frame "Serv" {
                          n689 = Unbundle By Name(w1212) -> ("Table_C"=w1210:refnum<queue>)
                          n690 = call "Put in mailbox.vi"("Priority? (F)"=TRUE ("Priority?"), "Message"=T40 {"Command"=enum."End", "Data"=variant(dbl[] [])} ("MSG to Servo"), "Queue in"=w1210) -> ()  [unwired: 6 in, 3 out]
                        }
                        frame "Rot" {
                          n691 = Unbundle By Name(w1216) -> ("Angle_C"=w1214:refnum<queue>)
                          n692 = call "Put in mailbox.vi"("Priority? (F)"=TRUE ("Priority?"), "Message"=cluster{"Command":T42, "Data":variant} {"Command"=enum."Disconnect", "Data"=variant} ("MSG to rotator"), "Queue in"=w1214) -> ()  [unwired: 6 in, 3 out]
                        }
                        frame "Ignore", Default {
                        }
                      }
                    }
                  }
                }
              }
            }
          }
          event "Stop": Value Change {
            n693 = event-data() -> ("NewVal"=w1222:bool)  [unwired: 1 in, 5 out]
            n694 = case shown="True" w1222 {
              tunnel: w1221 -> [_ w1226]
              tunnel: [_ w1225] -> w1220
              frame False {
              }
              frame True {
                # "Can not stop application just like that,\nAll modules must respond first, \nthat they are done."
                n695 = control-ref of="Instr status"() -> (w1228:refnum<vi>)
                n696 = property class="Clust (strict)"(reference=w1228) -> ("Value"=w1223:T79)  [unwired: 1 in, 2 out]
                n697 = property class="Clust (strict)"(reference=w1228) -> ("Controls[]"=w1229:refnum<vi>[])  [unwired: 1 in, 2 out]
                n698 = Cluster To Array(cluster=w1223) -> (array=w1227:bool[])
                n699 = Or Array Elements(Boolean array=w1227) -> (logical OR=w1224:bool)
                n700 = for {
                  tunnel: w1229 -> [w1235] mode=indexing
                  tunnel: w1226 -> [w1233]
                  n701 = property class="Ctl"(reference=w1235) -> ("Label.Text"=w1234:string, "Value"=w1232:variant)  [unwired: 1 in, 2 out]
                  n702 = Variant To Data(type=FALSE, Variant=w1232) -> (data=w1230:bool)  [unwired: 1 in, 1 out]
                  n703 = case shown="True" w1230 {
                    tunnel: w1234 -> [_ w1237]
                    tunnel: w1233 -> [_ w1236]
                    frame False {
                    }
                    frame True {
                      n704 = case shown="\"MFLI\"" w1237 {
                        tunnel: w1236 -> [w1241 w1245 w1249 w1253 w1257 w1261 w1265 _]
                        frame "Mag" {
                          n705 = Unbundle By Name(w1241) -> ("Field_C"=w1239:refnum<queue>)
                          n706 = call "Put in mailbox.vi"("Priority? (F)"=TRUE ("Priority?"), "Message"=T38 {"Order"=enum."Disconnect", "Data"=variant} ("MSG to magnet"), "Queue in"=w1239) -> ()  [unwired: 6 in, 3 out]
                        }
                        frame "VTI" {
                          n707 = Unbundle By Name(w1245) -> ("Tmp_C"=w1243:refnum<queue>)
                          n708 = call "Put in mailbox.vi"("Priority? (F)"=TRUE ("Priority?"), "Message"=T52 {"Command"=enum."End", "Data"=variant} ("MSG for VTI"), "Queue in"=w1243) -> ()  [unwired: 6 in, 3 out]
                        }
                        frame "THz" {
                          n709 = Unbundle By Name(w1249) -> ("MW_C"=w1247:refnum<queue>)
                          n710 = call "Put in mailbox.vi"("Priority? (F)"=TRUE ("Priority?"), "Message"=T45 {"Command"=enum."End", "Data"=variant} ("Incoming msg"), "Queue in"=w1247) -> ()  [unwired: 6 in, 3 out]
                        }
                        frame "MFLI" {
                          n711 = Unbundle By Name(w1253) -> ("Data_Aq"=w1251:refnum<queue>)
                          n712 = call "Put in mailbox.vi"("Priority? (F)"=TRUE ("Priority?"), "Message"=T49 {"Command"=enum."End", "Data"=variant} ("MSG for  ACQ"), "Queue in"=w1251) -> ()  [unwired: 6 in, 3 out]
                        }
                        frame "Serv" {
                          n713 = Unbundle By Name(w1257) -> ("Table_C"=w1255:refnum<queue>)
                          n714 = call "Put in mailbox.vi"("Priority? (F)"=TRUE ("Priority?"), "Message"=T40 {"Command"=enum."End", "Data"=variant(dbl[] [])} ("MSG to Servo"), "Queue in"=w1255) -> ()  [unwired: 6 in, 3 out]
                        }
                        frame "Rot" {
                          n715 = Unbundle By Name(w1261) -> ("Angle_C"=w1259:refnum<queue>)
                          n716 = call "Put in mailbox.vi"("Priority? (F)"=TRUE ("Priority?"), "Message"=cluster{"Command":T42, "Data":variant} {"Command"=enum."End", "Data"=variant} ("MSG to rotator"), "Queue in"=w1259) -> ()  [unwired: 6 in, 3 out]
                        }
                        frame "SMU" {
                          n717 = Unbundle By Name(w1265) -> ("Mod_M"=w1263:refnum<queue>)
                          n718 = call "Put in mailbox.vi"("Priority? (F)"=TRUE ("Priority?"), "Message"=T53 {"Command"=enum."End", "Data"=variant} ("MSG to Source meter"), "Queue in"=w1263) -> ()  [unwired: 6 in, 3 out]
                        }
                        frame "Ignore", Default {
                        }
                      }
                    }
                  }
                }
                n719 = case shown="False" w1224 {
                  tunnel: w1223 -> [_ _]
                  tunnel: w1226 -> [w1288 _]
                  tunnel: [TRUE _] -> w1225
                  frame False {
                    n720 = Cluster To Array(cluster=w1288) -> (array=w1289:refnum<queue>[])
                    n721 = local read "loggersRef"() -> (w1280:refnum<file>)
                    n722 = for {
                      tunnel: w1289 -> [w1297] mode=indexing
                      tunnel: [w1290] -> w1285
                      n723 = Wait (ms)(milliseconds to wait=u32 100) -> ()  [unwired: 1 out]
                      n724 = Get Queue Status(queue=w1297) -> (queue out=w1296:refnum<queue>, error out=w1291:errorcluster, # elements in queue=w1294:i32)  [unwired: 2 in, 5 out]
                      n725 = Less Or Equal?(x=w1294, y=0) -> (x <= y?=w1292:bool)
                      n726 = Release Queue(queue=w1296, force destroy? (F)=w1292, error in (no error)=w1291) -> (error out=w1290:errorcluster)  [unwired: 2 out]
                    }
                    n727 = Wait (ms)(milliseconds to wait=u32 2000) -> ()  [unwired: 1 out]
                    n728 = local read "Temperature log ref"() -> (w1284:refnum<file>)
                    n729 = call "Add actual date time to string.vi"("String in"="Program ended") -> ("String out"=w1281:string)  [unwired: 4 in]
                    n730 = call "Write in logger.vi"("String in"=w1281, "logger refnum"=w1280) -> ("refnum out"=w1279:refnum<file>)  [unwired: 2 in, 1 out]
                    n731 = local read "System config file path"() -> (w1278:path)
                    n732 = local read "Acquisition controls"() -> (w1275:T21)
                    n733 = local read "THz control"() -> (w1274:T22)
                    n734 = Close File(refnum=w1279, error in=w1285) -> (error out=w1283:errorcluster)  [unwired: 1 out]
                    n735 = Close File(refnum=w1284, error in=w1283) -> ()  [unwired: 2 out]
                    n736 = call "Open config file.vi"("MAG config file path"=w1278) -> ("error out"=w1276:errorcluster, "Refnum out"=w1277:T76)  [unwired: 7 in, 2 out]
                    n737 = Unbundle By Name(w1275) -> ("ACQ parameters"=w1271:T19)
                    n738 = call <userlib>:"Write Section Cluster__ogtk.vi"("error in (no error)"=w1276, "Section Formatted Cluster"=w1274, "refnum"=w1277) -> ("error out"=w1273:errorcluster, "dup refnum"=w1272:T76)  [unwired: 7 in]
                    n739 = local read "Instr info"() -> (w1266:T8)
                    n740 = call <userlib>:"Write Section Cluster__ogtk.vi"("error in (no error)"=w1273, "Section Formatted Cluster"=w1271, "refnum"=w1272) -> ("error out"=w1268:errorcluster, "dup refnum"=w1270:T76)  [unwired: 7 in]
                    n741 = call <userlib>:"Write Section Cluster__ogtk.vi"("error in (no error)"=w1268, "Section Formatted Cluster"=w1266, "refnum"=w1270) -> ("error out"=w1267:errorcluster, "dup refnum"=w1269:T76)  [unwired: 7 in]
                    n742 = call <vilib>:"Close Config Data.vi"("error in (no error)"=w1267, "refnum"=w1269) -> ()  [unwired: 8 in, 2 out]
                  }
                  frame True {
                  }
                }
              }
            }
          }
          event "Re-connect instruments": Value Change {
            n743 = event-data() -> ()  [unwired: 1 in, 4 out]
            n744 = local read "System config file path"() -> (w1299:path)
            n745 = case shown="\"THz\"" "Select module" {
              tunnel: w1304 -> [w1309 _ w1319 w1350 w1360 w1368 w1375 w1396 w1406]
              tunnel: w1299 -> [w1308 _ _ _ _ _ _ w1390 w1398]
              tunnel: w1303 -> [w1307 w1310 w1320 w1351 w1357 w1366 w1376 w1397 w1407]
              tunnel: [w1307 w1310 w1320 w1351 w1357 w1366 w1376 w1397 w1407] -> w1302
              tunnel: "Use previous settings" -> [_ _ w1311 _ _ _ _ _ _]
              frame "All", Default {
                n746 = call "Send message to initialize all modules.vi"("System config file path"=w1308, "Messenger referencies"=w1309) -> ()  [unwired: 10 in]
                n747 = property on="Select module" class="Enum (strict)"("DisabledEnum"=T34."Enabled" ("Disabled")) -> ()  [unwired: 2 in, 2 out]
              }
              frame "None" {
              }
              frame "ACQ" {
                w1312 = T49 {"Command"=enum."Initialize", "Data"=variant} ("MSG for  ACQ")
                n748 = Unbundle By Name(w1319) -> ("Data_Aq"=w1316:refnum<queue>)
                n749 = Bundle By Name(cluster=w1312, "Command"=MFLI_command_enum."Initialize", "Data"="MF-DEV4029") -> (w1317:T49)
                n750 = call "Put in mailbox.vi"("Priority? (F)"=TRUE, "Message"=w1317, "Queue in"=w1316) -> ("Queue out"=w1313:refnum<queue>)  [unwired: 6 in, 2 out]
                n751 = case shown="True" w1311 {
                  tunnel: w1313 -> [_ w1342]
                  tunnel: w1312 -> [_ w1340]
                  frame False {
                  }
                  frame True {
                    w1329 = T46 {"parameter"=enum."filter_order [-]", "value"=0.0} ("Parameter to set")
                    n752 = local read "Acquisition controls"() -> (w1338:T21)
                    n753 = Unbundle By Name(w1338) -> ("ACQ parameters"=w1325:T19)
                    n754 = Unbundle By Name(w1325) -> ("Filter order"=w1337:dbl, "Filter tau [ms]"=w1336:dbl, "F_Mod [kHz]"=w1335:dbl, "Amp_Mod [mV]"=w1334:dbl)
                    n755 = Divide(x=w1334, y=1000.0) -> (x/y=w1333:dbl)
                    n756 = Bundle(cluster=w1329, "parameter"=MFLI_node."osc_freq [kHz]", "value"=w1335) -> (w1327:T46)
                    n757 = Bundle(cluster=w1329, "parameter"=MFLI_node."filter_constant [ms]", "value"=w1336) -> (w1328:T46)
                    n758 = Bundle(cluster=w1329, "parameter"=MFLI_node."out_ampl [V]", "value"=w1333) -> (w1331:T46)
                    n759 = Bundle(cluster=w1329, "parameter"=MFLI_node."filter_order [-]", "value"=w1337) -> (w1330:T46)
                    n760 = Build Array(w1330, w1328, w1327, w1331) -> (w1326:T46[])
                    n761 = Bundle By Name(cluster=w1340, "Command"=MFLI_command_enum."Set individual parameters", "Data"=w1326) -> (w1341:T49)
                    n762 = call "Put in mailbox.vi"("Message"=w1341, "Queue in"=w1342) -> ()  [unwired: 7 in, 3 out]
                  }
                }
              }
              frame "ROT" {
                n763 = Unbundle By Name(w1350) -> ("Angle_C"=w1347:refnum<queue>)
                n764 = disable-structure shown="TARGET_BITNESS==64, Default" {
                  disable-tunnel: [path "C:/Program Files/National Instruments/LabVIEW 2024/instr.lib/ANC350/Win32/anc350v4.dll" ("File Path Control") path "C:/Programs/Debug/ANC350 lib/Software_ANC350v4/Windows/ANC350_Library/lib64/anc350v4.dll" ("File Path Control")] -> w1343
                  frame condition #0 {
                  }
                  frame condition #1 (active) {
                  }
                }
                n765 = Build Array(w1343, path "C:/Programs/Debug/HFEPR spectrometer SW 2024/Multi-HFEPR app/SystemData/ANRv51-C4-124.LUT" ("File Path Control")) -> (w1345:path[])
                n766 = Bundle By Name(cluster=T41 {"Command"=enum."Initialize", "Data"=variant} ("MSG to rotator"), "Command"=Rotator_commands."Initialize", "Data"=w1345) -> (w1349:T41)
                n767 = disable-structure shown="Enabled" {
                  disable-tunnel: w1349 -> [w1355 _]
                  disable-tunnel: w1347 -> [w1354 _]
                  frame Enabled {
                    n768 = call "Put in mailbox.vi"("Message"=w1355, "Queue in"=w1354) -> ()  [unwired: 7 in, 3 out]
                  }
                  frame Disabled {
                  }
                }
              }
              frame "VTI" {
                n769 = Unbundle By Name(w1360) -> ("Tmp_C"=w1359:refnum<queue>)
                n770 = Bundle By Name(cluster=T52 {"Command"=enum."Initialize", "Data"=variant} ("MSG for VTI"), "Command"=TC_commands."Initialize", "Data"="COM4") -> (w1358:T52)
                n771 = call "Put in mailbox.vi"("Message"=w1358, "Queue in"=w1359) -> ()  [unwired: 7 in, 3 out]
              }
              frame "SMU" {
                n772 = Unbundle By Name(w1368) -> ("Field_M"=w1367:refnum<queue>)
                n773 = Bundle By Name(cluster=T53 {"Command"=enum."Connect", "Data"=variant} ("MSG to Source meter"), "Data"="USB0::0x05E6::0x2450::04405250::INSTR") -> (w1364:T53)
                n774 = call "Put in mailbox.vi"("Message"=w1364, "Queue in"=w1367) -> ()  [unwired: 7 in, 3 out]
              }
              frame "THz" {
                n775 = disable-structure shown="Enabled" {
                  disable-tunnel: [T57[] [{"Lower limit [GHz]"=8.0, "Upper limit [GHz]"=20.0, "Device name"="VDIS0122", "Connection"="", "Description"="VDI Synth", "Connected"=FALSE, "Last settings"="", "Operation mode"=enum."Disabled", "Enable ch 1"=FALSE, "Enable ch 2"=FALSE}, {"Lower limit [GHz]"=8.0, "Upper limit [GHz]"=20.0, "Device name"="VDIYT7", "Connection"="", "Description"="VDI Tracking", "Connected"=FALSE, "Last settings"="", "Operation mode"=enum."Disabled", "Enable ch 1"=FALSE, "Enable ch 2"=FALSE}] ("Array") w1378] -> w1369
                  frame Disabled {
                  }
                  frame Enabled {
                    n776 = Bundle By Name(cluster=T57 {"Lower limit [GHz]"=0.0, "Upper limit [GHz]"=0.0, "Device name"="", "Connection"="", "Description"="", "Connected"=FALSE, "Last settings"="", "Operation mode"=enum."Disabled", "Enable ch 1"=FALSE, "Enable ch 2"=FALSE} ("Configuration"), "Connection"="USB0::0x03EB::0xAFFF::848-0B4424003-0065::INSTR") -> (w1379:T57)
                    n777 = Build Array(w1379) -> (w1378:T57[])
                  }
                }
                n778 = Unbundle By Name(w1375) -> ("MW_C"=w1371:refnum<queue>)
                n779 = Bundle By Name(cluster=T45 {"Command"=enum."Connect", "Data"=variant} ("Incoming msg"), "Command"=THz_commands_enum."Connect", "Data"=w1369) -> (w1374:T45)
                n780 = call "Put in mailbox.vi"("Priority? (F)"=TRUE, "Message"=w1374, "Queue in"=w1371) -> ()  [unwired: 6 in, 3 out]
              }
              frame "MAG" {
                n781 = call "Read magnet system configuration.vi"("MAG config file path"=w1390) -> ("error out"=w1392:errorcluster, "Magnet Constantsout"=w1388:T80)  [unwired: 8 in, 1 out]
                n782 = Unbundle By Name(w1396) -> ("Field_C"=w1391:refnum<queue>)
                n783 = Unbundle By Name(w1388) -> ("Maximum field [T]"=w1387:dbl, "Field Constant [T/A]"=w1385:dbl, "Ramp limits [A/s]"=w1386:dbl[])
                n784 = Bundle By Name(cluster=T38 {"Order"=enum."Connect", "Data"=variant(enum16{"Ramping", "Perzistant"} enum."Ramping")} ("MSG to magnet"), "Order"=Magnet_Orders."Connect", "Data"=w1388) -> (w1394:T38)
                n785 = Index Array(array=w1386) -> (element=w1384:dbl)  [unwired: 1 in]
                n786 = call "Put in mailbox.vi"("Priority? (F)"=TRUE, "error in (no error)"=w1392, "Message"=w1394, "Queue in"=w1391) -> ()  [unwired: 5 in, 3 out]
                n787 = Compound Arithmetic op=MULTIPLY(w1385, w1384, 1000.0 ("value")) -> (w1382:dbl)
                n788 = property on="Set Field [T]" class="DigNum (strict)"("Maximum"=w1387) -> ()  [unwired: 2 in, 2 out]
                n789 = property on="Desired\nramp [mT/s]" class="DigNum (strict)"("Maximum"=w1382) -> ()  [unwired: 2 in, 2 out]
              }
              frame "SERV" {
                n790 = Unbundle By Name(w1406) -> ("Table_C"=w1399:refnum<queue>)
                n791 = call "Servo Read system configuration.vi"("MAG config file path"=w1398) -> ("error out"=w1403:errorcluster, "IP addresses"=w1404:string[])  [unwired: 8 in, 1 out]
                n792 = Bundle By Name(cluster=T40 {"Command"=enum."Initialize", "Data"=variant(dbl[] [])} ("MSG to Servo"), "Command"=Servo_commands."Initialize", "Data"=w1404) -> (w1405:T40)
                n793 = call "Put in mailbox.vi"("Priority? (F)"=TRUE, "error in (no error)"=w1403, "Message"=w1405, "Queue in"=w1399) -> ()  [unwired: 5 in, 3 out]
              }
            }
          }
        }
        "Actual measurement" <- w114
        "Logger" <- w113
        n794 = Index Array(array=w113) -> (element=w118:string)  [unwired: 1 in]
        n795 = Bundle By Name(cluster=w117, "Last log"=w118) -> (w115:T25)
        n796 = local write "Infobar"(w115) -> ()
      }
      frame "Check message" {
        n797 = Unbundle By Name(w1412) -> ("TOP"=w1429:refnum<queue>)
        n798 = call "Receive message by TOP.vi"("timeout (100)"=10 ("timeout in ms (-1)"), "Mailbox in"=w1429) -> ("error out"=w1422:errorcluster, "timed out?"=w1424:bool, "Unread"=w1421:i32, "MSG packet"=w1428:T81)  [unwired: 6 in]
        n799 = Or(x=w1424, y=w1422) -> (x .or. y?=w1423:bool)
        n800 = local read "Busy"() -> (w1418:bool)
        n801 = Unbundle By Name(w1409) -> ("Experiment state"=w1408:T26)
        n802 = Not(x=w1418) -> (.not. x?=w1416:bool)
        n803 = Greater?(x=w1421, y=2) -> (0:w1419:bool)
        n804 = And(x=w1419, y=w1416) -> (x .and. y?=w1417:bool)
        n805 = case shown="False" w1423 {
          tunnel: w1428 -> [w1451 _]
          tunnel: w1426 -> [w1448 w2834]
          tunnel: [w1447 w2834] -> w1425
          tunnel: w1409 -> [w1442 w2833]
          tunnel: [w1441 w2833] -> w1414
          tunnel: w1413 -> [w1444 _]
          tunnel: w1412 -> [w1443 _]
          tunnel: w1411 -> [w1440 w2832]
          tunnel: [w1439 w2832] -> w1410
          frame False {
            n806 = Unbundle By Name(w1451) -> ("Time"=w1446:timestamp, "Module"=w1450:T82, "Response"=w1449:string, "Data"=w1445:variant)
            n807 = case "Message from module:" shown="\"Excitation\"" w1450 {
              selector: w1450 -> [_ _ _ _ _ _ _ _ _ _ w2663 w2828]
              tunnel: w1449 -> [w1462 w1778 w1914 w1929 w1944 w1962 w1985 w2119 w2261 w2388 w2667 w2826]
              tunnel: w1445 -> [w1461 w1775 w1911 w1926 w1941 w1959 w1982 w2118 w2260 w2391 w2666 _]
              tunnel: w1448 -> [w1460 w1777 w1913 w1928 w1943 w1961 w1984 w2115 w2259 w2390 w2665 w2831]
              tunnel: [w1459 w1776 w1912 w1927 w1942 w1960 w1983 w2114 w2258 w2389 w2664 w2830] -> w1447
              tunnel: w1446 -> [w1458 w1774 w1910 w1925 w1940 w1958 w1981 w2117 w2253 w2382 w2656 _]
              tunnel: w1442 -> [w1457 w1772 w1908 w1923 w1938 w1956 w1979 w2116 w2251 w2387 w2662 w2824]
              tunnel: [w1456 w1773 w1909 w1924 w1939 w1957 w1980 w2116 w2257 w2387 w2662 w2824] -> w1441
              tunnel: w1444 -> [_ _ w1907 w1922 w1937 w1955 w1978 _ _ _ _ _]
              tunnel: w1443 -> [_ _ _ _ _ _ _ w2109 _ _ _ _]
              tunnel: w1440 -> [w1455 w1771 w1906 w1921 w1936 w1954 w1977 w2110 w2256 w2386 w2660 w2823]
              tunnel: [w1453 w1769 w1904 w1919 w1934 w1952 w1975 w2111 w2255 w2385 w2658 w2823] -> w1439
              frame "Magnet" {
                # "list of responses:"
                n808 = Unbundle By Name(w1455) -> ("Magnet"=w1454:T83)
                n809 = case shown="\"Temperatures\"" w1462 {
                  selector: w1462 -> [w1469 _ _ _ _ _ _ _ _ _ _ w1666 _ _ _ _]
                  tunnel: w1461 -> [w1465 w1512 w1526 w1537 w1561 w1590 w1600 w1615 w1628 w1638 w1653 w1670 w1703 w1741 _ _]
                  tunnel: w1460 -> [w1467 w1509 w1519 w1533 w1545 w1582 w1595 w1613 w1626 w1635 w1650 w1663 w1686 w1742 w1746 w1758]
                  tunnel: [w1468 w1492 w1520 w1532 w1544 w1581 w1596 w1614 w1627 w1636 w1651 w1662 w1687 w1742 w1745 w1757] -> w1459
                  tunnel: w1458 -> [_ _ _ _ w1548 _ _ _ _ _ _ _ w1678 w1737 _ _]
                  tunnel: w1457 -> [w1464 w1497 w1518 w1529 w1551 w1578 w1594 w1612 w1625 w1634 w1649 w1661 w1672 w1738 w1748 w1760]
                  tunnel: [w1464 w1497 w1518 w1529 w1550 w1578 w1594 w1612 w1625 w1634 w1649 w1661 w1684 w1738 w1748 w1760] -> w1456
                  tunnel: w1454 -> [w1463 w1496 w1517 w1527 w1549 w1577 w1593 w1611 w1624 w1633 w1648 w1660 w1682 w1727 w1744 w1756]
                  tunnel: [w1463 w1491 w1516 w1527 w1547 w1577 w1593 w1611 w1624 w1633 w1648 w1659 w1677 w1727 w1744 w1756] -> w1452
                  frame "ignore", Default {
                    n810 = Match Pattern(string=w1469, regular expression="Error") -> (after substring=w1466:string, offset past match=w1471:i32)  [unwired: 1 in, 2 out]
                    n811 = Greater Or Equal To 0?(x=w1471) -> (x >= 0?=w1470:bool)
                    n812 = case shown="True" w1470 {
                      tunnel: w1467 -> [w1475 w1485]
                      tunnel: w1469 -> [w1474 w1484]
                      tunnel: [w1473 w1486] -> w1468
                      tunnel: w1466 -> [_ _]
                      tunnel: w1465 -> [_ w1482]
                      frame False {
                        n813 = call "simple Shift string array.vi"("Element in"=w1474, "Array in"=w1475) -> ("Array out"=w1473:string[])  [unwired: 8 in, 1 out]
                      }
                      frame True {
                        n814 = Variant To Data(type=errorcluster {"status"=FALSE, "code"=0, "source"=""} ("error constant"), Variant=w1482) -> (data=w1480:errorcluster)  [unwired: 1 in, 1 out]
                        n815 = Unbundle By Name(w1480) -> ("source"=w1479:string)
                        n816 = call <vilib>:"Space Constant.vi"() -> ("String"=w1483:string)
                        n817 = Concatenate Strings("Magnet: " ("string"), w1484, w1483, w1479) -> (w1477:string)
                        n818 = local read "loggersRef"() -> (w1478:refnum<file>)
                        n819 = call "Write in logger.vi"("String in"=w1477, "logger refnum"=w1478) -> ()  [unwired: 2 in, 2 out]
                        n820 = call "simple Shift string array.vi"("Element in"=w1477, "Array in"=w1485) -> ("Array out"=w1486:string[])  [unwired: 8 in, 1 out]
                      }
                    }
                  }
                  frame "Connect" {
                    w1504 = TRUE ("PSU")
                    w1503 = T34."Enabled" ("Disabled")
                    n821 = Variant To Data(type="", Variant=w1512) -> (data=w1488:string)  [unwired: 1 in, 1 out]
                    n822 = local read "Instr status"() -> (w1507:T1)
                    n823 = Bundle By Name(cluster=w1507, "Mag"=w1504) -> (w1511:T1)
                    n824 = Unbundle By Name(w1507) -> ("THz"=w1506:bool, "MFLI"=w1505:bool)
                    n825 = local write "Instr status"(w1511) -> ()
                    n826 = control-ref of="Magnet controls"() -> (w1508:refnum<vi>)
                    n827 = Compound Arithmetic op=AND(w1506, w1505, w1504) -> (w1502:bool)
                    n828 = call "Add actual date time to string.vi"("String in"="Magnet module initialized") -> ("String out"=w1500:string)  [unwired: 4 in]
                    n829 = Select(t=w1503, s=w1502, f=T34."Disabled and Grayed Out" ("Disabled")) -> (s? t:f=w1498:T34)
                    n830 = local read "loggersRef"() -> (w1499:refnum<file>)
                    n831 = property class="Clust (strict)"(reference=w1508, "DisabledEnum"=w1503) -> ()  [unwired: 1 in, 2 out]
                    n832 = Concatenate Strings(w1500, "\r\n", w1488) -> (w1490:string)
                    n833 = call "simple Shift string array.vi"("Element in"=w1500, "Array in"=w1509) -> ("Array out"=w1493:string[])  [unwired: 8 in, 1 out]
                    n834 = call "Write in logger.vi"("String in"=w1490, "logger refnum"=w1499) -> ()  [unwired: 2 in, 2 out]
                    n835 = call "Add actual date time to string.vi"("String in"=w1488) -> ("String out"=w1494:string)  [unwired: 4 in]
                    n836 = call "simple Shift string array.vi"("Element in"=w1494, "Array in"=w1493) -> ("Array out"=w1492:string[])  [unwired: 8 in, 1 out]
                    n837 = property on="Run script btn" class="Bool (strict)"("DisabledEnum"=w1498) -> ()  [unwired: 2 in, 2 out]
                    n838 = Bundle By Name(cluster=w1496, "PSU"="SMS120" ("regular expression")) -> (w1491:T83)
                  }
                  frame "TM revision" {
                    n839 = Variant To Data(type=T58 {"Instr Serial Number"="", "Instr Driver Revision"="", "Instr Firmware Revision"="", "Instr Model Number"=""} ("TM Revision"), Variant=w1526) -> (data=w1524:T58)  [unwired: 1 in, 1 out]
                    n840 = Unbundle By Name(w1524) -> ("Instr Model Number"=w1515:string)
                    n841 = call <vilib>:"Space Constant.vi"() -> ("String"=w1522:string)
                    n842 = Concatenate Strings("Temperature monitor:" ("string"), w1522, w1515) -> (w1521:string)
                    n843 = Bundle By Name(cluster=w1517, "T monitor"=w1515) -> (w1516:T83)
                    n844 = call "Add actual date time to string.vi"("String in"=w1521) -> ("String out"=w1513:string)  [unwired: 4 in]
                    n845 = local read "loggersRef"() -> (w1514:refnum<file>)
                    n846 = call "simple Shift string array.vi"("Element in"=w1513, "Array in"=w1519) -> ("Array out"=w1520:string[])  [unwired: 8 in, 1 out]
                    n847 = call "Write in logger.vi"("String in"=w1513, "logger refnum"=w1514) -> ()  [unwired: 2 in, 2 out]
                  }
                  frame "Initialization error" {
                    n848 = Variant To Data(type=errorcluster {"status"=FALSE, "code"=0, "source"=""} ("error constant"), Variant=w1537) -> (data=w1535:errorcluster, error out=w1528:errorcluster)  [unwired: 1 in]
                    n849 = Unbundle By Name(w1535) -> ("source"=w1534:string)
                    n850 = call "Add actual date time to string.vi"("String in"=w1534) -> ("String out"=w1531:string)  [unwired: 4 in]
                    n851 = call "simple Shift string array.vi"("Element in"=w1531, "Array in"=w1533) -> ("Array out"=w1532:string[])  [unwired: 8 in, 1 out]
                    n852 = local read "loggersRef"() -> (w1530:refnum<file>)
                    n853 = call "Write in logger.vi"("error in"=w1528, "String in"=w1531, "logger refnum"=w1530) -> ()  [unwired: 1 in, 2 out]
                  }
                  frame "Update" {
                    n854 = Variant To Data(type=T59 {"Desired"={"Field [T]"=0.0, "Ramp [T/s]"=0.0, "Custom Ramp?"=TRUE, "Mode"=enum."Persistant"}, "Actual"={"Mode"=enum."Persistant", "Ramping output"=enum."At Target", "Ready for change"=FALSE, "Switch heater"=FALSE, "Cooler Overheat"=FALSE, "Coil overheat"=FALSE, "Energized"=FALSE, "Output [T]"=0.0, "Field [T]"=0.0, "Ramp[T/s]"=0.0, "Switch\ntemperature [K]"=1.0, "Voltage [V]"=0.0, "Current direction"=FALSE}} ("output cluster"), Variant=w1561) -> (data=w1543:T59)  [unwired: 1 in, 1 out]
                    n855 = Unbundle By Name(w1543) -> ("Actual.Ready for change"=w1541:bool, "Actual.Mode"=w1542:T61, "Actual.Field [T]"=w1539:dbl)
                    n856 = local read "Instr status"() -> (w1559:T1)
                    n857 = local read "Magnet controls"() -> (w1554:T24)
                    n858 = Bundle By Name(cluster=w1559, "Mag"=TRUE ("PSU")) -> (w1558:T1)
                    n859 = Bundle By Name(cluster=w1551, "Field [T]"=w1539) -> (w1550:T25)
                    n860 = local write "Instr status"(w1558) -> ()
                    n861 = call "Magnet update rewiring.vi"("output cluster"=w1543, "Time"=w1548, "Magnet in"=w1549, "Magnet controls in"=w1554) -> ("Magnet out"=w1547:T83, "Magnet controls out"=w1553:T24)  [unwired: 6 in]
                    n862 = Greater?(x=w1539, y=0.01) -> (0:→"Magnetic\nfield state":bool)
                    n863 = local write "Magnet controls"(w1553) -> ()
                    n864 = case shown="\"Quenched\"" w1542 {
                      selector: w1542 -> [_ _ _ w1570]
                      tunnel: [w1563 w1564 w1567 w1572] -> w1544
                      tunnel: w1545 -> [w1563 w1564 w1567 w1571]
                      tunnel: [T34."Enabled" ("Disabled") T34."Disabled and Grayed Out" ("f") T34."Disabled and Grayed Out" ("f") T34."Disabled and Grayed Out" ("f")] -> w1546
                      frame "Persistant", Default {
                      }
                      frame "Switching" {
                      }
                      frame "Ramping" {
                      }
                      frame "Quenched" {
                        n865 = Format Into String(w1570) -> (resulting string=w1569:string)  [unwired: 3 in, 1 out]
                        n866 = call "Add actual date time to string.vi"("String in"=w1569) -> ("String out"=w1573:string)  [unwired: 4 in]
                        n867 = local read "loggersRef"() -> (w1574:refnum<file>)
                        n868 = call "simple Shift string array.vi"("Element in"=w1573, "Array in"=w1571) -> ("Array out"=w1572:string[])  [unwired: 8 in, 1 out]
                        n869 = call "Write in logger.vi"("String in"=w1573, "logger refnum"=w1574) -> ()  [unwired: 2 in, 2 out]
                      }
                    }
                    n870 = Select(t=T34."Enabled" ("Disabled"), s=w1541, f=T34."Disabled and Grayed Out") -> (s? t:f=w1552:T34)
                    n871 = property on="Mode switch" class="Bool (strict)"("DisabledEnum"=w1552) -> ()  [unwired: 2 in, 2 out]
                    n872 = property on="Equalize" class="Bool (strict)"("DisabledEnum"=w1546) -> ()  [unwired: 2 in, 2 out]
                    n873 = property on="Discharge" class="Bool (strict)"("DisabledEnum"=w1546) -> ()  [unwired: 2 in, 2 out]
                  }
                  frame "Update error" {
                    # "ReInitialize Magnet?"
                    n874 = Variant To Data(type=errorcluster {"status"=FALSE, "code"=0, "source"=""} ("error in (no error)"), Variant=w1590) -> (data=w1588:errorcluster)  [unwired: 1 in, 1 out]
                    n875 = Unbundle By Name(w1588) -> ("source"=w1585:string)
                    n876 = local read "Instr status"() -> (w1584:T1)
                    n877 = Bundle By Name(cluster=w1584, "Mag"=FALSE ("PSU")) -> (w1583:T1)
                    n878 = local write "Instr status"(w1583) -> ()
                    n879 = Concatenate Strings("Magnet Update error: " ("String in"), w1585) -> (w1586:string)
                    n880 = property on="Magnet controls" class="Clust (strict)"("DisabledEnum"=T34."Disabled and Grayed Out" ("Disabled")) -> ()  [unwired: 2 in, 2 out]
                    n881 = local read "loggersRef"() -> (w1576:refnum<file>)
                    n882 = call "Add actual date time to string.vi"("String in"=w1586) -> ("String out"=w1575:string)  [unwired: 4 in]
                    n883 = call "Write in logger.vi"("String in"=w1575, "logger refnum"=w1576) -> ()  [unwired: 2 in, 2 out]
                    n884 = call "simple Shift string array.vi"("Element in"=w1575, "Array in"=w1582) -> ("Array out"=w1581:string[])  [unwired: 8 in, 1 out]
                  }
                  frame "Switch mode acepted" {
                    n885 = Variant To Data(type=Magnet_mode_public."Ramping" ("Operation mode"), Variant=w1600) -> (data=w1598:T35)  [unwired: 1 in, 1 out]
                    n886 = case shown="\"Ramping\", Default" w1598 {
                      tunnel: ["Switching to ramping mode" "Switching to perzistant mode"] -> w1597
                      frame "Ramping", Default {
                      }
                      frame "Persistant" {
                      }
                    }
                    n887 = call "Add actual date time to string.vi"("String in"=w1597) -> ("String out"=w1591:string)  [unwired: 4 in]
                    n888 = local read "loggersRef"() -> (w1592:refnum<file>)
                    n889 = call "simple Shift string array.vi"("Element in"=w1591, "Array in"=w1595) -> ("Array out"=w1596:string[])  [unwired: 8 in, 1 out]
                    n890 = call "Write in logger.vi"("String in"=w1591, "logger refnum"=w1592) -> ()  [unwired: 2 in, 2 out]
                  }
                  frame "Equalize output" {
                    n891 = Variant To Data(type=T36 {"Field [T]"=0.0, "Ramp [T/s]"=0.0, "Custom Ramp?"=TRUE, "Mode"=enum."Persistant"} ("Desired"), Variant=w1615) -> (data=w1607:T36)  [unwired: 1 in, 1 out]
                    n892 = Unbundle By Name(w1607) -> ("Field [T]"=w1603:dbl, "Ramp [T/s]"=w1606:dbl)
                    n893 = Equal To 0?(x=w1606) -> (x = 0?=w1605:bool)
                    n894 = case shown="False" w1605 {
                      tunnel: [w1616 "Output equalization command ignored"] -> w1604
                      tunnel: w1603 -> [w1618 _]
                      frame False {
                        n895 = Format Into String(format string="Output equalized to %f T ", w1618) -> (resulting string=w1616:string)  [unwired: 2 in, 1 out]
                      }
                      frame True {
                      }
                    }
                    n896 = call "Add actual date time to string.vi"("String in"=w1604) -> ("String out"=w1609:string)  [unwired: 4 in]
                    n897 = local read "loggersRef"() -> (w1610:refnum<file>)
                    n898 = call "simple Shift string array.vi"("Element in"=w1609, "Array in"=w1613) -> ("Array out"=w1614:string[])  [unwired: 8 in, 1 out]
                    n899 = call "Write in logger.vi"("String in"=w1609, "logger refnum"=w1610) -> ()  [unwired: 2 in, 2 out]
                  }
                  frame "Stop ramping" {
                    n900 = Variant To Data(type="" ("Desired"), Variant=w1628) -> (data=w1620:string)  [unwired: 1 in, 1 out]
                    n901 = call "Add actual date time to string.vi"("String in"=w1620) -> ("String out"=w1622:string)  [unwired: 4 in]
                    n902 = local read "loggersRef"() -> (w1623:refnum<file>)
                    n903 = call "simple Shift string array.vi"("Element in"=w1622, "Array in"=w1626) -> ("Array out"=w1627:string[])  [unwired: 8 in, 1 out]
                    n904 = call "Write in logger.vi"("String in"=w1622, "logger refnum"=w1623) -> ()  [unwired: 2 in, 2 out]
                  }
                  frame "Flip polarity" {
                    n905 = Variant To Data(type="" ("Operation mode"), Variant=w1638) -> (data=w1630:string, error out=w1629:errorcluster)  [unwired: 1 in]
                    n906 = call "Add actual date time to string.vi"("String in"=w1630) -> ("String out"=w1631:string)  [unwired: 4 in]
                    n907 = local read "loggersRef"() -> (w1632:refnum<file>)
                    n908 = call "simple Shift string array.vi"("Element in"=w1631, "Array in"=w1635) -> ("Array out"=w1636:string[])  [unwired: 8 in, 1 out]
                    n909 = call "Write in logger.vi"("error in"=w1629, "String in"=w1631, "logger refnum"=w1632) -> ()  [unwired: 1 in, 2 out]
                  }
                  frame "Zero output" {
                    n910 = Variant To Data(type=TRUE, Variant=w1653) -> (data=w1644:bool, error out=w1645:errorcluster)  [unwired: 1 in]
                    n911 = Select(t="confirmed", s=w1644, f="denied") -> (s? t:f=w1641:string)
                    n912 = Concatenate Strings("Zero output ", w1641) -> (w1639:string)
                    n913 = call "Add actual date time to string.vi"("String in"=w1639) -> ("String out"=w1646:string)  [unwired: 4 in]
                    n914 = local read "loggersRef"() -> (w1647:refnum<file>)
                    n915 = call "simple Shift string array.vi"("Element in"=w1646, "Array in"=w1650) -> ("Array out"=w1651:string[])  [unwired: 8 in, 1 out]
                    n916 = call "Write in logger.vi"("error in"=w1645, "String in"=w1646, "logger refnum"=w1647) -> ()  [unwired: 1 in, 2 out]
                  }
                  frame "Ramping" {
                    n917 = Variant To Data(type=T36 {"Field [T]"=0.0, "Ramp [T/s]"=0.0, "Custom Ramp?"=TRUE, "Mode"=enum."Persistant"} ("Set Field"), Variant=w1670) -> (data=w1668:T36)  [unwired: 1 in, 1 out]
                    n918 = Unbundle By Name(w1668) -> ("Field [T]"=w1665:dbl, "Ramp [T/s]"=w1657:dbl)
                    n919 = Multiply(x=w1657, y=1000.0) -> (x*y=w1656:dbl)
                    n920 = Bundle By Name(cluster=w1660, "Ramp [mT/s]"=w1656) -> (w1659:T83)
                    n921 = Format Into String(format string=" B= %f [T] Ramp= %f [mT/s]", initial string=w1666, w1665, w1656) -> (resulting string=w1664:string)  [unwired: 1 in, 1 out]
                    n922 = call "Add actual date time to string.vi"("String in"=w1664) -> ("String out"=w1654:string)  [unwired: 4 in]
                    n923 = local read "loggersRef"() -> (w1655:refnum<file>)
                    n924 = call "simple Shift string array.vi"("Element in"=w1654, "Array in"=w1663) -> ("Array out"=w1662:string[])  [unwired: 8 in, 1 out]
                    n925 = call "Write in logger.vi"("String in"=w1654, "logger refnum"=w1655) -> ()  [unwired: 2 in, 2 out]
                  }
                  frame "Set field" {
                    n926 = Unbundle By Name(w1672) -> ("Experiment state"=w1685:T26)
                    n927 = local read "Magnet controls"() -> (w1701:T24)
                    n928 = Variant To Data(type=T36 {"Field [T]"=0.0, "Ramp [T/s]"=0.0, "Custom Ramp?"=TRUE, "Mode"=enum."Persistant"} ("Set Field"), Variant=w1703) -> (data=w1700:T36, error out=w1673:errorcluster)  [unwired: 1 in]
                    n929 = Unbundle By Name(w1682) -> ("Field [T]"=w1689:dbl)
                    n930 = case shown="\"Begin\"" w1685 {
                      selector: w1685 -> [w1705 _]
                      tunnel: [w1705 experiment_state."Acquisition" ("Value")] -> w1683
                      tunnel: w1678 -> [_ w1708]
                      tunnel: w1672 -> [w1704 w1706]
                      tunnel: [w1704 w1707] -> w1671
                      frame "Setup", Default {
                      }
                      frame "Begin" {
                        n931 = Bundle By Name(cluster=w1706, "Started"=w1708) -> (w1707:T25)
                      }
                    }
                    n932 = Unbundle By Name(w1700) -> ("Field [T]"=w1694:dbl, "Ramp [T/s]"=w1681:dbl, "Custom Ramp?"=w1699:bool)
                    n933 = Unbundle By Name(w1701) -> ("Desired\nramp [mT/s]"=w1698:dbl)
                    n934 = Not(x=w1699) -> (.not. x?=w1697:bool)
                    n935 = call <userlib>:"MGI Approximately Equal.vi"("Numeric 2"=w1698, "Numeric 1"=w1681) -> ("approx = ?"=w1696:bool)
                    n936 = Multiply(x=w1681, y=1000.0 ("x")) -> (x*y=w1679:dbl)
                    n937 = Or(x=w1697, y=w1696) -> (x .or. y?=w1693:bool)
                    n938 = Bundle By Name(cluster=w1671, "Experiment state"=w1683) -> (w1684:T25)
                    n939 = case shown="False" w1693 {
                      tunnel: ["Warning: Custom ramp was adjusted" ""] -> w1691
                      frame False {
                      }
                      frame True {
                      }
                    }
                    n940 = Format Into String(format string="Setting magnetic field from %f [T ] to %f [T] with ramp %f [mT/s]", error in=w1673, w1689, w1694, w1679) -> (resulting string=w1692:string, error out=w1674:errorcluster)  [unwired: 1 in]
                    n941 = Concatenate Strings(w1692, "\r", w1691) -> (w1675:string)
                    n942 = call "Add actual date time to string.vi"("String in"=w1675) -> ("String out"=w1688:string)  [unwired: 4 in]
                    n943 = local read "loggersRef"() -> (w1676:refnum<file>)
                    n944 = Bundle By Name(cluster=w1682, "Last update"=w1678, "Ramp [mT/s]"=w1679) -> (w1677:T83)
                    n945 = call "simple Shift string array.vi"("Element in"=w1688, "Array in"=w1686) -> ("Array out"=w1687:string[])  [unwired: 8 in, 1 out]
                    n946 = call "Write in logger.vi"("error in"=w1674, "String in"=w1675, "logger refnum"=w1676) -> ()  [unwired: 1 in, 2 out]
                  }
                  frame "Temperatures" {
                    n947 = local read "Temperature monitor"() -> (w1724:T12)
                    n948 = Variant To Data(type=T62 {"First stage A [K]"=0.0, "Second stage A [K]"=0.0, "Firs stage B [K]"=0.0, "Second stage B [K]"=0.0, "Inner magnet [K]"=0.0, "Outer Magnet [K]"=0.0, "Switch [K]"=0.0, "Support plate [K]"=0.0, "Time stamp"=0.0} ("LSC218 sensors"), Variant=w1741) -> (data=w1731:T62)  [unwired: 1 in, 1 out]
                    n949 = local read "Drift[K/s]"() -> (w1725:dbl[])
                    n950 = property on="VTI" class="Clust (strict)"() -> ("Value"=w1736:T84)  [unwired: 2 in, 2 out]
                    n951 = Cluster To Array(cluster=w1731) -> (array=w1721:dbl[])
                    n952 = Unbundle By Name(w1727) -> ("Field [T]"=w1726:dbl)
                    n953 = local read "Temperature log ref"() -> (w1739:refnum<file>)
                    n954 = Cluster To Array(cluster=w1724) -> (array=w1723:dbl[])
                    n955 = Unbundle By Name(w1736) -> ("VTI [K]"=w1729:dbl, "Sample [K]"=w1728:dbl, "Trap[K]"=w1735:dbl, "HePot [K]"=w1734:dbl)
                    n956 = Array Subset(array=w1721, length=8) -> (w1713:dbl[])  [unwired: 1 in]
                    n957 = Array Subset(array=w1723, length=8) -> (w1718:dbl[])  [unwired: 1 in]
                    n958 = Subtract(x=w1713, y=w1718) -> (x-y=w1720:dbl[])
                    n959 = Divide(x=w1720, y=2.5) -> (x/y=w1717:dbl[])
                    n960 = call "Bundle temperatures.vi"("Sample"=w1728, "VTI space"=w1729, "LSC218 sensors"=w1731) -> ("Tmp [K]"=→"Tmp [K]":T3)  [unwired: 8 in]
                    n961 = Build Array (concatenate)(w1713, w1729, w1728, w1735, w1734) -> (w1733:dbl[])
                    n962 = call "Log temperatures.vi"("LSC218 sensors"=w1731, "Time"=w1737, "Tmp logfile in"=w1739, "VTI"=w1729, "Sample"=w1728, "Trap"=w1735, "HePot"=w1734, "Field [T]"=w1726, "Logging interval (10s)"=10.0 ("Logging interval (20s)")) -> ("Tmp logfile ref"=w1714:refnum<file>)  [unwired: 4 in, 2 out]
                    n963 = Replace Array Subset(array=w1725, new element=w1717) -> (→"Drift[K/s]":dbl[])  [unwired: 1 in]
                    n964 = Array To Cluster(array=w1733) -> (cluster=w1732:T12)
                    n965 = local write "Temperature log ref"(w1714) -> ()
                    n966 = flat-sequence {
                      tunnel: w1732 -> [w1743]
                      tunnel: w1718 -> [_]
                      frame #0 {
                        "Temperature monitor" <- w1743
                      }
                    }
                  }
                  frame "End" {
                    n967 = local read "loggersRef"() -> (w1750:refnum<file>)
                    n968 = local read "Instr status"() -> (w1754:T1)
                    n969 = call "Add actual date time to string.vi"("String in"="Magnet ended") -> ("String out"=w1747:string)  [unwired: 4 in]
                    n970 = Bundle By Name(cluster=w1754, "Mag"=FALSE ("PSU")) -> (w1755:T1)
                    n971 = call "Write in logger.vi"("String in"=w1747, "logger refnum"=w1750) -> ()  [unwired: 2 in, 2 out]
                    n972 = local write "Instr status"(w1755) -> ()
                    n973 = control-ref of="Magnet controls"() -> (w1752:refnum<vi>)
                    n974 = call "simple Shift string array.vi"("Element in"=w1747, "Array in"=w1746) -> ("Array out"=w1745:string[])  [unwired: 8 in, 1 out]
                    n975 = property class="Clust (strict)"(reference=w1752, "DisabledEnum"=T34."Disabled and Grayed Out" ("Disabled")) -> ()  [unwired: 1 in, 2 out]
                  }
                  frame "Disconnect" {
                    n976 = local read "loggersRef"() -> (w1762:refnum<file>)
                    n977 = local read "Instr status"() -> (w1766:T1)
                    n978 = call "Add actual date time to string.vi"("String in"="Magnet dissconnected") -> ("String out"=w1759:string)  [unwired: 4 in]
                    n979 = Bundle By Name(cluster=w1766, "Mag"=FALSE ("PSU")) -> (w1767:T1)
                    n980 = call "Write in logger.vi"("String in"=w1759, "logger refnum"=w1762) -> ()  [unwired: 2 in, 2 out]
                    n981 = local write "Instr status"(w1767) -> ()
                    n982 = call "simple Shift string array.vi"("Element in"=w1759, "Array in"=w1758) -> ("Array out"=w1757:string[])  [unwired: 8 in, 1 out]
                    n983 = control-ref of="Magnet controls"() -> (w1764:refnum<vi>)
                    n984 = property class="Clust (strict)"(reference=w1764, "DisabledEnum"=T34."Disabled and Grayed Out" ("Disabled")) -> ()  [unwired: 1 in, 2 out]
                  }
                }
                n985 = Bundle By Name(cluster=w1455, "Magnet"=w1452) -> (w1453:T8)
              }
              frame "Excitation" {
                n986 = Unbundle By Name(w1771) -> ("THz"=w1770:T85)
                n987 = case shown="\"Connect\", \"Initialize\"" w1778 {
                  selector: w1778 -> [w1781 _ _ _ _ _]
                  tunnel: w1777 -> [w1780 w1836 w1839 w1869 w1875 w1891]
                  tunnel: [w1779 w1835 w1839 w1870 w1876 w1892] -> w1776
                  tunnel: w1775 -> [w1782 w1827 _ w1868 w1877 w1893]
                  tunnel: w1774 -> [_ w1807 _ w1845 w1879 w1895]
                  tunnel: w1772 -> [w1787 w1826 w1838 w1841 w1883 w1899]
                  tunnel: [w1787 w1826 w1838 w1857 w1883 w1899] -> w1773
                  tunnel: w1770 -> [w1786 w1821 w1837 w1847 w1882 w1898]
                  tunnel: [w1786 w1820 w1837 w1846 w1881 w1897] -> w1768
                  frame "Ignore", Default {
                    n988 = Match Pattern(string=w1781, regular expression="Error") -> (offset past match=w1785:i32)  [unwired: 1 in, 3 out]
                    n989 = Greater Or Equal To 0?(x=w1785) -> (x >= 0?=w1783:bool)
                    n990 = case shown="False" w1783 {
                      tunnel: w1780 -> [w1790 w1800]
                      tunnel: w1781 -> [w1789 w1799]
                      tunnel: [w1788 w1801] -> w1779
                      tunnel: w1782 -> [_ w1797]
                      frame False {
                        n991 = call "simple Shift string array.vi"("Element in"=w1789, "Array in"=w1790) -> ("Array out"=w1788:string[])  [unwired: 8 in, 1 out]
                      }
                      frame True {
                        n992 = Variant To Data(type=errorcluster {"status"=FALSE, "code"=0, "source"=""} ("error constant"), Variant=w1797) -> (data=w1795:errorcluster)  [unwired: 1 in, 1 out]
                        n993 = Unbundle By Name(w1795) -> ("source"=w1794:string)
                        n994 = call <vilib>:"Space Constant.vi"() -> ("String"=w1798:string)
                        n995 = Concatenate Strings("THz: " ("string"), w1799, w1798, w1794) -> (w1792:string)
                        n996 = local read "loggersRef"() -> (w1793:refnum<file>)
                        n997 = call "Write in logger.vi"("String in"=w1792, "logger refnum"=w1793) -> ()  [unwired: 2 in, 2 out]
                        n998 = call "simple Shift string array.vi"("Element in"=w1792, "Array in"=w1800) -> ("Array out"=w1801:string[])  [unwired: 8 in, 1 out]
                      }
                    }
                  }
                  frame "Connect", "Initialize" {
                    w1803 = T34."Disabled and Grayed Out" ("f")
                    w1804 = T34."Enabled" ("Disabled")
                    n999 = Variant To Data(type="", Variant=w1827) -> (data=w1825:string, error out=w1819:errorcluster)  [unwired: 1 in]
                    n1000 = call <vilib>:"Trim Whitespace.vi"("string"=w1825) -> ("trimmed string"=w1816:string)  [unwired: 1 in]
                    n1001 = Concatenate Strings("Initializing..." ("string"), w1825) -> (w1809:string)
                    n1002 = Match Pattern(string=w1816, regular expression="Device:") -> (after substring=w1817:string)  [unwired: 1 in, 3 out]
                    n1003 = Match Pattern(string=w1817, regular expression="Description:") -> (before substring=w1814:string, after substring=w1813:string)  [unwired: 1 in, 2 out]
                    n1004 = Match Pattern(string=w1813, regular expression="Connection:") -> (before substring=w1811:string, offset past match=w1810:i32)  [unwired: 1 in, 2 out]
                    n1005 = Greater Or Equal To 0?(x=w1810) -> (x >= 0?=w1802:bool)
                    n1006 = local read "Instr status"() -> (w1832:T1)
                    n1007 = Bundle By Name(cluster=w1821, "Name"=w1814, "Description"=w1811, "Last update"=w1807) -> (w1820:T85)
                    n1008 = Bundle By Name(cluster=w1832, "THz"=w1802) -> (w1833:T1)
                    n1009 = local write "Instr status"(w1833) -> ()
                    n1010 = Unbundle By Name(w1832) -> ("Mag"=w1831:bool, "MFLI"=w1830:bool)
                    n1011 = local read "loggersRef"() -> (w1828:refnum<file>)
                    n1012 = Compound Arithmetic op=AND(w1802, w1831, w1830) -> (w1829:bool)
                    n1013 = call "Add actual date time to string.vi"("String in"=w1809) -> ("String out"=w1824:string)  [unwired: 4 in]
                    n1014 = Select(t=w1804, s=w1829, f=w1803) -> (s? t:f=w1806:T34)
                    n1015 = Select(t=w1804, s=w1802, f=w1803) -> (s? t:f=w1805:T34)
                    n1016 = property on="Run script btn" class="Bool (strict)"(error in=w1819, "DisabledEnum"=w1806) -> (error out=w1823:errorcluster)  [unwired: 1 in, 1 out]
                    n1017 = call "Write in logger.vi"("error in"=w1823, "String in"=w1824, "logger refnum"=w1828) -> ("error out"=w1822:errorcluster)  [unwired: 1 in, 1 out]
                    n1018 = property on="THz control" class="Clust (strict)"("DisabledEnum"=w1805) -> ()  [unwired: 2 in, 2 out]
                    n1019 = call "simple Shift string array.vi"("Element in"=w1809, "Array in"=w1836) -> ("Array out"=w1835:string[])  [unwired: 8 in, 1 out]
                    n1020 = call <vilib>:"Clear Errors.vi"("error in (no error)"=w1822) -> ()  [unwired: 5 in, 2 out]
                  }
                  frame "Update" {
                  }
                  frame "Set parameters" {
                    n1021 = Variant To Data(type=T44 {"Start [GHz]"=8.0, "End [GHz] "=8.0, "Sweep up\ntime [ms]"=0.0, "Sweep down\ntime [ms]"=0.0, "Intermidiate [MHz]"=0.0, "Reset trigger"=FALSE} ("Sweep parameters"), Variant=w1868) -> (data=w1856:T44, error out=w1858:errorcluster)  [unwired: 1 in]
                    n1022 = Unbundle By Name(w1841) -> ("Experiment state"=w1840:T26)
                    n1023 = Unbundle By Name(w1856) -> ("Start [GHz]"=w1853:dbl, "End [GHz]"=w1852:dbl, "Sweep up\ntime [ms]"=w1851:dbl, "Intermidiate [MHz]"=w1855:dbl)
                    n1024 = local read "THz control"() -> (w1864:T22)
                    n1025 = Unbundle By Name(w1864) -> ("AMC"=w1865:u16, "Multip"=w1866:u16)
                    n1026 = Multiply(x=w1865, y=w1866) -> (x*y=w1854:u16)
                    n1027 = Multiply(x=w1853, y=w1854) -> (x*y=w1844:dbl)
                    n1028 = Multiply(x=w1852, y=w1854) -> (x*y=w1843:dbl)
                    n1029 = Multiply(x=w1851, y=w1854) -> (x*y=w1850:dbl)
                    n1030 = Multiply(x=w1855, y=w1854) -> (x*y=w1842:dbl)
                    n1031 = Equal To 0?(x=w1850) -> (x = 0?=w1862:bool)
                    n1032 = Select(t="CW", s=w1862, f="Sweep") -> (s? t:f=w1859:string)
                    n1033 = Bundle By Name(cluster=w1841, "Experiment state"=w1840) -> (w1857:T25)
                    n1034 = Format Into String(format string="THz source set to %s mode at %f GHz ", error in=w1858, w1859, w1844) -> (resulting string=w1849:string)  [unwired: 1 in, 1 out]
                    n1035 = Bundle By Name(cluster=w1847, "Last update"=w1845, "Start [GHz]"=w1844, "End [GHz]"=w1843, "Im Freq[MHz]"=w1842) -> (w1846:T85)
                    n1036 = call "Add actual date time to string.vi"("String in"=w1849) -> ("String out"=w1848:string)  [unwired: 4 in]
                    n1037 = call "simple Shift string array.vi"("Element in"=w1848, "Array in"=w1869) -> ("Array out"=w1870:string[])  [unwired: 8 in, 1 out]
                  }
                  frame "End" {
                    w1880 = "None" ("Master")
                    n1038 = Variant To Data(type="", Variant=w1877) -> (data=w1872:string)  [unwired: 1 in, 1 out]
                    n1039 = Bundle By Name(cluster=w1882, "Name"=w1880, "Description"=w1880, "Last update"=w1879) -> (w1881:T85)
                    n1040 = property on="THz" class="Bool (strict)"("Value"=FALSE) -> ()  [unwired: 2 in, 2 out]
                    n1041 = call "Add actual date time to string.vi"("String in"="Excitation module (VDI) ended") -> ("String out"=w1874:string)  [unwired: 4 in]
                    n1042 = Concatenate Strings(w1874, "\r\n", w1872) -> (w1873:string)
                    n1043 = local read "loggersRef"() -> (w1885:refnum<file>)
                    n1044 = call "Write in logger.vi"("String in"=w1873, "logger refnum"=w1885) -> ()  [unwired: 2 in, 2 out]
                    n1045 = call "simple Shift string array.vi"("Element in"=w1873, "Array in"=w1875) -> ("Array out"=w1876:string[])  [unwired: 8 in, 1 out]
                  }
                  frame "Disconnect" {
                    w1896 = "None" ("Master")
                    n1046 = Variant To Data(type="", Variant=w1893) -> (data=w1888:string)  [unwired: 1 in, 1 out]
                    n1047 = Bundle By Name(cluster=w1898, "Name"=w1896, "Description"=w1896, "Last update"=w1895) -> (w1897:T85)
                    n1048 = property on="THz" class="Bool (strict)"("Value"=FALSE) -> ()  [unwired: 2 in, 2 out]
                    n1049 = call "Add actual date time to string.vi"("String in"="Microwave excitation module Disconnected") -> ("String out"=w1890:string)  [unwired: 4 in]
                    n1050 = Concatenate Strings(w1890, "\r\n", w1888) -> (w1889:string)
                    n1051 = local read "loggersRef"() -> (w1901:refnum<file>)
                    n1052 = call "Write in logger.vi"("String in"=w1889, "logger refnum"=w1901) -> ()  [unwired: 2 in, 2 out]
                    n1053 = call "simple Shift string array.vi"("Element in"=w1889, "Array in"=w1891) -> ("Array out"=w1892:string[])  [unwired: 8 in, 1 out]
                  }
                }
                n1054 = Bundle By Name(cluster=w1771, "THz"=w1768) -> (w1769:T8)
              }
              frame "Digitizer" {
                n1055 = Unbundle By Name(w1906) -> ("THz"=w1905:T85)
                n1056 = case shown="\"Ignore\", Default" w1914 {
                  tunnel: w1913 -> [w1917]
                  tunnel: [w1917] -> w1912
                  tunnel: w1911 -> [_]
                  tunnel: w1910 -> [_]
                  tunnel: w1908 -> [w1916]
                  tunnel: [w1916] -> w1909
                  tunnel: w1907 -> [_]
                  tunnel: w1905 -> [w1915]
                  tunnel: [w1915] -> w1903
                  frame "Ignore", Default {
                  }
                }
                n1057 = Bundle By Name(cluster=w1906, "THz"=w1903) -> (w1904:T8)
              }
              frame "Carousel" {
                n1058 = Unbundle By Name(w1921) -> ("THz"=w1920:T85)
                n1059 = case shown="\"Ignore\", Default" w1929 {
                  tunnel: w1928 -> [w1932]
                  tunnel: [w1932] -> w1927
                  tunnel: w1926 -> [_]
                  tunnel: w1925 -> [_]
                  tunnel: w1923 -> [w1931]
                  tunnel: [w1931] -> w1924
                  tunnel: w1922 -> [_]
                  tunnel: w1920 -> [w1930]
                  tunnel: [w1930] -> w1918
                  frame "Ignore", Default {
                  }
                }
                n1060 = Bundle By Name(cluster=w1921, "THz"=w1918) -> (w1919:T8)
              }
              frame "Multimeter" {
                n1061 = Unbundle By Name(w1936) -> ("THz"=w1935:T85)
                n1062 = case shown="\"Get value\"" w1944 {
                  tunnel: w1943 -> [w1947 w1950]
                  tunnel: [w1947 w1950] -> w1942
                  tunnel: w1941 -> [_ _]
                  tunnel: w1940 -> [_ _]
                  tunnel: w1938 -> [w1946 w1949]
                  tunnel: [w1946 w1949] -> w1939
                  tunnel: w1937 -> [_ _]
                  tunnel: w1935 -> [w1945 w1948]
                  tunnel: [w1945 w1948] -> w1933
                  frame "Ignore", Default {
                  }
                  frame "Get value" {
                  }
                }
                n1063 = Bundle By Name(cluster=w1936, "THz"=w1933) -> (w1934:T8)
              }
              frame "Power monitor" {
                n1064 = Unbundle By Name(w1954) -> ("PwrMonitor"=w1953:T86)
                n1065 = case shown="\"Update\"" w1962 {
                  tunnel: w1961 -> [w1965 w1970 w1973]
                  tunnel: [w1965 w1970 w1973] -> w1960
                  tunnel: w1959 -> [_ w1968 _]
                  tunnel: w1958 -> [_ _ _]
                  tunnel: w1956 -> [w1964 w1969 w1972]
                  tunnel: [w1964 w1969 w1972] -> w1957
                  tunnel: w1955 -> [_ _ _]
                  tunnel: w1953 -> [w1963 _ w1971]
                  tunnel: [w1963 w1966 w1971] -> w1951
                  frame "Ignore", Default {
                  }
                  frame "Update" {
                    n1066 = Variant To Data(type=T63 {"Name"="", "Last update"=timestamp(0 s since 1904-01-01), "Outage?"=FALSE, "Low"=FALSE, "No battery"=FALSE, "Battery [%]"=0, "Charging"=FALSE} ("PwrM"), Variant=w1968) -> (data=w1966:T63)  [unwired: 1 in, 1 out]
                  }
                  frame "End" {
                  }
                }
                n1067 = Bundle By Name(cluster=w1954, "PwrMonitor"=w1951) -> (w1952:T8)
              }
              frame "SMU2450" {
                n1068 = Unbundle By Name(w1977) -> ("SMU"=w1976:T87)
                n1069 = case shown="\"Update\"" w1985 {
                  tunnel: w1984 -> [w1988 w2009 w2012 w2033 w2046 w2079 w2098]
                  tunnel: [w1988 w2008 w2012 w2034 w2046 w2080 w2099] -> w1983
                  tunnel: w1982 -> [_ w2004 _ w2032 w2063 w2081 w2100]
                  tunnel: w1981 -> [_ w1994 _ w2028 w2060 w2082 w2101]
                  tunnel: w1979 -> [w1987 w2003 w2011 w2027 w2059 w2086 w2105]
                  tunnel: [w1987 w2003 w2011 w2027 w2059 w2086 w2105] -> w1980
                  tunnel: w1978 -> [_ _ _ _ _ _ _]
                  tunnel: w1976 -> [w1986 w2001 w2010 w2030 w2062 w2085 w2104]
                  tunnel: [w1986 w2000 w2010 w2029 w2061 w2084 w2103] -> w1974
                  frame "Ignore", Default {
                  }
                  frame "Connect" {
                    n1070 = Variant To Data(type=T64 {"VISA name"="", "Connected"=FALSE, "Name"="", "Message"="", "Error message"="", "Min voltage"=0.0, "Max voltage"=0.0, "Min Current"=0.0, "Max Current"=0.0, "Measurement value"=0.0, "Source Voltage"=0.0, "Measurement"=FALSE, "Source Current"=0.0, "Source Mode"=0, "Measure Function"=0} ("output cluster"), Variant=w2004) -> (data=w1996:T64, error out=w1997:errorcluster)  [unwired: 1 in]
                    n1071 = Unbundle By Name(w1996) -> ("Name"=w1989:string, "Message"=w1991:string, "Connected"=w1995:bool)  [unwired: 1 out]
                    n1072 = local read "Instr status"() -> (w2006:T1)
                    n1073 = Bundle By Name(cluster=w2006, "SMU"=w1995) -> (w2007:T1)
                    n1074 = local write "Instr status"(w2007) -> ()
                    n1075 = Concatenate Strings(w1989, " connected. " ("string"), w1991) -> (w1990:string)
                    n1076 = Bundle By Name(cluster=w2001, "Name"=w1989, "Last update"=w1994) -> (w2000:T87)
                    n1077 = property on="SMU controls" class="Clust (strict)"("DisabledEnum"=T34."Enabled" ("Disabled")) -> ()  [unwired: 2 in, 2 out]
                    n1078 = local read "loggersRef"() -> (w2005:refnum<file>)
                    n1079 = call "Add actual date time to string.vi"("String in"=w1990) -> ("String out"=w1993:string)  [unwired: 4 in]
                    n1080 = call "Write in logger.vi"("error in"=w1997, "String in"=w1993, "logger refnum"=w2005) -> ("error out"=w2002:errorcluster)  [unwired: 1 in, 1 out]
                    n1081 = call "simple Shift string array.vi"("Element in"=w1993, "Array in"=w2009) -> ("Array out"=w2008:string[])  [unwired: 8 in, 1 out]
                    n1082 = call <vilib>:"Clear Errors.vi"("error in (no error)"=w2002) -> ()  [unwired: 5 in, 2 out]
                  }
                  frame "Update" {
                  }
                  frame "Set measurement" {
                    # "add surce funcion and value"
                    n1083 = Variant To Data(type=T64 {"VISA name"="", "Connected"=FALSE, "Name"="", "Message"="", "Error message"="", "Min voltage"=0.0, "Max voltage"=0.0, "Min Current"=0.0, "Max Current"=0.0, "Measurement value"=0.0, "Source Voltage"=0.0, "Measurement"=FALSE, "Source Current"=0.0, "Source Mode"=0, "Measure Function"=0} ("SMU status out"), Variant=w2032) -> (data=w2026:T64)  [unwired: 1 in, 1 out]
                    n1084 = Unbundle By Name(w2026) -> ("Measurement value"=w2014:dbl, "Measurement"=w2024:bool, "Source Voltage"=w2022:dbl, "Source Current"=w2023:dbl, "Source Mode"=w2016:u16, "Measure Function"=w2020:u16)
                    n1085 = case shown="0, Default" w2016 {
                      tunnel: w2023 -> [_ w2040]
                      tunnel: w2022 -> [w2038 _]
                      tunnel: [w2038 w2040] -> w2015
                      tunnel: ["Voltage" "Current"] -> w2021
                      frame 0, Default {
                      }
                      frame 1 {
                      }
                    }
                    n1086 = case shown="0, Default" w2020 {
                      tunnel: ["Voltage" "Current"] -> w2019
                      frame 0, Default {
                      }
                      frame 1 {
                      }
                    }
                    n1087 = local read "SMU controls"() -> (w2018:T14)
                    n1088 = Bundle By Name(cluster=w2018, "Measurement settings.Source Mode"=w2016, "Measurement settings.Source Level"=w2015, "Value"=w2014) -> (w2017:T14)
                    n1089 = Bundle By Name(cluster=w2030, "Last update"=w2028, "MeasValue"=w2014, "Output"=w2024, "SourFunc"=w2021, "SourValue"=w2015, "MeasFunc"=w2019) -> (w2029:T87)
                    n1090 = local write "SMU controls"(w2017) -> ()
                    n1091 = call "Add actual date time to string.vi"("String in"="SMU set") -> ("String out"=w2031:string)  [unwired: 4 in]
                    n1092 = call "simple Shift string array.vi"("Element in"=w2031, "Array in"=w2033) -> ("Array out"=w2034:string[])  [unwired: 8 in, 1 out]
                  }
                  frame "Get actual results" {
                    # "add surce funcion and value"
                    n1093 = Variant To Data(type=T64 {"VISA name"="", "Connected"=FALSE, "Name"="", "Message"="", "Error message"="", "Min voltage"=0.0, "Max voltage"=0.0, "Min Current"=0.0, "Max Current"=0.0, "Measurement value"=0.0, "Source Voltage"=0.0, "Measurement"=FALSE, "Source Current"=0.0, "Source Mode"=0, "Measure Function"=0} ("SMU status out"), Variant=w2063) -> (data=w2058:T64)  [unwired: 1 in, 1 out]
                    n1094 = Unbundle By Name(w2058) -> ("Measurement value"=w2044:dbl, "Measurement"=w2056:bool, "Source Voltage"=w2054:dbl, "Source Current"=w2055:dbl, "Source Mode"=w2048:u16, "Measure Function"=w2047:u16)
                    n1095 = Add(x=w2044, y=3.7e-06) -> (x+y=w2042:dbl)
                    n1096 = case shown="1" w2048 {
                      tunnel: w2055 -> [_ w2069]
                      tunnel: w2054 -> [w2067 _]
                      tunnel: [w2067 w2069] -> w2053
                      tunnel: ["Voltage" "Current"] -> w2052
                      frame 0, Default {
                      }
                      frame 1 {
                      }
                    }
                    n1097 = case shown="0, Default" w2047 {
                      tunnel: ["Voltage" "Current"] -> w2051
                      frame 0, Default {
                      }
                      frame 1 {
                      }
                    }
                    n1098 = Divide(x=w2042, y=0.00998) -> (x/y=w2045:dbl)
                    n1099 = local read "SMU controls"() -> (w2050:T14)
                    n1100 = Bundle By Name(cluster=w2050, "Value"=w2042, "B[T]"=w2045) -> (w2049:T14)
                    n1101 = Bundle By Name(cluster=w2062, "Last update"=w2060, "MeasValue"=w2044, "Output"=w2056, "SourFunc"=w2052, "SourValue"=w2053, "MeasFunc"=w2051) -> (w2061:T87)
                    n1102 = local write "SMU controls"(w2049) -> ()
                  }
                  frame "End" {
                    n1103 = Variant To Data(type=T64 {"VISA name"="", "Connected"=FALSE, "Name"="", "Message"="", "Error message"="", "Min voltage"=0.0, "Max voltage"=0.0, "Min Current"=0.0, "Max Current"=0.0, "Measurement value"=0.0, "Source Voltage"=0.0, "Measurement"=FALSE, "Source Current"=0.0, "Source Mode"=0, "Measure Function"=0} ("SMU status out"), Variant=w2081) -> (data=w2074:T64)  [unwired: 1 in, 1 out]
                    n1104 = Unbundle By Name(w2074) -> ("Name"=w2072:string, "Measurement"=w2070:bool)
                    n1105 = Bundle By Name(cluster=w2085, "Name"="None" ("Master"), "Output"=w2070, "Last update"=w2082) -> (w2084:T87)
                    n1106 = property on="SMU" class="Bool (strict)"("Value"=FALSE) -> ()  [unwired: 2 in, 2 out]
                    n1107 = Concatenate Strings("SMU module " ("String in"), w2072, " ended." ("string")) -> (w2073:string)
                    n1108 = call "Add actual date time to string.vi"("String in"=w2073) -> ("String out"=w2078:string)  [unwired: 4 in]
                    n1109 = Concatenate Strings(w2078, "\r\n") -> (w2077:string)
                    n1110 = local read "loggersRef"() -> (w2088:refnum<file>)
                    n1111 = call "Write in logger.vi"("String in"=w2077, "logger refnum"=w2088) -> ()  [unwired: 2 in, 2 out]
                    n1112 = call "simple Shift string array.vi"("Element in"=w2077, "Array in"=w2079) -> ("Array out"=w2080:string[])  [unwired: 8 in, 1 out]
                  }
                  frame "Disconnect" {
                    n1113 = Variant To Data(type=T64 {"VISA name"="", "Connected"=FALSE, "Name"="", "Message"="", "Error message"="", "Min voltage"=0.0, "Max voltage"=0.0, "Min Current"=0.0, "Max Current"=0.0, "Measurement value"=0.0, "Source Voltage"=0.0, "Measurement"=FALSE, "Source Current"=0.0, "Source Mode"=0, "Measure Function"=0} ("SMU status out"), Variant=w2100) -> (data=w2095:T64)  [unwired: 1 in, 1 out]
                    n1114 = Unbundle By Name(w2095) -> ("Name"=w2091:string, "Measurement"=w2090:bool)
                    n1115 = Bundle By Name(cluster=w2104, "Name"="None" ("Master"), "Output"=w2090, "Last update"=w2101) -> (w2103:T87)
                    n1116 = property on="SMU" class="Bool (strict)"("Value"=FALSE) -> ()  [unwired: 2 in, 2 out]
                    n1117 = Concatenate Strings(w2091, " SMU disconnected." ("String in")) -> (w2092:string)
                    n1118 = call "Add actual date time to string.vi"("String in"=w2092) -> ("String out"=w2097:string)  [unwired: 4 in]
                    n1119 = Concatenate Strings(w2097, "\r\n") -> (w2096:string)
                    n1120 = local read "loggersRef"() -> (w2107:refnum<file>)
                    n1121 = call "Write in logger.vi"("String in"=w2096, "logger refnum"=w2107) -> ()  [unwired: 2 in, 2 out]
                    n1122 = call "simple Shift string array.vi"("Element in"=w2096, "Array in"=w2098) -> ("Array out"=w2099:string[])  [unwired: 8 in, 1 out]
                  }
                }
                n1123 = Bundle By Name(cluster=w1977, "SMU"=w1974) -> (w1975:T8)
              }
              frame "Acquisition" {
                n1124 = Unbundle By Name(w2110) -> ("MFLI"=w2113:T88)
                n1125 = case shown="\"Get point\"" w2119 {
                  tunnel: w2118 -> [w2144 w2160 w2182 w2201 w2210 w2229 w2239 w2248 _]
                  tunnel: w2117 -> [w2123 w2152 w2176 w2198 w2208 _ _ _ _]
                  tunnel: [w2128 w2156 w2181 w2192 w2211 w2230 w2233 w2242 w2250] -> w2114
                  tunnel: w2115 -> [w2129 w2157 w2181 w2192 w2211 w2230 w2234 w2243 w2250]
                  tunnel: w2113 -> [w2124 w2153 w2179 w2187 w2205 w2226 w2231 w2240 w2249]
                  tunnel: [w2121 w2147 w2177 w2187 w2205 w2226 w2231 w2240 w2249] -> w2112
                  tunnel: w2109 -> [_ _ _ _ _ w2219 _ _ _]
                  frame "Initialize" {
                    w2136 = TRUE ("PSU")
                    w2135 = T34."Enabled" ("Disabled")
                    n1126 = Variant To Data(type="", Variant=w2144) -> (data=w2122:string)  [unwired: 1 in, 1 out]
                    n1127 = Bundle By Name(cluster=w2124, "Last update"=w2123, "Lock-in"=w2122, "Multimeter"="Unknown") -> (w2121:T88)
                    n1128 = local read "Instr status"() -> (w2139:T1)
                    n1129 = Bundle By Name(cluster=w2139, "MFLI"=w2136) -> (w2141:T1)
                    n1130 = Unbundle By Name(w2139) -> ("THz"=w2138:bool, "Mag"=w2137:bool)
                    n1131 = local write "Instr status"(w2141) -> ()
                    n1132 = control-ref of="Acquisition controls"() -> (w2140:refnum<vi>)
                    n1133 = Compound Arithmetic op=AND(w2138, w2137, w2136) -> (w2134:bool)
                    n1134 = Concatenate Strings(w2122, " connected as ACQ" ("String in")) -> (w2126:string)
                    n1135 = Select(t=w2135, s=w2134, f=T34."Disabled and Grayed Out" ("Disabled")) -> (s? t:f=w2130:T34)
                    n1136 = property class="Clust (strict)"(reference=w2140, "DisabledEnum"=w2135) -> ()  [unwired: 1 in, 2 out]
                    n1137 = local read "loggersRef"() -> (w2133:refnum<file>)
                    n1138 = control-ref of="Run script btn"() -> (w2132:refnum<vi>)
                    n1139 = call "Add actual date time to string.vi"("String in"=w2126) -> ("String out"=w2125:string)  [unwired: 4 in]
                    n1140 = Build Array(w2132) -> (w2131:refnum<vi>[])
                    n1141 = call "Write in logger.vi"("String in"=w2125, "logger refnum"=w2133) -> ()  [unwired: 2 in, 2 out]
                    n1142 = call "Dis- or en- able controls.vi"("Disabled"=w2130, "Control referencies"=w2131) -> ()  [unwired: 9 in, 1 out]
                    n1143 = call "simple Shift string array.vi"("Element in"=w2125, "Array in"=w2129) -> ("Array out"=w2128:string[])  [unwired: 8 in, 1 out]
                  }
                  frame "Set parameters" {
                    n1144 = Variant To Data(type=T19 {"Filter order"=1.0, "Filter tau [ms]"=1.0, "F_Mod [kHz]"=0.0, "Amp_Mod [mV]"=0.0, "Enable output"=0, "Phase [°]"=0.0} ("ACQ parameters"), Variant=w2160) -> (data=w2145:T19)  [unwired: 1 in, 1 out]
                    n1145 = local read "Acquisition controls"() -> (w2146:T21)
                    n1146 = Unbundle By Name(w2145) -> ("F_Mod [kHz]"=w2151:dbl, "Amp_Mod [mV]"=w2150:dbl, "Enable output"=w2149:u16)
                    n1147 = property on="ACQ parameters" class="Clust (strict)"("Value"=w2145) -> ()  [unwired: 2 in, 2 out]
                    n1148 = Bundle By Name(cluster=w2146, "ACQ parameters"=w2145) -> (w2158:T21)
                    n1149 = Greater Or Equal To 0?(x=w2149) -> (x >= 0?=w2148:bool)
                    n1150 = local write "Acquisition controls"(w2158) -> ()
                    n1151 = call "Add actual date time to string.vi"("String in"="Lock-in: parameters set" ("Element in")) -> ("String out"=w2154:string)  [unwired: 4 in]
                    n1152 = call "simple Shift string array.vi"("Element in"=w2154, "Array in"=w2157) -> ("Array out"=w2156:string[])  [unwired: 8 in, 1 out]
                    n1153 = Bundle By Name(cluster=w2153, "Last update"=w2152, "Freq [kHz]"=w2151, "Ampl [mV]"=w2150, "OutEn"=w2148) -> (w2147:T88)
                  }
                  frame "Update" {
                    w2173 = 1000.0 ("x")
                    n1154 = Variant To Data(type=T65 {"In50"=FALSE, "InAC"=FALSE, "InDiff"=FALSE, "Out50"=FALSE, "OutEN"=FALSE, "OutF[Hz]"=0.0, "OutA[V]"=0.0, "DemEN"=FALSE, "Const[ms]"=0.0, "Order[-]"=0, "Phase [°]"=0.0} ("Lock-in info"), Variant=w2182) -> (data=w2178:T65)  [unwired: 1 in, 1 out]
                    n1155 = Unbundle By Name(w2178) -> ("OutF[Hz]"=w2175:dbl, "OutA[V]"=w2174:dbl, "OutEN"=w2169:bool, "Out50"=w2166:bool, "In50"=w2163:bool, "Order[-]"=w2165:i32, "Const[ms]"=w2164:dbl, "DemEN"=w2162:bool, "Phase [°]"=w2161:dbl)
                    n1156 = Divide(x=w2175, y=w2173) -> (x/y=w2168:dbl)
                    n1157 = Multiply(x=w2174, y=w2173) -> (x*y=w2167:dbl)
                    n1158 = Boolean To (0,1)(Boolean=w2169) -> (0, 1=w2170:i16)
                    n1159 = local read "Acquisition controls"() -> (w2172:T21)
                    n1160 = Bundle By Name(cluster=w2172, "ACQ parameters.Enable output"=w2170, "ACQ parameters.F_Mod [kHz]"=w2168, "ACQ parameters.Amp_Mod [mV]"=w2167, "Out50"=w2166, "In50"=w2163, "ACQ parameters.Filter order"=w2165, "ACQ parameters.Filter tau [ms]"=w2164, "DemEn"=w2162, "ACQ parameters.Phase [°]"=w2161) -> (w2171:T21)
                    n1161 = Bundle By Name(cluster=w2179, "Last update"=w2176, "Freq [kHz]"=w2168, "Ampl [mV]"=w2167, "OutEn"=w2169, "In50 Ohm"=w2163, "DemEn"=w2162) -> (w2177:T88)
                    n1162 = local write "Acquisition controls"(w2171) -> ()
                  }
                  frame "Get point" {
                    n1163 = local read "Acquisition controls"() -> (w2186:T21)
                    n1164 = Variant To Data(type=T67 {"Timestamps (ticks)"=0, "X (Vrms)"=0.0, "Y (Vrms)"=0.0, "Osc Phase (deg)"=0.0, "Freq (Hz)"=0.0, "DIO"=0, "AuxIn0 (V)"=0.0, "AuxIn1 (V)"=0.0, "Trigger"=0} ("Update data"), Variant=w2201) -> (data=w2199:T67)  [unwired: 1 in, 1 out]
                    n1165 = Unbundle By Name(w2199) -> ("X (Vrms)"=w2190:dbl, "Y (Vrms)"=w2189:dbl, "AuxIn0 (V)"=w2185:dbl, "AuxIn1 (V)"=w2184:dbl)
                    n1166 = Unbundle By Name(w2186) -> ("ACQ shot btn"=w2193:bool)
                    n1167 = Bundle By Name(cluster=w2186, "AuxIn0 [V]"=w2185, "AuxIn1 [V]"=w2184) -> (w2183:T21)
                    n1168 = local read "Tab Control"() -> (w2196:T6)
                    n1169 = local write "Acquisition controls"(w2183) -> ()
                    n1170 = Build Array(w2190, w2189) -> (→"Data":dbl[])
                    n1171 = Equal?(x=w2196, y=T66."Adjustment" ("Tab Control")) -> (x = y?=w2195:bool)
                    n1172 = And(x=w2195, y=w2193) -> (x .and. y?=w2194:bool)
                    n1173 = case shown="True" w2194 {
                      tunnel: w2190 -> [_ w2204]
                      tunnel: w2189 -> [_ w2203]
                      frame False {
                      }
                      frame True {
                        n1174 = Bundle("X (Vrms)"=w2204, "Y (Vrms)"=w2203) -> (→"lookup":cluster{"X (Vrms)":dbl, "Y (Vrms)":dbl})  [unwired: 1 in]
                      }
                    }
                    "New data" <- TRUE ("New data")
                    "data time" <- w2198
                  }
                  frame "Get array" {
                    n1175 = Variant To Data(type=dbl[] [], Variant=w2210) -> (data=w2206:dbl[])  [unwired: 1 in, 1 out]
                    n1176 = local write "data time"(w2208) -> ()
                    n1177 = local write "New data"(TRUE ("New data")) -> ()
                    n1178 = local write "Data"(w2206) -> ()
                  }
                  frame "Get ModA" {
                    n1179 = Variant To Data(type=0.0, Variant=w2229) -> (data=w2212:dbl)  [unwired: 1 in, 1 out]
                    n1180 = local read "Acquisition controls"() -> (w2225:T21)
                    n1181 = Unbundle By Name(w2225) -> ("Sample holder"=w2213:T20, "ACQ parameters.Amp_Mod [mV]"=w2222:dbl)
                    n1182 = local read "Acquisition controls"() -> (w2224:T21)
                    n1183 = Unbundle By Name(w2224) -> ("Desired [G]"=w2223:dbl, "Auto-modulation"=w2218:bool, "ACQ parameters.Enable output"=w2217:u16)
                    n1184 = call "Modulation current to field conversion.vi"("Sample holder"=w2213, "Modulation current (mA)"=w2212) -> ("Modulation field (G)"=w2214:dbl)  [unwired: 9 in]
                    n1185 = Unbundle By Name(w2219) -> ("Tmp_C"=w2220:refnum<queue>)
                    n1186 = Greater Than 0?(x=w2217) -> (x > 0?=w2215:bool)
                    n1187 = And(x=w2218, y=w2215) -> (x .and. y?=w2216:bool)
                    n1188 = call "Modulation amplitude auto adjustment.vi"("Amp_Mod [mV]"=w2222, "Enable auto adjustment"=w2216, "Actual [G]"=w2214, "Desired [G]"=w2223, "Queue in"=w2220) -> ("Adjusted"=w2221:bool)  [unwired: 6 in]
                    n1189 = Bundle By Name(cluster=w2224, "Modulation [A]"=w2212, "Actual [G]"=w2214, "Adj mod"=w2221) -> (w2227:T21)
                    n1190 = local write "Acquisition controls"(w2227) -> ()
                  }
                  frame "End" {
                    n1191 = Variant To Data(type=T68 {"handleValid"=FALSE, "Conn"=0, "Path Prefix"="", "Handle"=0, "Connected"=FALSE, "Clockbase(s)"=0.0} ("Handle Out"), Variant=w2239) -> ()  [unwired: 1 in, 2 out]
                    n1192 = local read "loggersRef"() -> (w2236:refnum<file>)
                    n1193 = property on="MFLI" class="Bool (strict)"("Value"=FALSE) -> ()  [unwired: 2 in, 2 out]
                    n1194 = call "Add actual date time to string.vi"("String in"="ACQ Ended") -> ("String out"=w2232:string)  [unwired: 4 in]
                    n1195 = call "Write in logger.vi"("String in"=w2232, "logger refnum"=w2236) -> ()  [unwired: 2 in, 2 out]
                    n1196 = call "simple Shift string array.vi"("Element in"=w2232, "Array in"=w2234) -> ("Array out"=w2233:string[])  [unwired: 8 in, 1 out]
                  }
                  frame "Disconnect" {
                    n1197 = Variant To Data(type=T68 {"handleValid"=FALSE, "Conn"=0, "Path Prefix"="", "Handle"=0, "Connected"=FALSE, "Clockbase(s)"=0.0} ("Handle Out"), Variant=w2248) -> ()  [unwired: 1 in, 2 out]
                    n1198 = local read "loggersRef"() -> (w2245:refnum<file>)
                    n1199 = property on="MFLI" class="Bool (strict)"("Value"=FALSE) -> ()  [unwired: 2 in, 2 out]
                    n1200 = call "Add actual date time to string.vi"("String in"="ACQ disconnected") -> ("String out"=w2241:string)  [unwired: 4 in]
                    n1201 = call "Write in logger.vi"("String in"=w2241, "logger refnum"=w2245) -> ()  [unwired: 2 in, 2 out]
                    n1202 = call "simple Shift string array.vi"("Element in"=w2241, "Array in"=w2243) -> ("Array out"=w2242:string[])  [unwired: 8 in, 1 out]
                  }
                  frame "Ignore", Default {
                  }
                }
                n1203 = Bundle By Name(cluster=w2110, "MFLI"=w2112) -> (w2111:T8)
              }
              frame "VTI" {
                n1204 = Unbundle By Name(w2256) -> ("VTI"=w2254:T84)
                n1205 = case shown="\"Update\"" w2261 {
                  tunnel: w2260 -> [_ w2281 w2316 w2332 _ _]
                  tunnel: w2259 -> [w2264 w2279 w2314 w2328 w2365 w2378]
                  tunnel: [w2264 w2278 w2314 w2327 w2364 w2377] -> w2258
                  tunnel: w2251 -> [w2263 w2269 w2312 w2330 w2360 w2373]
                  tunnel: [w2263 w2269 w2311 w2330 w2360 w2373] -> w2257
                  tunnel: w2254 -> [w2262 w2268 w2299 w2329 w2359 w2372]
                  tunnel: w2253 -> [_ _ w2303 _ _ _]
                  tunnel: [w2262 w2267 w2310 w2329 w2358 w2371] -> w2252
                  frame "Ignore", Default {
                  }
                  frame "Initialize" {
                    n1206 = Variant To Data(type="", Variant=w2281) -> (data=w2266:string)  [unwired: 1 in, 1 out]
                    n1207 = local read "Instr status"() -> (w2275:T1)
                    n1208 = Bundle By Name(cluster=w2275, "VTI"=TRUE) -> (w2274:T1)
                    n1209 = local write "Instr status"(w2274) -> ()
                    n1210 = Concatenate Strings("Temperature controller " ("string"), w2266, " initialized" ("string")) -> (w2270:string)
                    n1211 = local read "loggersRef"() -> (w2271:refnum<file>)
                    n1212 = call "Add actual date time to string.vi"("String in"=w2270) -> ("String out"=w2272:string)  [unwired: 4 in]
                    n1213 = call "Write in logger.vi"("String in"=w2272, "logger refnum"=w2271) -> ()  [unwired: 2 in, 2 out]
                    n1214 = property on="VTI control" class="Clust (strict)"("DisabledEnum"=T34."Enabled" ("Disabled")) -> ()  [unwired: 2 in, 2 out]
                    n1215 = Bundle By Name(cluster=w2268, "TempCtl"=w2266) -> (w2267:T84)
                    n1216 = call "simple Shift string array.vi"("Element in"=w2270, "Array in"=w2279) -> ("Array out"=w2278:string[])  [unwired: 8 in, 1 out]
                  }
                  frame "Update" {
                    n1217 = Variant To Data(type=T69 {"VTI space"=0.0, "Sample"=0.0, "He pot"=0.0, "Trap"=0.0, "Ambient"=0.0, "SetP_VTI"=0.0, "SetP_Smp"=0.0, "SetP_Pot"=0.0, "SetP_Trap"=0.0, "Range out 1"=1, "Out 1 [%]"=0.0, "Out 2 [%]"=0.0} ("TC sensors [K]"), Variant=w2316) -> (data=w2313:T69)  [unwired: 1 in, 1 out]
                    n1218 = Unbundle(w2313) -> ("VTI space"=w2285:dbl, "Sample"=w2282:dbl, "He pot"=w2283:dbl, "Trap"=w2284:dbl, "Ambient"=w2290:dbl, "SetP_VTI"=w2307:dbl, "SetP_Smp"=w2306:dbl, "SetP_Pot"=w2305:dbl, "SetP_Trap"=w2304:dbl, "Range out 1"=w2286:u16, "Out 1 [%]"=w2288:dbl, "Out 2 [%]"=w2287:dbl)
                    n1219 = Unbundle(w2299) -> ("VTI [K]"=w2295:dbl, "Sample [K]"=w2296:dbl, "Trap[K]"=w2297:dbl, "HePot [K]"=w2298:dbl)  [unwired: 3 out]
                    n1220 = local read "VTI control"() -> (w2309:T18)
                    n1221 = Bundle By Name(cluster=w2312, "T_sample [K]"=w2282) -> (w2311:T25)
                    n1222 = Build Array(w2285, w2282, w2284, w2283) -> (w2291:dbl[])
                    n1223 = Bundle By Name(cluster=w2299, "Last update"=w2303, "VTI [K]"=w2285, "Sample [K]"=w2282, "HePot [K]"=w2283, "Trap[K]"=w2284, "Ambient [K]"=w2290) -> (w2310:T84)
                    n1224 = Build Array(w2295, w2296, w2297, w2298) -> (w2294:dbl[])
                    n1225 = Bundle(cluster=w2309, "VTI space [K]"=w2307, "Sample [K]"=w2306, "Heater3 [K]"=w2305, "Heater4 [K]"=w2304, "Out 1 [%]"=w2288, "Out 2 [%]"=w2287, "Range out 1"=w2286) -> (w2308:T18)
                    n1226 = Subtract(x=w2291, y=w2294) -> (x-y=w2293:dbl[])
                    n1227 = local read "Drift[K/s]"() -> (w2302:dbl[])
                    n1228 = local write "VTI control"(w2308) -> ()
                    n1229 = Divide(x=w2293, y=2.0) -> (x/y=w2289:dbl[])
                    n1230 = Replace Array Subset(array=w2302, new element=w2289, index=8) -> (w2300:dbl[])
                    n1231 = local write "Drift[K/s]"(w2300) -> ()
                  }
                  frame "Set point" {
                    n1232 = Variant To Data(type=T50 {"Heater"="", "Tmp [K]"=0.0}, Variant=w2332) -> (data=w2331:T50)  [unwired: 1 in, 1 out]
                    n1233 = Unbundle By Name(w2331) -> ("Heater"=w2321:string, "Tmp [K]"=w2318:dbl)
                    n1234 = local read "VTI control"() -> (w2320:T18)
                    n1235 = case shown="\"VTI space [K]\"" w2321 {
                      selector: w2321 -> [_ w2336 w2341 w2349 w2354]
                      tunnel: [u16 0 ("Output's Control Loop (1:1)") w2340 w2345 w2350 w2355] -> _
                      tunnel: w2318 -> [_ w2337 w2342 w2346 w2351]
                      tunnel: w2320 -> [w2334 w2339 w2344 w2348 w2353]
                      tunnel: [w2334 w2338 w2343 w2347 w2352] -> w2319
                      tunnel: ["Unknown setpoint" w2336 w2341 w2349 w2354] -> w2317
                      frame "None", Default {
                      }
                      frame "VTI space [K]" {
                        w2340 = u16 1 items=["1"=1, "2"=2, "3"=3, "4"=4] ("Output's Control Loop (1:1)")
                        n1236 = Bundle By Name(cluster=w2339, "VTI space [K]"=w2337) -> (w2338:T18)
                      }
                      frame "Sample [K]" {
                        w2345 = u16 2 items=["1"=1, "2"=2, "3"=3, "4"=4] ("Output's Control Loop (1:1)")
                        n1237 = Bundle By Name(cluster=w2344, "Sample [K]"=w2342) -> (w2343:T18)
                      }
                      frame "Heater3 [K]" {
                        w2350 = u16 3 items=["1"=1, "2"=2, "3"=3, "4"=4] ("Output's Control Loop (1:1)")
                        n1238 = Bundle By Name(cluster=w2348, "Heater3 [K]"=w2346) -> (w2347:T18)
                      }
                      frame "Heater4 [K]" {
                        w2355 = u16 4 items=["1"=1, "2"=2, "3"=3, "4"=4] ("Output's Control Loop (1:1)")
                        n1239 = Bundle By Name(cluster=w2353, "Heater4 [K]"=w2351) -> (w2352:T18)
                      }
                    }
                    n1240 = local write "VTI control"(w2319) -> ()
                    n1241 = Format Into String(format string="%f K", initial string=w2317, w2318) -> (resulting string=w2325:string)  [unwired: 1 in, 1 out]
                    n1242 = local read "loggersRef"() -> (w2326:refnum<file>)
                    n1243 = call "Add actual date time to string.vi"("String in"=w2325) -> ("String out"=w2323:string)  [unwired: 4 in]
                    n1244 = call "simple Shift string array.vi"("Element in"=w2323, "Array in"=w2328) -> ("Array out"=w2327:string[])  [unwired: 8 in, 1 out]
                    n1245 = call "Write in logger.vi"("String in"=w2323, "logger refnum"=w2326) -> ()  [unwired: 2 in, 2 out]
                  }
                  frame "End" {
                    w2362 = "VTI closed" ("Element in")
                    n1246 = local read "Instr status"() -> (w2368:T1)
                    n1247 = Bundle By Name(cluster=w2359, "TempCtl"="None" ("TC")) -> (w2358:T84)
                    n1248 = Bundle By Name(cluster=w2368, "VTI"=FALSE) -> (w2366:T1)
                    n1249 = local write "Instr status"(w2366) -> ()
                    n1250 = property on="VTI control" class="Clust (strict)"("DisabledEnum"=T34."Disabled and Grayed Out" ("Disabled")) -> ()  [unwired: 2 in, 2 out]
                    n1251 = call "Add actual date time to string.vi"("String in"=w2362) -> ("String out"=w2361:string)  [unwired: 4 in]
                    n1252 = local read "loggersRef"() -> (w2363:refnum<file>)
                    n1253 = call "simple Shift string array.vi"("Element in"=w2362, "Array in"=w2365) -> ("Array out"=w2364:string[])  [unwired: 8 in, 1 out]
                    n1254 = call "Write in logger.vi"("String in"=w2361, "logger refnum"=w2363) -> ()  [unwired: 2 in, 2 out]
                  }
                  frame "Disconnect" {
                    w2375 = "VTI Disconnected" ("Element in")
                    n1255 = local read "Instr status"() -> (w2381:T1)
                    n1256 = Bundle By Name(cluster=w2372, "TempCtl"="None" ("TC")) -> (w2371:T84)
                    n1257 = Bundle By Name(cluster=w2381, "VTI"=FALSE) -> (w2379:T1)
                    n1258 = local write "Instr status"(w2379) -> ()
                    n1259 = property on="VTI control" class="Clust (strict)"("DisabledEnum"=T34."Disabled and Grayed Out" ("Disabled")) -> ()  [unwired: 2 in, 2 out]
                    n1260 = call "Add actual date time to string.vi"("String in"=w2375) -> ("String out"=w2374:string)  [unwired: 4 in]
                    n1261 = local read "loggersRef"() -> (w2376:refnum<file>)
                    n1262 = call "simple Shift string array.vi"("Element in"=w2375, "Array in"=w2378) -> ("Array out"=w2377:string[])  [unwired: 8 in, 1 out]
                    n1263 = call "Write in logger.vi"("String in"=w2374, "logger refnum"=w2376) -> ()  [unwired: 2 in, 2 out]
                  }
                }
                n1264 = Bundle By Name(cluster=w2256, "VTI"=w2252) -> (w2255:T8)
              }
              frame "Servo" {
                n1265 = Unbundle By Name(w2386) -> ("Servo"=w2384:T10[])
                n1266 = case shown="\"Initialize\"" w2388 {
                  selector: w2388 -> [w2408 w2456 w2509 _ _ w2651]
                  tunnel: w2391 -> [w2410 w2458 w2516 _ _ w2649]
                  tunnel: w2390 -> [w2406 w2454 w2512 w2595 w2635 w2654]
                  tunnel: [w2407 w2455 w2513 w2596 w2636 w2653] -> w2389
                  tunnel: w2384 -> [w2393 w2442 w2495 w2563 w2628 w2643]
                  tunnel: [w2392 w2444 w2494 w2592 w2631 w2643] -> w2383
                  tunnel: w2382 -> [w2394 _ w2492 _ _ _]
                  frame "Initialize" {
                    n1267 = Variant To Data(type=T70[] [] ("Servo status"), Variant=w2410) -> (data=w2396:T70[])  [unwired: 1 in, 1 out]
                    n1268 = Index Array(array=w2393) -> (element=w2395:T10)  [unwired: 1 in]
                    n1269 = for {
                      tunnel: w2396 -> [w2426] mode=indexing
                      tunnel: w2395 -> [w2422]
                      tunnel: w2394 -> [w2420]
                      tunnel: [w2414] -> w2392 mode=indexing
                      n1270 = Unbundle By Name(w2426) -> ("Servo constants.Name"=w2421:T11, "Servo variables.Actual position"=w2419:dbl, "Servo constants.Pos position limit [mm]"=w2416:dbl, "Servo constants.Neg position limit [mm]"=w2415:dbl, "Servo variables.Power ON"=w2417:bool, "Servo variables.Connected"=w2418:bool)
                      n1271 = Select(t=T34."Enabled" ("Disabled"), s=w2418, f=T34."Disabled and Grayed Out" ("Disabled")) -> (s? t:f=w2423:T34)
                      n1272 = Bundle By Name(cluster=w2422, "Name"=w2421, "Last update"=w2420, "Position"=w2419, "Pos limit"=w2416, "Neg limit"=w2415, "Power"=w2417) -> (w2414:T10)
                      n1273 = case shown="\"AxisX\", Default" w2421 {
                        tunnel: w2419 -> [w2428 w2430 w2432 w2434 w2436]
                        tunnel: w2418 -> [_ _ _ _ _]
                        tunnel: w2423 -> [w2427 w2429 w2431 w2433 w2435]
                        frame "AxisX", Default {
                          n1274 = property on="X backward" class="Bool"("DisabledEnum"=w2427) -> ()  [unwired: 2 in, 2 out]
                          n1275 = property on="X forward" class="Bool"("DisabledEnum"=w2427) -> ()  [unwired: 2 in, 2 out]
                          n1276 = property on="X" class="DigNum (strict)"("Val(Sgnl)"=w2428) -> ()  [unwired: 2 in, 2 out]
                        }
                        frame "AxisY" {
                          n1277 = property on="Y left" class="Bool"("DisabledEnum"=w2429) -> ()  [unwired: 2 in, 2 out]
                          n1278 = property on="Y right" class="Bool"("DisabledEnum"=w2429) -> ()  [unwired: 2 in, 2 out]
                          n1279 = property on="Y" class="DigNum (strict)"("Value"=w2430) -> ()  [unwired: 2 in, 2 out]
                        }
                        frame "AxisZ_left" {
                          n1280 = property on="ZLup" class="Bool"("DisabledEnum"=w2431) -> ()  [unwired: 2 in, 2 out]
                          n1281 = property on="ZLdown" class="Bool"("DisabledEnum"=w2431) -> ()  [unwired: 2 in, 2 out]
                          n1282 = property on="ZL" class="DigNum (strict)"("Value"=w2432) -> ()  [unwired: 2 in, 2 out]
                        }
                        frame "AxisZ_middle" {
                          n1283 = property on="ZM" class="DigNum (strict)"("Value"=w2434) -> ()  [unwired: 2 in, 2 out]
                          n1284 = property on="ZMdown" class="Bool"("DisabledEnum"=w2433) -> ()  [unwired: 2 in, 2 out]
                          n1285 = property on="ZMup" class="Bool"("DisabledEnum"=w2433) -> ()  [unwired: 2 in, 2 out]
                        }
                        frame "AxisZ_right" {
                          n1286 = property on="ZRup" class="Bool"("DisabledEnum"=w2435) -> ()  [unwired: 2 in, 2 out]
                          n1287 = property on="ZRdown" class="Bool"("DisabledEnum"=w2435) -> ()  [unwired: 2 in, 2 out]
                          n1288 = property on="ZR" class="DigNum (strict)"("Value"=w2436) -> ()  [unwired: 2 in, 2 out]
                        }
                      }
                    }
                    n1289 = for {
                      tunnel: w2396 -> [w2438] mode=indexing
                      tunnel: [w2437] -> w2400 mode=indexing
                      n1290 = Unbundle By Name(w2438) -> ("Servo variables.Connected"=w2437:bool)
                    }
                    n1291 = And Array Elements(Boolean array=w2400) -> (logical AND=w2399:bool)
                    n1292 = call <vilib>:"Space Constant.vi"() -> ("String"=w2402:string)
                    n1293 = case shown="True" w2399 {
                      frame False {
                      }
                      frame True {
                        n1294 = control-ref of="Servo controls"() -> (w2413:refnum<vi>)
                        n1295 = Build Array(w2413) -> (w2412:refnum<vi>[])
                        n1296 = call "Dis- or en- able controls.vi"("Disabled"=T34."Enabled", "Control referencies"=w2412) -> ()  [unwired: 9 in, 1 out]
                      }
                    }
                    n1297 = local read "Instr status"() -> (w2405:T1)
                    n1298 = Concatenate Strings("Servo" ("string"), w2402, w2408, w2402) -> (w2409:string)
                    n1299 = local read "loggersRef"() -> (w2398:refnum<file>)
                    n1300 = Bundle By Name(cluster=w2405, "Serv"=w2399) -> (w2404:T1)
                    n1301 = call "Add actual date time to string.vi"("String in"=w2409) -> ("String out"=w2397:string)  [unwired: 4 in]
                    n1302 = local write "Instr status"(w2404) -> ()
                    n1303 = call "simple Shift string array.vi"("Element in"=w2397, "Array in"=w2406) -> ("Array out"=w2407:string[])  [unwired: 8 in, 1 out]
                    n1304 = call "Write in logger.vi"("String in"=w2397, "logger refnum"=w2398) -> ()  [unwired: 2 in, 2 out]
                  }
                  frame "Move by" {
                    n1305 = Variant To Data(type=T73 {"Property"="", "Value"=variant, "Name"=enum."AxisX"} ("Array"), Variant=w2458) -> (data=w2450:T73)  [unwired: 1 in, 1 out]
                    n1306 = Unbundle By Name(w2450) -> ("Property"=w2449:string, "Value"=w2448:variant, "Name"=w2447:T11)
                    n1307 = call "Extract axis properties.vi"("Name"=w2447, "All servo status"=w2442) -> ("Servo"=w2441:T10, "Index"=w2443:i32, "Found?"=w2445:bool)  [unwired: 6 in]
                    n1308 = case shown="True" w2445 {
                      tunnel: w2449 -> [w2460 w2469]
                      tunnel: w2448 -> [_ w2468]
                      tunnel: w2447 -> [_ w2467]
                      tunnel: w2441 -> [_ w2466]
                      tunnel: w2443 -> [_ w2465]
                      tunnel: w2442 -> [w2459 w2464]
                      tunnel: [w2460 w2462] -> w2446
                      tunnel: [w2459 w2461] -> w2444
                      frame False {
                      }
                      frame True {
                        n1309 = case shown="\"Power ON\"" w2469 {
                          selector: w2469 -> [w2470 w2473 w2485]
                          tunnel: w2468 -> [_ w2472 w2491]
                          tunnel: w2467 -> [_ w2475 _]
                          tunnel: w2466 -> [w2471 w2478 w2489]
                          tunnel: [w2471 w2477 w2488] -> w2463
                          tunnel: [w2470 w2476 w2487] -> w2462
                          frame "Nothing", Default {
                          }
                          frame "Actual position" {
                            n1310 = Variant To Data(type=0.0, Variant=w2472) -> (data=w2474:dbl)  [unwired: 1 in, 1 out]
                            n1311 = case shown="\"AxisZ_right\"" w2475 {
                              tunnel: w2474 -> [w2480 w2481 w2482 w2483 w2484]
                              frame "AxisX", Default {
                                n1312 = property on="X" class="DigNum (strict)"("Val(Sgnl)"=w2480) -> ()  [unwired: 2 in, 2 out]
                              }
                              frame "AxisY" {
                                n1313 = property on="Y" class="DigNum (strict)"("Value"=w2481) -> ()  [unwired: 2 in, 2 out]
                              }
                              frame "AxisZ_left" {
                                n1314 = property on="ZL" class="DigNum (strict)"("Value"=w2482) -> ()  [unwired: 2 in, 2 out]
                              }
                              frame "AxisZ_middle" {
                                n1315 = property on="ZM" class="DigNum (strict)"("Value"=w2483) -> ()  [unwired: 2 in, 2 out]
                              }
                              frame "AxisZ_right" {
                                n1316 = property on="ZR" class="DigNum (strict)"("Value"=w2484) -> ()  [unwired: 2 in, 2 out]
                              }
                            }
                            n1317 = Bundle By Name(cluster=w2478, "Position"=w2474) -> (w2477:T10)
                            n1318 = Format Into String(initial string=w2473, w2474) -> (resulting string=w2476:string)  [unwired: 2 in, 1 out]
                          }
                          frame "Power ON" {
                            n1319 = Variant To Data(type=FALSE ("Connected"), Variant=w2491) -> (data=w2486:bool)  [unwired: 1 in, 1 out]
                            n1320 = Bundle By Name(cluster=w2489, "Power"=w2486) -> (w2488:T10)
                            n1321 = Format Into String(initial string=w2485, w2486) -> (resulting string=w2487:string)  [unwired: 2 in, 1 out]
                          }
                        }
                        n1322 = Replace Array Subset(array=w2464, new element=w2463, index=w2465) -> (w2461:T10[])
                      }
                    }
                    n1323 = call <vilib>:"Space Constant.vi"() -> ("String"=w2452:string)
                    n1324 = local read "loggersRef"() -> (w2439:refnum<file>)
                    n1325 = Concatenate Strings("Servo" ("string"), w2452, w2456, w2452, w2446) -> (w2457:string)
                    n1326 = call "Add actual date time to string.vi"("String in"=w2457) -> ("String out"=w2440:string)  [unwired: 4 in]
                    n1327 = call "Write in logger.vi"("String in"=w2440, "logger refnum"=w2439) -> ()  [unwired: 2 in, 2 out]
                    n1328 = call "simple Shift string array.vi"("Element in"=w2440, "Array in"=w2454) -> ("Array out"=w2455:string[])  [unwired: 8 in, 1 out]
                  }
                  frame "Update" {
                    n1329 = Variant To Data(type=T73 {"Property"="", "Value"=variant, "Name"=enum."AxisX"} ("Array"), Variant=w2516) -> (data=w2508:T73)  [unwired: 1 in, 1 out]
                    n1330 = Unbundle By Name(w2508) -> ("Property"=w2502:string, "Value"=w2507:variant, "Name"=w2504:T11)
                    n1331 = call "Extract axis properties.vi"("Name"=w2504, "All servo status"=w2495) -> ("Servo"=w2506:T10, "Index"=w2505:i32, "Found?"=w2497:bool)  [unwired: 6 in]
                    n1332 = Format Into String(w2504) -> (resulting string=w2503:string)  [unwired: 3 in, 1 out]
                    n1333 = Bundle By Name(cluster=w2506, "Last update"=w2492) -> (w2493:T10)
                    n1334 = call <vilib>:"Space Constant.vi"() -> ("String"=w2499:string)
                    n1335 = Concatenate Strings(w2502, w2499, w2503, ":" ("string"), w2499) -> (w2501:string)
                    n1336 = case shown="False" w2497 {
                      tunnel: w2507 -> [_ w2533]
                      tunnel: w2493 -> [_ w2532]
                      tunnel: w2495 -> [w2517 w2531]
                      tunnel: w2505 -> [_ w2529]
                      tunnel: w2504 -> [w2523 w2528]
                      tunnel: w2502 -> [w2519 w2527]
                      tunnel: w2501 -> [_ w2526]
                      tunnel: [w2521 w2525] -> w2498
                      tunnel: [w2517 w2524] -> w2494
                      frame False {
                        n1337 = call <vilib>:"Space Constant.vi"() -> ("String"=w2518:string)
                        n1338 = Concatenate Strings(w2519, w2518, "Unknown driver" ("initial string")) -> (w2520:string)
                        n1339 = Format Into String(initial string=w2520, w2523) -> (resulting string=w2521:string)  [unwired: 2 in, 1 out]
                      }
                      frame True {
                        n1340 = case shown="\"Target position\"" w2527 {
                          tunnel: w2533 -> [_ w2543 w2554 w2561]
                          tunnel: w2528 -> [_ w2537 _ _]
                          tunnel: w2532 -> [w2535 w2541 w2552 w2559]
                          tunnel: [w2535 w2540 w2552 w2558] -> w2530
                          tunnel: w2526 -> [w2534 w2539 w2549 w2556]
                          tunnel: [w2534 w2538 w2551 w2557] -> w2525
                          frame "Nothing", Default {
                          }
                          frame "Actual position" {
                            n1341 = Variant To Data(type=0.0, Variant=w2543) -> (data=w2536:dbl)  [unwired: 1 in, 1 out]
                            n1342 = case shown="\"AxisZ_left\"" w2537 {
                              tunnel: w2536 -> [w2544 w2545 w2546 w2547 w2548]
                              frame "AxisX", Default {
                                n1343 = property on="X" class="DigNum (strict)"("Val(Sgnl)"=w2544) -> ()  [unwired: 2 in, 2 out]
                              }
                              frame "AxisY" {
                                n1344 = property on="Y" class="DigNum (strict)"("Value"=w2545) -> ()  [unwired: 2 in, 2 out]
                              }
                              frame "AxisZ_left" {
                                n1345 = property on="ZL" class="DigNum (strict)"("Value"=w2546) -> ()  [unwired: 2 in, 2 out]
                              }
                              frame "AxisZ_middle" {
                                n1346 = property on="ZM" class="DigNum (strict)"("Value"=w2547) -> ()  [unwired: 2 in, 2 out]
                              }
                              frame "AxisZ_right" {
                                n1347 = property on="ZR" class="DigNum (strict)"("Value"=w2548) -> ()  [unwired: 2 in, 2 out]
                              }
                            }
                            n1348 = Bundle By Name(cluster=w2541, "Position"=w2536) -> (w2540:T10)
                            n1349 = Format Into String(initial string=w2539, w2536) -> (resulting string=w2538:string)  [unwired: 2 in, 1 out]
                          }
                          frame "Target position" {
                            n1350 = Variant To Data(type=0.0, Variant=w2554) -> (data=w2550:dbl)  [unwired: 1 in, 1 out]
                            n1351 = Format Into String(initial string=w2549, w2550) -> (resulting string=w2551:string)  [unwired: 2 in, 1 out]
                          }
                          frame "Power ON" {
                            n1352 = Variant To Data(type=FALSE ("Connected"), Variant=w2561) -> (data=w2555:bool)  [unwired: 1 in, 1 out]
                            n1353 = Bundle By Name(cluster=w2559, "Power"=w2555) -> (w2558:T10)
                            n1354 = Format Into String(initial string=w2556, w2555) -> (resulting string=w2557:string)  [unwired: 2 in, 1 out]
                          }
                        }
                        n1355 = Replace Array Subset(array=w2531, new element=w2530, index=w2529) -> (w2524:T10[])
                      }
                    }
                    n1356 = call <vilib>:"Space Constant.vi"() -> ("String"=w2496:string)
                    n1357 = Concatenate Strings("Servo" ("string"), w2496, w2509, w2496, w2496, w2496, w2498, w2496) -> (w2510:string)
                    n1358 = call "Add actual date time to string.vi"("String in"=w2510) -> ("String out"=w2514:string)  [unwired: 4 in]
                    n1359 = call "simple Shift string array.vi"("Element in"=w2514, "Array in"=w2512) -> ("Array out"=w2513:string[])  [unwired: 8 in, 1 out]
                  }
                  frame "End" {
                    w2574 = nan
                    n1360 = local read "Instr status"() -> (w2600:T1)
                    n1361 = control-ref of="Servo controls"() -> (w2598:refnum<vi>)
                    n1362 = Bundle By Name(cluster=w2600, "Serv"=FALSE ("PSU")) -> (w2601:T1)
                    n1363 = local write "Instr status"(w2601) -> ()
                    n1364 = Array Size(array=w2563) -> (size(s)=w2593:i32)
                    n1365 = property class="Clust"(reference=w2598, "DisabledEnum"=T34."Disabled and Grayed Out" ("Disabled")) -> ()  [unwired: 1 in, 2 out]
                    n1366 = call "Extract axis properties.vi"("Name"=Axis_names."AxisX", "All servo status"=w2563) -> ("Servo"=w2591:T10, "Found?"=w2586:bool)  [unwired: 6 in, 1 out]
                    n1367 = call "Extract axis properties.vi"("Name"=Axis_names."AxisY", "All servo status"=w2563) -> ("Servo"=w2590:T10, "Found?"=w2584:bool)  [unwired: 6 in, 1 out]
                    n1368 = call "Extract axis properties.vi"("Name"=Axis_names."AxisZ_middle", "All servo status"=w2563) -> ("Servo"=w2589:T10, "Found?"=w2583:bool)  [unwired: 6 in, 1 out]
                    n1369 = call "Extract axis properties.vi"("Name"=Axis_names."AxisZ_left", "All servo status"=w2563) -> ("Servo"=w2588:T10, "Found?"=w2582:bool)  [unwired: 6 in, 1 out]
                    n1370 = call "Extract axis properties.vi"("Name"=Axis_names."AxisZ_right", "All servo status"=w2563) -> ("Servo"=w2587:T10, "Found?"=w2581:bool)  [unwired: 6 in, 1 out]
                    n1371 = Delete From Array(array=w2563, length=w2593) -> (array with subset deleted=w2592:T10[])  [unwired: 1 in, 1 out]
                    n1372 = Unbundle By Name(w2587) -> ("Position"=w2579:dbl)
                    n1373 = Unbundle By Name(w2590) -> ("Position"=w2577:dbl)
                    n1374 = Unbundle By Name(w2589) -> ("Position"=w2578:dbl)
                    n1375 = Unbundle By Name(w2588) -> ("Position"=w2580:dbl)
                    n1376 = Unbundle By Name(w2591) -> ("Position"=w2585:dbl)
                    n1377 = Select(t=w2585, s=w2586, f=w2574) -> (s? t:f=w2564:dbl)
                    n1378 = Select(t=w2577, s=w2584, f=w2574) -> (s? t:f=w2568:dbl)
                    n1379 = Select(t=w2578, s=w2583, f=w2574) -> (s? t:f=w2566:dbl)
                    n1380 = Select(t=w2580, s=w2582, f=w2574) -> (s? t:f=w2567:dbl)
                    n1381 = Select(t=w2579, s=w2581, f=w2574) -> (s? t:f=w2565:dbl)
                    n1382 = Format Into String(format string="\\nX: %f\\tY: %f\\tZM: %f\\tZL: %f\\tZR: %f", initial string="Servo ended " ("Element in"), w2564, w2568, w2566, w2567, w2565) -> (resulting string=w2562:string)  [unwired: 1 in, 1 out]
                    n1383 = local read "loggersRef"() -> (w2594:refnum<file>)
                    n1384 = call "simple Shift string array.vi"("Element in"=w2562, "Array in"=w2595) -> ("Array out"=w2596:string[])  [unwired: 8 in, 1 out]
                    n1385 = call "Write in logger.vi"("String in"=w2562, "logger refnum"=w2594) -> ()  [unwired: 2 in, 2 out]
                  }
                  frame "Disconnect" {
                    w2609 = nan
                    n1386 = local read "Instr status"() -> (w2640:T1)
                    n1387 = control-ref of="Servo controls"() -> (w2638:refnum<vi>)
                    n1388 = Bundle By Name(cluster=w2640, "Serv"=FALSE ("PSU")) -> (w2641:T1)
                    n1389 = Array Size(array=w2628) -> (size(s)=w2632:i32)
                    n1390 = local write "Instr status"(w2641) -> ()
                    n1391 = Delete From Array(array=w2628, length=w2632) -> (array with subset deleted=w2631:T10[])  [unwired: 1 in, 1 out]
                    n1392 = call "Extract axis properties.vi"("Name"=Axis_names."AxisX", "All servo status"=w2628) -> ("Servo"=w2622:T10, "Found?"=w2617:bool)  [unwired: 6 in, 1 out]
                    n1393 = call "Extract axis properties.vi"("Name"=Axis_names."AxisY", "All servo status"=w2628) -> ("Servo"=w2621:T10, "Found?"=w2615:bool)  [unwired: 6 in, 1 out]
                    n1394 = call "Extract axis properties.vi"("Name"=Axis_names."AxisZ_middle", "All servo status"=w2628) -> ("Servo"=w2620:T10, "Found?"=w2614:bool)  [unwired: 6 in, 1 out]
                    n1395 = call "Extract axis properties.vi"("Name"=Axis_names."AxisZ_left", "All servo status"=w2628) -> ("Servo"=w2619:T10, "Found?"=w2613:bool)  [unwired: 6 in, 1 out]
                    n1396 = call "Extract axis properties.vi"("Name"=Axis_names."AxisZ_right", "All servo status"=w2628) -> ("Servo"=w2618:T10, "Found?"=w2612:bool)  [unwired: 6 in, 1 out]
                    n1397 = property class="Clust"(reference=w2638, "DisabledEnum"=T34."Disabled and Grayed Out" ("Disabled")) -> ()  [unwired: 1 in, 2 out]
                    n1398 = Unbundle By Name(w2618) -> ("Position"=w2610:dbl)
                    n1399 = Unbundle By Name(w2621) -> ("Position"=w2607:dbl)
                    n1400 = Unbundle By Name(w2620) -> ("Position"=w2608:dbl)
                    n1401 = Unbundle By Name(w2619) -> ("Position"=w2611:dbl)
                    n1402 = Unbundle By Name(w2622) -> ("Position"=w2616:dbl)
                    n1403 = Select(t=w2616, s=w2617, f=w2609) -> (s? t:f=w2606:dbl)
                    n1404 = Select(t=w2607, s=w2615, f=w2609) -> (s? t:f=w2605:dbl)
                    n1405 = Select(t=w2608, s=w2614, f=w2609) -> (s? t:f=w2604:dbl)
                    n1406 = Select(t=w2611, s=w2613, f=w2609) -> (s? t:f=w2603:dbl)
                    n1407 = Select(t=w2610, s=w2612, f=w2609) -> (s? t:f=w2602:dbl)
                    n1408 = Format Into String(format string="\\nX: %f\\tY: %f\\tZM: %f\\tZL: %f\\tZR: %f", initial string="Servo disconnected " ("Element in"), w2606, w2605, w2604, w2603, w2602) -> (resulting string=w2630:string)  [unwired: 1 in, 1 out]
                    n1409 = local read "loggersRef"() -> (w2634:refnum<file>)
                    n1410 = call "simple Shift string array.vi"("Element in"=w2630, "Array in"=w2635) -> ("Array out"=w2636:string[])  [unwired: 8 in, 1 out]
                    n1411 = call "Write in logger.vi"("String in"=w2630, "logger refnum"=w2634) -> ()  [unwired: 2 in, 2 out]
                  }
                  frame "Error", Default {
                    n1412 = Variant To Data(type=errorcluster {"status"=FALSE, "code"=0, "source"=""} ("error constant"), Variant=w2649) -> (data=w2647:errorcluster)  [unwired: 1 in, 1 out]
                    n1413 = Unbundle By Name(w2647) -> ("source"=w2646:string)
                    n1414 = call <vilib>:"Space Constant.vi"() -> ("String"=w2652:string)
                    n1415 = Concatenate Strings("Servo: " ("string"), w2651, w2652, w2646) -> (w2650:string)
                    n1416 = local read "loggersRef"() -> (w2645:refnum<file>)
                    n1417 = call "Add actual date time to string.vi"("String in"=w2650) -> ("String out"=w2644:string)  [unwired: 4 in]
                    n1418 = call "simple Shift string array.vi"("Element in"=w2644, "Array in"=w2654) -> ("Array out"=w2653:string[])  [unwired: 8 in, 1 out]
                    n1419 = call "Write in logger.vi"("String in"=w2644, "logger refnum"=w2645) -> ()  [unwired: 2 in, 2 out]
                  }
                }
                n1420 = Bundle By Name(cluster=w2386, "Servo"=w2383) -> (w2385:T8)
              }
              frame "Rotator" {
                n1421 = Format Into String(w2663) -> (resulting string=w2661:string)  [unwired: 3 in, 1 out]
                n1422 = Unbundle By Name(w2660) -> ("Magnet.Field [T]"=w2655:dbl, "Rotator"=w2659:T89)
                n1423 = case shown="\"Initialize\"" w2667 {
                  selector: w2667 -> [_ _ _ w2731 _ w2779 _ _]
                  tunnel: w2666 -> [_ w2690 w2727 w2752 w2773 w2786 w2797 w2812]
                  tunnel: w2665 -> [w2669 w2689 w2725 w2729 w2766 w2784 w2801 w2815]
                  tunnel: [w2669 w2688 w2725 w2728 w2765 w2783 w2800 w2814] -> w2664
                  tunnel: w2661 -> [_ w2684 _ w2733 _ w2780 _ _]
                  tunnel: w2659 -> [w2668 w2685 w2723 w2749 w2771 w2782 w2802 w2817]
                  tunnel: [w2668 w2682 w2722 w2748 w2771 w2782 w2795 w2816] -> w2657
                  tunnel: w2656 -> [_ w2681 w2721 w2747 _ _ w2793 _]
                  tunnel: w2655 -> [_ _ w2710 w2737 _ _ _ _]
                  frame "Ignore", Default {
                  }
                  frame "Initialize" {
                    n1424 = Variant To Data(type=T74 {"Controller info"={"deviceNumber"=0, "DeviceType"=0, "ID"=0, "Serial"="", "Address"="", "connected"=FALSE}, "Handle"=0, "FW-Version"=0, "Features"=0, "ActuatorType"=0, "ActuatorName"="", "Axis info"={"Axis status"={"connected"=FALSE, "enabled"=FALSE, "moving"=FALSE, "target"=FALSE, "EotFwd"=FALSE, "EotBwd"=FALSE, "error"=FALSE}, "Position [°]"=0.0, "Freque [Hz]"=0.0, "Voltage [V]"=0.0}, "Capacitance[uF]"=0.0, "Path to DLL"=path ""} ("Rotator"), Variant=w2690) -> (data=w2687:T74)  [unwired: 1 in, 1 out]
                    n1425 = Unbundle By Name(w2687) -> ("Controller info.DeviceType"=w2676:i32, "Controller info.connected"=w2686:bool, "Axis info.Axis status.connected"=w2680:bool, "Axis info.Axis status.moving"=w2679:bool, "Axis info.Axis status.target"=w2677:bool, "Capacitance[uF]"=w2678:dbl, "Axis info.Position [°]"=w2673:dbl, "Axis info.Freque [Hz]"=w2671:dbl, "Axis info.Voltage [V]"=w2672:dbl, "ActuatorType"=w2675:u16)
                    n1426 = property on="Rot" class="Bool (strict)"("Value"=w2686) -> ()  [unwired: 2 in, 2 out]
                    n1427 = case shown="True" w2686 {
                      tunnel: w2689 -> [w2692 w2702]
                      tunnel: [w2692 w2701] -> w2688
                      tunnel: w2684 -> [_ w2697]
                      tunnel: w2676 -> [_ w2698]
                      tunnel: ["None" w2693] -> _
                      frame False {
                      }
                      frame True {
                        n1428 = case shown="0, Default" w2698 {
                          tunnel: ["ANC350res" "ANC350num" "ANC350fps" "Unknown"] -> w2693
                          frame 0, Default {
                          }
                          frame 1 {
                          }
                          frame 2 {
                          }
                          frame 3 {
                          }
                        }
                        n1429 = local read "loggersRef"() -> (w2699:refnum<file>)
                        n1430 = call <vilib>:"Space Constant.vi"() -> ("String"=w2696:string)
                        n1431 = Concatenate Strings(w2697, w2696, "Rotator" ("string"), w2696, w2693) -> (w2700:string)
                        n1432 = call "Add actual date time to string.vi"("String in"=w2700) -> ("String out"=w2694:string)  [unwired: 4 in]
                        n1433 = call "simple Shift string array.vi"("Element in"=w2694, "Array in"=w2702) -> ("Array out"=w2701:string[])  [unwired: 8 in, 1 out]
                        n1434 = call "Write in logger.vi"("String in"=w2694, "logger refnum"=w2699) -> ()  [unwired: 2 in, 2 out]
                      }
                    }
                    n1435 = local read "Rotator controls"() -> (w2674:T15)
                    n1436 = Bundle By Name(cluster=w2674, "Motion properties.Frequency [Hz]"=w2671, "Motion properties.Amplitude [V]"=w2672, "Actual angle[°]"=w2673) -> (w2670:T15)
                    n1437 = Bundle By Name(cluster=w2685, "Name"=w2676, "Last update"=w2681, "Actuator"=w2675, "Connected"=w2680, "Moving"=w2679, "Target"=w2677, "Cap [nF]"=w2678, "Position [°]"=w2673) -> (w2682:T89)
                    n1438 = local write "Rotator controls"(w2670) -> ()
                  }
                  frame "Update" {
                    n1439 = Variant To Data(type=T75 {"Axis status"={"connected"=FALSE, "enabled"=FALSE, "moving"=FALSE, "target"=FALSE, "EotFwd"=FALSE, "EotBwd"=FALSE, "error"=FALSE}, "Position [°]"=0.0, "Freque [Hz]"=0.0, "Voltage [V]"=0.0} ("Axis status"), Variant=w2727) -> (data=w2724:T75)  [unwired: 1 in, 1 out]
                    n1440 = Unbundle By Name(w2724) -> ("Axis status.connected"=w2715:bool, "Axis status.moving"=w2714:bool, "Axis status.target"=w2713:bool, "Position [°]"=w2717:dbl, "Voltage [V]"=w2718:dbl, "Freque [Hz]"=w2716:dbl, "Axis status.EotFwd"=w2709:bool, "Axis status.EotBwd"=w2708:bool, "Axis status.error"=w2707:bool)
                    n1441 = Less Or Equal?(x=w2710, y=8.0) -> (x <= y?=w2712:bool)
                    n1442 = local read "Rotator controls"() -> (w2720:T15)
                    n1443 = Bundle By Name(cluster=w2720, "Motion properties.Amplitude [V]"=w2718, "Motion properties.Frequency [Hz]"=w2716, "Actual angle[°]"=w2717, "Set position.Safe to move?"=w2712, "EoF"=w2709, "EoB"=w2708, "Error"=w2707) -> (w2719:T15)
                    n1444 = Bundle By Name(cluster=w2723, "Last update"=w2721, "Position [°]"=w2717, "Connected"=w2715, "Moving"=w2714, "Target"=w2713) -> (w2722:T89)
                    n1445 = local write "Rotator controls"(w2719) -> ()
                  }
                  frame "Stop movement" {
                    n1446 = Variant To Data(type=T75 {"Axis status"={"connected"=FALSE, "enabled"=FALSE, "moving"=FALSE, "target"=FALSE, "EotFwd"=FALSE, "EotBwd"=FALSE, "error"=FALSE}, "Position [°]"=0.0, "Freque [Hz]"=0.0, "Voltage [V]"=0.0} ("Axis status"), Variant=w2752) -> (data=w2750:T75)  [unwired: 1 in, 1 out]
                    n1447 = Unbundle By Name(w2750) -> ("Axis status.connected"=w2742:bool, "Axis status.moving"=w2741:bool, "Axis status.target"=w2740:bool, "Position [°]"=w2732:dbl, "Voltage [V]"=w2744:dbl, "Freque [Hz]"=w2743:dbl)
                    n1448 = Format Into String(format string=": %s at %.1f°", initial string=w2733, w2731, w2732) -> (resulting string=w2735:string)  [unwired: 1 in, 1 out]
                    n1449 = local read "loggersRef"() -> (w2736:refnum<file>)
                    n1450 = call "Add actual date time to string.vi"("String in"=w2735) -> ("String out"=w2730:string)  [unwired: 4 in]
                    n1451 = Less Or Equal?(x=w2737, y=8.0) -> (x <= y?=w2739:bool)
                    n1452 = call "Write in logger.vi"("String in"=w2730, "logger refnum"=w2736) -> ()  [unwired: 2 in, 2 out]
                    n1453 = local read "Rotator controls"() -> (w2746:T15)
                    n1454 = Bundle By Name(cluster=w2746, "Motion properties.Amplitude [V]"=w2744, "Motion properties.Frequency [Hz]"=w2743, "Actual angle[°]"=w2732, "Set position.Safe to move?"=w2739) -> (w2745:T15)
                    n1455 = Bundle By Name(cluster=w2749, "Last update"=w2747, "Position [°]"=w2732, "Connected"=w2742, "Moving"=w2741, "Target"=w2740) -> (w2748:T89)
                    n1456 = local write "Rotator controls"(w2745) -> ()
                    n1457 = call "simple Shift string array.vi"("Element in"=w2730, "Array in"=w2729) -> ("Array out"=w2728:string[])  [unwired: 8 in, 1 out]
                  }
                  frame "Set parameters" {
                    n1458 = Variant To Data(type=T16 {"Frequency [Hz]"=1000.0, "Precision [m°]"=10.0, "DC voltage [V]"=1.0, "Amplitude [V]"=6.0} ("Motion parameters"), Variant=w2773) -> (data=w2769:T16)  [unwired: 1 in, 1 out]
                    n1459 = local read "Rotator controls"() -> (w2770:T15)
                    n1460 = Bundle By Name(cluster=w2770, "Motion properties"=w2769) -> (w2762:T15)
                    n1461 = Unbundle By Name(w2762) -> ("Motion properties.Frequency [Hz]"=w2760:dbl, "Motion properties.Precision [m°]"=w2759:dbl, "Motion properties.DC voltage [V]"=w2758:dbl, "Motion properties.Amplitude [V]"=w2757:dbl)
                    n1462 = local write "Rotator controls"(w2762) -> ()
                    n1463 = Format Into String(format string="\\n%s %.1f,%s %.1f,%s %.1f,%s %.1f", initial string="Rotator: new parameters set" ("String in"), "Freq [Hz]" ("input 1"), w2760, "Range [m°]" ("input 1"), w2759, "DC voltage [V]" ("input 1"), w2758, "Amplitude [Hz]" ("input 1"), w2757) -> (resulting string=w2761:string)  [unwired: 1 in, 1 out]
                    n1464 = local read "loggersRef"() -> (w2768:refnum<file>)
                    n1465 = call "Add actual date time to string.vi"("String in"=w2761) -> ("String out"=w2767:string)  [unwired: 4 in]
                    n1466 = call "Write in logger.vi"("String in"=w2767, "logger refnum"=w2768) -> ()  [unwired: 2 in, 2 out]
                    n1467 = call "simple Shift string array.vi"("Element in"=w2767, "Array in"=w2766) -> ("Array out"=w2765:string[])  [unwired: 8 in, 1 out]
                  }
                  frame "Set position" {
                    n1468 = Variant To Data(type=T17 {"Relative?"=FALSE, "Position [°]"=0.0, "Safe to move?"=FALSE} ("Set position"), Variant=w2786) -> (data=w2775:T17)  [unwired: 1 in, 1 out]
                    n1469 = Unbundle By Name(w2775) -> ("Position [°]"=w2774:dbl)
                    n1470 = Format Into String(format string=": %s %.1f°", initial string=w2780, w2779, w2774) -> (resulting string=w2778:string)  [unwired: 1 in, 1 out]
                    n1471 = local read "Rotator controls"() -> (w2777:T15)
                    n1472 = Bundle By Name(cluster=w2777, "Set position"=w2775) -> (w2776:T15)
                    n1473 = local write "Rotator controls"(w2776) -> ()
                    n1474 = call "simple Shift string array.vi"("Element in"=w2778, "Array in"=w2784) -> ("Array out"=w2783:string[])  [unwired: 8 in, 1 out]
                  }
                  frame "End" {
                    n1475 = Variant To Data(type=T74 {"Controller info"={"deviceNumber"=0, "DeviceType"=0, "ID"=0, "Serial"="", "Address"="", "connected"=FALSE}, "Handle"=0, "FW-Version"=0, "Features"=0, "ActuatorType"=0, "ActuatorName"="", "Axis info"={"Axis status"={"connected"=FALSE, "enabled"=FALSE, "moving"=FALSE, "target"=FALSE, "EotFwd"=FALSE, "EotBwd"=FALSE, "error"=FALSE}, "Position [°]"=0.0, "Freque [Hz]"=0.0, "Voltage [V]"=0.0}, "Capacitance[uF]"=0.0, "Path to DLL"=path ""} ("Rotator"), Variant=w2797) -> (data=w2796:T74)  [unwired: 1 in, 1 out]
                    n1476 = Unbundle By Name(w2796) -> ("Controller info.DeviceType"=w2794:i32, "ActuatorType"=w2791:u16, "Controller info.connected"=w2792:bool, "Axis info.Axis status.moving"=w2790:bool, "Axis info.Axis status.target"=w2789:bool, "Capacitance[uF]"=w2788:dbl, "Axis info.Position [°]"=w2787:dbl)
                    n1477 = Bundle By Name(cluster=w2802, "Name"=w2794, "Last update"=w2793, "Actuator"=w2791, "Connected"=w2792, "Moving"=w2790, "Target"=w2789, "Cap [nF]"=w2788, "Position [°]"=w2787) -> (w2795:T89)
                    n1478 = call "Add actual date time to string.vi"("String in"="Rotator module ended") -> ("String out"=w2799:string)  [unwired: 4 in]
                    n1479 = local read "loggersRef"() -> (w2804:refnum<file>)
                    n1480 = local read "Instr status"() -> (w2806:T1)
                    n1481 = Bundle By Name(cluster=w2806, "Rot"=FALSE ("PSU")) -> (w2807:T1)
                    n1482 = call "Write in logger.vi"("String in"=w2799, "logger refnum"=w2804) -> ()  [unwired: 2 in, 2 out]
                    n1483 = local write "Instr status"(w2807) -> ()
                    n1484 = call "simple Shift string array.vi"("Element in"=w2799, "Array in"=w2801) -> ("Array out"=w2800:string[])  [unwired: 8 in, 1 out]
                  }
                  frame "Disconnect" {
                    n1485 = Variant To Data(type=T74 {"Controller info"={"deviceNumber"=0, "DeviceType"=0, "ID"=0, "Serial"="", "Address"="", "connected"=FALSE}, "Handle"=0, "FW-Version"=0, "Features"=0, "ActuatorType"=0, "ActuatorName"="", "Axis info"={"Axis status"={"connected"=FALSE, "enabled"=FALSE, "moving"=FALSE, "target"=FALSE, "EotFwd"=FALSE, "EotBwd"=FALSE, "error"=FALSE}, "Position [°]"=0.0, "Freque [Hz]"=0.0, "Voltage [V]"=0.0}, "Capacitance[uF]"=0.0, "Path to DLL"=path ""} ("Rotator"), Variant=w2812) -> (data=w2810:T74)  [unwired: 1 in, 1 out]
                    n1486 = Unbundle By Name(w2810) -> ("Axis info.Axis status.connected"=w2809:bool, "Axis info.Position [°]"=w2808:dbl)
                    n1487 = Bundle By Name(cluster=w2817, "Connected"=w2809, "Position [°]"=w2808) -> (w2816:T89)
                    n1488 = local read "Instr status"() -> (w2821:T1)
                    n1489 = local read "loggersRef"() -> (w2819:refnum<file>)
                    n1490 = call "Add actual date time to string.vi"("String in"="Rotator module disconnected") -> ("String out"=w2813:string)  [unwired: 4 in]
                    n1491 = Bundle By Name(cluster=w2821, "Rot"=FALSE ("PSU")) -> (w2822:T1)
                    n1492 = call "Write in logger.vi"("String in"=w2813, "logger refnum"=w2819) -> ()  [unwired: 2 in, 2 out]
                    n1493 = local write "Instr status"(w2822) -> ()
                    n1494 = call "simple Shift string array.vi"("Element in"=w2813, "Array in"=w2815) -> ("Array out"=w2814:string[])  [unwired: 8 in, 1 out]
                  }
                }
                n1495 = Bundle By Name(cluster=w2660, "Rotator"=w2657) -> (w2658:T8)
              }
              frame "Emty", Default {
                n1496 = Format Into String(w2828) -> (resulting string=w2827:string)  [unwired: 3 in, 1 out]
                n1497 = call <vilib>:"Space Constant.vi"() -> ("String"=w2829:string)
                n1498 = Concatenate Strings(w2827, w2829, w2826) -> (w2825:string)
                n1499 = call "simple Shift string array.vi"("Element in"=w2825, "Array in"=w2831) -> ("Array out"=w2830:string[])  [unwired: 8 in, 1 out]
              }
            }
          }
          frame True {
          }
        }
        "Instr info" <- w1410
        n1500 = case shown="False" w1417 {
          selector: w1417 -> [w1436 w1437]
          tunnel: [w1434 TopStates."Check message" ("State")] -> w1415
          tunnel: w1408 -> [w1430 _]
          frame False {
            n1501 = local write "Busy"(w1436) -> ()
            n1502 = Equal?(x=w1430, y=experiment_state."Setup" ("Value")) -> (x = y?=w1432:bool)
            n1503 = Select(t=TopStates."Wait for Event" ("State"), s=w1432, f=TopStates."Check measurement") -> (s? t:f=w1434:T30)
          }
          frame True {
            "Busy" <- w1437
          }
        }
      }
      frame "Check measurement" {
        n1504 = Unbundle By Name(w2835) -> ("Experiment state"=w2837:T26)  [unwired: 1 out]
        n1505 = case shown="\"Preparation\"" w2837 {
          tunnel: w2843 -> [_ w2871 w2893 _ _ _]
          tunnel: w2839 -> [w2845 w2860 w2906 w2964 w2973 w3049]
          tunnel: w2842 -> [w2847 w2877 w2911 w2968 w2979 w3068]
          tunnel: [w2847 w2875 w2910 w2968 w2979 w3067] -> w2841
          tunnel: [w2846 w2874 w2908 w2967 w2975 w3065] -> w2840
          tunnel: w2835 -> [w2846 w2872 w2909 w2967 w2976 w3066]
          tunnel: [w2845 w2860 w2905 w2964 w2973 w3062] -> w2838
          tunnel: w2836 -> [_ w2852 w2904 _ w2971 _]
          tunnel: w2835 -> [_ _ _ _ w2970 _]
          frame "Setup", Default {
            # "here can be implemented check of input parameters before measurement"
          }
          frame "Preparation" {
            n1506 = local read "THz control"() -> (w2851:T22)
            n1507 = call "Add point to array for XY graph.vi"("Reset?(F)"=TRUE ("Reset?")) -> ()  [unwired: 6 in, 1 out]
            n1508 = Unbundle By Name(w2860) -> ("Mod_A [G]"=w2853:dbl)
            n1509 = call "Prepare measurement.vi"("Instr info"=w2852, "VID control"=w2851, "Script cluster"=w2860, "Referencies in"=w2871) -> ("error out"=w2865:errorcluster)  [unwired: 7 in]
            n1510 = local write "VTI tmp reached"(FALSE ("VTI tmp reached")) -> ()
            n1511 = local read "Acquisition controls"() -> (w2855:T21)
            n1512 = call "Add actual date time to string.vi"("String in"="Preparing for measurement") -> ("String out"=w2878:string)  [unwired: 4 in]
            n1513 = call "simple Shift string array.vi"("Element in"=w2878, "Array in"=w2877) -> ("Array out"=w2875:string[])  [unwired: 8 in, 1 out]
            n1514 = Unbundle By Name(w2855) -> ("Sample holder"=w2856:T20)
            n1515 = Bundle By Name(cluster=w2855, "Desired [G]"=w2853, "Auto-modulation"=TRUE) -> (w2854:T21)
            n1516 = property on="Script Array" class="Arr (strict)"() -> ("Selection Start []"=w2859:u32[])  [unwired: 2 in, 2 out]
            n1517 = local read "Main data folder"() -> (w2857:path)
            n1518 = local write "Acquisition controls"(w2854) -> ()
            n1519 = Index Array(array=w2859) -> (element=w2858:u32)  [unwired: 1 in]
            n1520 = Select(t=experiment_state."Setup", s=w2865, f=experiment_state."Stabilization" ("Value")) -> (s? t:f=w2866:T26)
            n1521 = call "Create measurement file.vi"("Global comment"="Global comment", "Subfolder"=w2857, "Operator"="Operator", "Row"=w2860, "Sample name"="Sample name", "Sample holder"=w2856, "Line index"=w2858, "Create folder with date"="Create folder with date") -> ("Data file ref out"=→"meas results":refnum<file>)  [unwired: 5 in, 2 out]
            n1522 = Bundle By Name(cluster=w2872, "Experiment state"=w2866) -> (w2874:T25)
            "VTI tmp reached" <- FALSE ("VTI tmp reached")
            "Tmp reched time" <- u32 0 ("Tmp reched time")
          }
          frame "Stabilization" {
            n1523 = Unbundle By Name(w2893) -> ("Angle_C"=w2886:refnum<queue>)
            n1524 = Unbundle By Name(w2904) -> ("Rotator.Connected"=w2891:bool, "Rotator.Target"=w2897:bool, "Magnet.Field [T]"=w2889:dbl, "VTI.VTI [K]"=w2903:dbl, "Rotator.Position [°]"=w2895:dbl)
            n1525 = Unbundle By Name(w2906) -> ("Angle [°]"=w2885:dbl, "Start"=w2900:dbl, "Tmp [K]"=w2880:dbl, "Wait [min]"=w2902:dbl)
            n1526 = Not(x=w2891) -> (.not. x?=w2896:bool)
            n1527 = Less Than 0?(x=w2885) -> (x < 0?=w2883:bool)
            n1528 = local read "VTI tmp reached"() -> (w2917:bool)
            n1529 = call "Is equal in tolerance.vi"("Absolut tolerance"=0.5, "Reference value"=w2885, "Input value"=w2895) -> ("Is in range"=w2887:bool)  [unwired: 1 in]
            n1530 = Compound Arithmetic op=OR(w2883, w2896, w2897) -> (w2898:bool)
            n1531 = Less Or Equal To 0?(x=w2880) -> (x <= 0?=w2879:bool)
            n1532 = call "Is equal in tolerance.vi"("Absolut tolerance"=0.5, "Reference value"=w2880, "Input value"=w2903) -> ("Is in range"=w2914:bool)  [unwired: 1 in]
            n1533 = Not(x=w2917) -> (.not. x?=w2915:bool)
            n1534 = Less Or Equal?(x=w2889, y=8.0) -> (x <= y?=w2888:bool)
            n1535 = Or(x=w2879, y=w2914) -> (x .or. y?=w2881:bool)
            n1536 = Or(x=w2887, y=w2883) -> (x .or. y?=w2884:bool)
            n1537 = And(x=w2891, y=w2888) -> (x .and. y?=w2892:bool)
            n1538 = And(x=w2881, y=w2915) -> (x .and. y?=w2916:bool)
            n1539 = case shown="True" w2892 {
              tunnel: w2884 -> [_ w2921]
              tunnel: w2886 -> [_ w2920]
              tunnel: w2885 -> [_ w2919]
              frame False {
              }
              frame True {
                n1540 = case shown="False" w2921 {
                  tunnel: w2920 -> [w2923 _]
                  tunnel: w2919 -> [w2922 _]
                  frame False {
                    n1541 = Bundle By Name(cluster=T17 {"Relative?"=FALSE, "Position [°]"=0.0, "Safe to move?"=TRUE} ("Set position"), "Position [°]"=w2922) -> (w2926:T17)
                    n1542 = Bundle By Name(cluster=T41 {"Command"=enum."Set position", "Data"=variant} ("MSG to rotator"), "Data"=w2926) -> (w2927:T41)
                    n1543 = call "Put in mailbox.vi"("Message"=w2927, "Queue in"=w2923) -> ()  [unwired: 7 in, 3 out]
                  }
                  frame True {
                  }
                }
              }
            }
            n1544 = case shown="False" w2916 {
              tunnel: w2881 -> [w2946 _]
              tunnel: w2902 -> [w2945 w2958]
              tunnel: [w2944 FALSE] -> w2913
              tunnel: [w2943 w2958] -> w2901
              frame False {
                n1545 = case shown="True" w2946 {
                  selector: w2946 -> [w2948 _]
                  tunnel: w2945 -> [w2947 w2953]
                  tunnel: [w2948 w2951] -> w2944
                  tunnel: [w2947 w2949] -> w2943
                  frame False {
                    n1546 = local write "VTI tmp reached"(w2948) -> ()
                  }
                  frame True {
                    n1547 = local read "Tmp reched time"() -> (w2957:dbl)
                    n1548 = Get Date/Time In Seconds() -> (seconds since 1Jan1904=w2950:timestamp)
                    n1549 = To Double Precision Float(number=w2950) -> (double precision float=w2955:dbl)
                    n1550 = Multiply(x=w2953, y=60.0) -> (x*y=w2952:dbl)
                    n1551 = Subtract(x=w2955, y=w2957) -> (x-y=w2954:dbl)
                    n1552 = Subtract(x=w2952, y=w2954) -> (x-y=w2949:dbl)
                    n1553 = Less Or Equal To 0?(x=w2949) -> (x <= 0?=w2951:bool)
                  }
                }
              }
              frame True {
                n1554 = Get Date/Time In Seconds() -> (seconds since 1Jan1904=w2960:timestamp)
                n1555 = To Double Precision Float(number=w2960) -> (double precision float=w2959:dbl)
                n1556 = local write "VTI tmp reached"(TRUE ("VTI tmp reached")) -> ()
                n1557 = local write "Tmp reched time"(w2959) -> ()
              }
            }
            n1558 = call "Is equal in tolerance.vi"("Absolut tolerance"=0.001, "Reference value"=w2900, "Input value"=w2889) -> ("Is in range"=w2899:bool)  [unwired: 1 in]
            n1559 = Compound Arithmetic op=AND(w2898, w2899, w2913) -> (w2912:bool)
            n1560 = case shown="True" w2912 {
              tunnel: w2906 -> [w2928 w2932]
              tunnel: w2893 -> [_ w2937]
              tunnel: w2911 -> [w2930 w2940]
              tunnel: [w2930 w2939] -> w2910
              tunnel: [experiment_state."Stabilization" ("Value") w2935] -> w2907
              tunnel: [w2928 w2932] -> w2905
              frame False {
              }
              frame True {
                n1561 = Unbundle By Name(w2932) -> ("Auto-mod"=w2931:bool)
                n1562 = call "Start measurement.vi"("Actual measurement"=w2932, "Referencies in"=w2937) -> ("error out"=w2936:errorcluster)  [unwired: 9 in]
                n1563 = call "Add actual date time to string.vi"("String in"="Starting measurement") -> ("String out"=w2941:string)  [unwired: 4 in]
                n1564 = call "simple Shift string array.vi"("Element in"=w2941, "Array in"=w2940) -> ("Array out"=w2939:string[])  [unwired: 8 in, 1 out]
                n1565 = Select(t=experiment_state."Save" ("Value"), s=w2936, f=experiment_state."Begin" ("Value")) -> (s? t:f=w2935:T26)
                n1566 = property on="Auto-modulation" class="Bool (strict)"("Value"=w2931) -> ()  [unwired: 2 in, 2 out]
                "Running experiment" <- TRUE ("Running experiment")
              }
            }
            n1567 = Bundle By Name(cluster=w2909, "Remains"=w2901, "Experiment state"=w2907) -> (w2908:T25)
          }
          frame "Begin" {
            n1568 = Unbundle By Name(w2964) -> ("Auto-mod"=w2963:bool)
            n1569 = local read "Acquisition controls"() -> (w2966:T21)
            n1570 = Bundle By Name(cluster=w2966, "Auto-modulation"=w2963) -> (w2965:T21)
            n1571 = local write "Acquisition controls"(w2965) -> ()
          }
          frame "Acquisition" {
            n1572 = local read "New data"() -> (w2972:bool)
            n1573 = case shown="True" w2972 {
              selector: w2972 -> [_ w3021]
              tunnel: [FALSE w3033] -> w2980
              tunnel: w2973 -> [_ w3031]
              tunnel: w2971 -> [_ w3026]
              tunnel: w2970 -> [w2982 w3025]
              tunnel: [w2981 w3022] -> w2969
              frame False {
                n1574 = Unbundle By Name(w2982) -> ("Remains"=w2981:dbl)
              }
              frame True {
                n1575 = Not(x=w3021) -> (.not. x?=w3020:bool)
                n1576 = local read "data time"() -> (w3030:timestamp)
                n1577 = Unbundle By Name(w3025) -> ("Started"=w3024:timestamp)
                n1578 = local write "New data"(w3020) -> ()
                n1579 = Unbundle By Name(w3031) -> ("Start"=w3032:dbl, "End"=w3027:dbl)
                n1580 = local read "Data"() -> (w3028:dbl[])
                n1581 = To Double Precision Float(number=w3024) -> (double precision float=w3023:dbl)
                n1582 = To Double Precision Float(number=w3030) -> (double precision float=w3029:dbl)
                n1583 = Unbundle By Name(w3026) -> ("VTI.VTI [K]"=w2985:dbl, "VTI.Sample [K]"=w2999:dbl, "Magnet.Field [T]"=w2992:dbl, "Magnet.Ramp state"=w3001:T9, "Magnet.Ramp [mT/s]"=w2998:dbl)
                n1584 = Index Array(array=w3028) -> (element #1=w2991:dbl, element #2=w2990:dbl)  [unwired: 2 in]
                n1585 = Less?(x=w3032, y=w3027) -> (x < y?=w3004:bool)
                n1586 = Select(t=0.001 ("x"), s=w3004, f=-0.001) -> (s? t:f=w3006:dbl)
                n1587 = Subtract(x=w3029, y=w3023) -> (x-y=w3017:dbl)
                n1588 = Multiply(x=w3006, y=w2998) -> (x*y=w3009:dbl)
                n1589 = Multiply(x=w3017, y=w3009) -> (x*y=w3010:dbl)
                n1590 = Equal?(x=w3001, y=RampingOutput."At Target" ("Magnet.Ramp state")) -> (x = y?=w3002:bool)
                n1591 = Square(x=w2991) -> (x^2=w2988:dbl)
                n1592 = Square(x=w2990) -> (x^2=w2987:dbl)
                n1593 = Add(x=w3010, y=w3032) -> (x+y=w2995:dbl)
                n1594 = Subtract(x=w2995, y=w3027) -> (x-y=w2996:dbl)
                n1595 = local read "Acquisition controls"() -> (w3008:T21)
                n1596 = Add(x=w2988, y=w2987) -> (x+y=w2989:dbl)
                n1597 = Unbundle By Name(w3008) -> ("Modulation [A]"=w3007:dbl)
                n1598 = Absolute Value(x=w2996) -> (abs(x)=w2997:dbl)
                n1599 = Square Root(x=w2989) -> ()  [unwired: 1 out]
                n1600 = call "Is equal in tolerance.vi"("Absolut tolerance"=0.01, "Reference value"=w3027, "Input value"=w2992) -> ("Is in range"=w3019:bool)  [unwired: 1 in]
                n1601 = Divide(x=w2997, y=w2998) -> (x/y=w2994:dbl)
                n1602 = local read "Tab Control"() -> (w3016:T6)
                n1603 = And(x=w3002, y=w3019) -> (x .and. y?=w3033:bool)
                n1604 = call "Add point to array for XY graph.vi"("X-axis"=w2995, "Input A"=w2991, "Input B"=w2990) -> ("Array"=w3012:cluster{"Array":dbl[], "Array":dbl[]}[])  [unwired: 4 in]
                n1605 = local read "SMU controls"() -> (w2986:T14)
                n1606 = Unbundle By Name(w2986) -> ("B[T]"=w2984:dbl)
                n1607 = case shown="\"EPR measurement\"" w3016 {
                  tunnel: w3012 -> [_ w3034]
                  frame "Page Status", Default {
                  }
                  frame "EPR measurement" {
                    "Spectrum" <- w3034
                  }
                }
                n1608 = local read "meas results"() -> (w3011:refnum<file>)
                n1609 = Build Array(w2995, w2984, w2991, w2990, w2999, w2985, w3007, w2992) -> (w3014:dbl[])
                n1610 = Multiply(x=w2994, y=1000.0) -> (x*y=w3022:dbl)
                n1611 = Array To Spreadsheet String(array=w3014, 3:"%e" ("format string")) -> (spreadsheet string=w3013:string)  [unwired: 1 in]
                n1612 = Write to Text File(file (use dialog)=w3011, text=w3013) -> ()  [unwired: 2 in, 3 out]
              }
            }
            n1613 = Select(t=experiment_state."Save" ("Value"), s=w2980, f=experiment_state."Acquisition" ("Value")) -> (s? t:f=w2974:T26)
            n1614 = Bundle By Name(cluster=w2976, "Experiment state"=w2974, "Remains"=w2969) -> (w2975:T25)
          }
          frame "Save" {
            n1615 = local read "THz control"() -> (w3040:T22)
            n1616 = property on="Script Array" class="Arr (strict)"() -> ("Selection Start []"=w3047:u32[])  [unwired: 2 in, 2 out]
            n1617 = local read "Script Array"() -> (w3063:T27[])
            n1618 = local read "Infobar"() -> (w3051:T25)
            n1619 = local read "Instr status"() -> (w3057:T1)
            n1620 = Index Array(array=w3047) -> (element=w3048:u32)  [unwired: 1 in]
            n1621 = Unbundle By Name(w3040) -> ("AMC"=w3038:u16, "Multip"=w3039:u16)
            n1622 = Increment(x=w3048) -> (x+1=w3060:u32)
            n1623 = Array Size(array=w3063) -> (size(s)=w3061:i32)
            n1624 = local read "Run script btn"() -> (w3055:bool)
            n1625 = Multiply(x=w3038, y=w3039) -> (x*y=w3037:u16)
            n1626 = Array Subset(array=w3063, index=w3060) -> (w3058:T27[])  [unwired: 1 in]
            n1627 = for {
              tunnel: [w3106] -> w3056
              tunnel: w3057 -> [w3108]
              tunnel: [w3107] -> w3053
              tunnel: w3058 -> [w3106] mode=indexing
              tunnel: [w3105] -> w3059
              tunnel: w3037 -> [w3104]
              i -> [w3105]
              stop <- w3107 stop-if-true
              n1628 = call "verify executabiity of line.vi"("Freq multiplication factor"=w3104, "Instr status"=w3108, "Script cluster"=w3106) -> ("is executable"=w3107:bool)  [unwired: 7 in, 1 out]
            }
            n1629 = Greater?(x=w3061, y=w3048) -> (0:w3054:bool)
            n1630 = Compound Arithmetic op=AND(w3055, w3054, w3053) -> (w3052:bool)
            n1631 = Add(x=w3059, y=w3060) -> (x+y=w3050:u32)
            n1632 = local write "Run script btn"(w3052) -> ()
            n1633 = case shown="False" w3052 {
              tunnel: [experiment_state."Setup" ("Value") experiment_state."Preparation" ("Value")] -> w3064
              tunnel: w3049 -> [w3113 _]
              tunnel: w3063 -> [_ _]
              tunnel: [w3113 w3116] -> w3062
              tunnel: w3048 -> [w3110 _]
              tunnel: w3056 -> [_ w3116]
              tunnel: w3051 -> [_ _]
              tunnel: w3050 -> [_ w3115]
              tunnel: [w3110 w3115] -> w3041
              frame False {
                n1634 = local read "Controls referencies"() -> (w3112:T2)
                n1635 = Unbundle By Name(w3112) -> ("To disable"=w3109:refnum<vi>[])
                n1636 = call "Dis- or en- able controls.vi"("Disabled"=T34."Enabled", "Control referencies"=w3109) -> ()  [unwired: 9 in, 1 out]
              }
              frame True {
              }
            }
            n1637 = call "Add point to array for XY graph.vi"("Write?(T)"=FALSE ("Write(T)")) -> ("Array"=w3035:cluster{"Array":dbl[], "Array":dbl[]}[])  [unwired: 6 in]
            n1638 = local write "Spectrum"(w3035) -> ()
            n1639 = local read "meas results"() -> (w3071:refnum<file>)
            n1640 = Close File(refnum=w3071) -> (path=w3044:path)  [unwired: 1 in, 1 out]
            n1641 = case shown="True" "Save also backup" {
              tunnel: w3044 -> [_ w3097]
              tunnel: w3035 -> [_ w3072]
              frame False {
              }
              frame True {
                w3081 = "\t"
                n1642 = Strip Path(path=w3097) -> (stripped path=w3093:path, name=w3096:string)
                n1643 = Concatenate Strings("Backup_", w3096) -> (w3094:string)
                n1644 = Build Path(base path=w3093, name or relative path=w3094) -> (appended path=w3092:path)
                n1645 = Index Array(array=w3072, index #1=0 ("index"), index #2=1 ("index")) -> (element #1=w3088:cluster{"Array":dbl[], "Array":dbl[]}, element #2=w3091:cluster{"Array":dbl[], "Array":dbl[]})
                n1646 = call <vilib>:"Create File with Incrementing Suffix.vi"("file path"=w3092) -> ("error out"=w3073:errorcluster, "refnum out"=w3076:refnum<file>)  [unwired: 8 in, 1 out]
                n1647 = Concatenate Strings("B[T]" ("string"), w3081, "X" ("string"), w3081, "Y", "\r\n") -> (w3078:string)
                n1648 = Unbundle(w3088) -> ("Array"=w3087:dbl[], "Array"=w3086:dbl[])
                n1649 = Unbundle(w3091) -> ("Array"=w3085:dbl[])  [unwired: 1 out]
                n1650 = for {
                  tunnel: w3087 -> [w3099] mode=indexing
                  tunnel: w3086 -> [w3101] mode=indexing
                  tunnel: w3085 -> [w3100] mode=indexing
                  tunnel: [w3102] -> w3079 mode=indexing
                  n1651 = Build Array(w3099, w3101, w3100) -> (w3098:dbl[])
                  n1652 = Array To Spreadsheet String(array=w3098, 3:"%g" ("format string")) -> (spreadsheet string=w3102:string)  [unwired: 1 in]
                }
                n1653 = Concatenate Strings(w3078, w3079) -> (w3077:string)
                n1654 = Write to Text File(file (use dialog)=w3076, text=w3077, error in=w3073) -> (refnum out=w3074:refnum<file>, error out=w3075:errorcluster)  [unwired: 1 in, 1 out]
                n1655 = Close File(refnum=w3074, error in=w3075) -> ()  [unwired: 2 out]
              }
            }
            n1656 = Build Array(w3041) -> (w3042:u32[])
            n1657 = Bundle By Name(cluster=w3066, "Experiment state"=w3064) -> (w3065:T25)
            n1658 = Path To String(path=w3044) -> (string=w3043:string)
            n1659 = property on="Script Array" class="Arr (strict)"("Selection Start []"=w3042) -> ()  [unwired: 2 in, 2 out]
            n1660 = Concatenate Strings("Measurrement finished " ("String in"), w3043) -> (w3045:string)
            n1661 = call "Add actual date time to string.vi"("String in"=w3045) -> ("String out"=w3070:string)  [unwired: 4 in]
            n1662 = call "simple Shift string array.vi"("Element in"=w3070, "Array in"=w3068) -> ("Array out"=w3067:string[])  [unwired: 8 in, 1 out]
          }
        }
      }
      frame "Stop" {
        n1663 = call "simple Shift string array.vi"("Element in"="Program stopped", "Array in"=w3123) -> ("Array out"=w3122:string[])  [unwired: 8 in, 1 out]
      }
      frame "Restart" {
        n1664 = Build Array("Program restarted") -> (w3128:string[])
      }
    }
    n1665 = Tick Count (ms)() -> (millisecond timer value=w20:u32)
    n1666 = Subtract(x=w20, y=w19) -> (x-y=→"round execution\ntime [ms]":u32)
  }
  n1667 = case shown="True" "Debug mode?" {
    tunnel: w10 -> [w3141 w3149]
    frame True {
      w3134 = u32 0 items=["1", "2", "3"] ("axis (0)")
      n1668 = Unbundle By Name(w3141) -> ("Mod_M"=w3133:refnum<queue>, "Field_C"=w3136:refnum<queue>, "MW_C"=w3138:refnum<queue>, "Angle_C"=w3139:refnum<queue>, "Table_C"=w3140:refnum<queue>, "Data_Aq"=w3135:refnum<queue>, "Tmp_C"=w3137:refnum<queue>, "TOP"=w3131:refnum<queue>)
      n1669 = call "TemperatureController main.vi"("Supervising module"=w3131, "Controller module"=w3137) -> ()  [unwired: 10 in]
      n1670 = call "MFLI module main.vi"("Master mailbox"=w3131, "Module mailbox"=w3135) -> ()  [unwired: 10 in]
      n1671 = call "Servo main.vi"("Queue to UI"=w3131, "Module queue servo"=w3140) -> ()  [unwired: 10 in]
      n1672 = call "SampleRotator main.vi"("axis (0)"=w3134, "Top"=w3131, "Rotator"=w3139) -> ()  [unwired: 8 in, 1 out]
      n1673 = call "Module for APVSG.vi"("Main controller mailbox"=w3131, "THz module mailbox"=w3138) -> ()  [unwired: 8 in, 2 out]
      n1674 = call "MagnetTop.vi"("Queue to UI"=w3131, "Module queue"=w3136) -> ()  [unwired: 10 in]
      n1675 = call "SMU magnetic field meter.vi"("update time (100ms)"=u32 100, "Mailbox address Top"=w3131, "Module mailbox"=w3133) -> ()  [unwired: 7 in, 2 out]
    }
    frame False {
      n1676 = Unbundle By Name(w3149) -> ("Instr_M"=w3144:refnum<queue>, "Tmp_M"=w3146:refnum<queue>, "MW_C"=w3147:refnum<queue>, "Table_C"=w3148:refnum<queue>, "Tmp_C"=w3143:refnum<queue>, "Field_C"=w3145:refnum<queue>, "TOP"=w3142:refnum<queue>)
      n1677 = call "Fake VTI module.vi"("Top address in"=w3142, "VTI Module ref"=w3145) -> ()  [unwired: 10 in]
      n1678 = call "fake lock-in module.vi"("Master mailbox"=w3142, "Module mailbox"=w3143) -> ()  [unwired: 10 in]
      n1679 = call "fake Servo modue.vi"("Queue to UI"=w3142, "Module queue servo"=w3148) -> ()  [unwired: 10 in]
      n1680 = call "fake SampleRotator module.vi"("Top"=w3142, "Rotator"=w3147) -> ()  [unwired: 8 in, 2 out]
      n1681 = call "fake THz module.vi"("Main controller mailbox"=w3142, "THz module mailbox"=w3146) -> ()  [unwired: 10 in]
      n1682 = call "fake main magnet module.vi"("Queue to UI"=w3142, "Module queue"=w3144) -> ()  [unwired: 10 in]
    }
  }
  n1683 = flat-sequence {
    tunnel: w5 -> [_]
    frame #0 {
      n1684 = Stop(stop? (T)=TRUE) -> ()
    }
  }
